vi "Labview.vi"() -> ()   [LabVIEW 2021]
uses:
  <vilib>/userdefined/High Color/IMAQdx.ctl
  <vilib>/Instr/_visa.llb/VISA Configure Serial Port (Instr).vi
  <vilib>/Utility/cursorutil.llb/Set Cursor (Icon Pict).vi
  <vilib>/Utility/file.llb/Write Delimited Spreadsheet (string).vi
  <vilib>/addons/VIRobotics/onnx/Session/Get_Result_float.vi
  <vilib>/vision/driver/NI_Vision_Acquisition_Software.lvlib
  <vilib>/vision/NI_Vision_Development_Module.lvlib
  <vilib>/addons/VIRobotics/onnx/Session/Session.lvclass
panel:
  out "String 2":string
  out "Tab Control":T1(tab)
  in  "Ga2 6":string="908"
  out "Sub1 3":string
  out "MSE loss":string
  in  "Is the probability of the model output deoxidization exceeding":bool
  out "Obtain Growth Temperature":bool
  out "From (2×4) to (n×6)":string
  out "From c(4×4) to (2×4)":string
  out "From As cap to c(4×4)":string
  out "Substrate to find Reconstruction temperature":string
  out "Cool to less than 100 ℃ and wait 20 minutes":bool
  out "GaAs buffer 0.6 μm/h":bool
  in  "nm 3":u32=100
  in  "Ga2 5":string="908"
  out "Sub1 2":string
  out "Heating to completely remove oxidation":bool
  out "Deoxidation temperature":string
  out "Substrate to find Deoxidation temperature":string
  out "Obtaining the reconstruction  temperature":bool
  out "Obtaining the deoxidation temperature":bool
  in  "Start":bool
  in  "Ga2 1":string="908"
  out "Ready for GaAs buffer 0.6 μm/h":bool
  out "GaAs buffer 0.6 μm/h":bool
  out "Sub1":string
  in  "nm":u32=100
  out "Reconstruction模型输出结果":string
  out "InAs growth temperature":string
  out "GaAs growth temperature":string
  out "C =":string
  out "B =":string
  out "A =":string
  in  "Is the probability of the model output c(4×4) exceeding":bool
  in  "Is the probability of the model output (2×4) exceeding":bool
  in  "Is the probability of the model output (n×6) exceeding":bool
  out "Surface InAs QDs for AFM":bool
  out "If In Shutter can be closed 1":bool
  out "Inside InAs QDs":bool
  out "10 nm GaAs cap layer 0.36 μm/h":bool
  out "GaAs buffer 0.6 μm/h  2":bool
  in  "Surface InAs QDs":bool=TRUE
  in  "Cooling":bool=TRUE
  in  "Sub5":string="150"
  out "Sub2":string
  in  "Ga2 2":string="888"
  out "Sub3":string
  in  "Ga2 3":string="908"
  out "Sub4":string
  in  "Ga2 4":string="800"
  out "Temperature adjustment 1":bool
  out "Temperature adjustment 2":bool
  out "Temperature adjustment 3":bool
  out "Optimize Sub Temperature 1":string
  out "Optimize Sub Temperature 2":string
  out "If In Shutter can be closed 2":bool
  in  "nm 2":u32=100
  out "Shutter模型输出结果":string
  out "Temperature模型输出结果 2":string
  in  "模型输出是否超过0.7概率是Ys":bool
  in  "Tab Control 3":enum32{"RHEED", "Array1", "Array2"}(tab)
  out "主界面 1":T2(plugin-control)
  in  "摄像头选择":T3 caption="摄像头开关"
  in  "摄像头开关":bool
  out "Countdow":u16
  out "Reminder Information":string
  in  "Model switch":bool
  in  "Whether to continue heat up for reconstruction":bool
  in  "While loop for cool to less than 100 ℃":bool
  in  "Is the probability of the model output oxidization exceeding":bool
  out "2 (2×4) count":u8
  out "5 (n×6) count":i32
  out "1 c(4×4) count":i32
  out "3 Oxidization count":u8
  out "4 Deoxidization count":u8
  out "0 As cap count":u8
  out "2 (2×4) number":u8
  out "5 (n×6) number":i32
  out "1 c(4×4) number":i32
  out "3 Oxidization number":u8
  out "4 Deoxidization number":u8
  out "0 As cap number":u8
  out "Reconstruction模型输出结果":sgl[](array[numeric])
  out "记录Reconstruction模型的连续24个输出结果":u8[](array[numeric])
  in  "T":i32=24
  in  "repetition 1 LT-GaAs not do":bool
  in  "10 nm LT-GaAs switch Yes is do":bool=TRUE
  out "Shutter count Yes":u8
  out "Shutter count No":u8
  out "Growth Switch":i32
  out "多张图片拼接后的多维数组":dbl[][][](array[numeric])
  out "用于存储单站图片转换后的单通道矩阵":dbl[][](array[numeric])
  out "经过python转换后的数组":dbl[][][][](array[numeric])
  out "error out 6":errorcluster
  in  "选择多少张图片（通道）":i32=24
  in  "转换给模型的像素长宽大小":i32=128
  out "记录Shutter模型的连续24个输出结果":u8[](array[numeric])
  out "0 Growth真空度（字符串）":string
  out "0 Buffer真空度(字符串)":string
  out "Temperature Switch":i32
  out "Shutter模型输出结果 2":sgl[](array[numeric])
  out "Temperature模型输出结果":sgl[](array[numeric])
  out "记录Temperature模型的连续24个输出结果":u8[](array[numeric])
  out "倒计时开关":bool
  out "Temperature count High":u8
  out "Temperature count Low":u8
  out "Temperature count Suitable":u8
  out "Temperature count result":u8
  out "Shutter count Yes result":u8
  in  "Yes prop":dbl=0.7 format="%#_13g"
  in  "Tetragon":cluster{"x":sgl, "y":sgl}[](array[cluster])=[{"x"=659.0, "y"=217.0}, {"x"=1148.0, "y"=217.0}, {"x"=1148.0, "y"=706.0}, {"x"=659.0, "y"=706.0}]
  in  "dimension size":i32=24
  in  "Suitable prop":dbl=0.4 format="%#_13g"
  in  "repeats of InAs/GaAs":i32=1
  in  "Is the probability of the model output As cap exceeding":bool
  in  "Reconstruction probability":dbl=0.8 format="%#_13g"
  in  "Repetition":i32
  in  "Whether to continue heating up operation":bool
  out "主界面 2":T2(plugin-control)
  in  "?":enum32{"Status"}(tab)
  out "Sub程序":string
  in  "Sub速度":string="10"
  in  "Sub设定":string="150" caption="0 Sub设定"
  out "Sub实测":string
  out "Buffer vacuum":dbl format="%.2e"
  out "Growth vacuum":dbl format="%.2e"
  in  "As挡板":bool=TRUE
  in  "In挡板":bool
  in  "Ga2挡板":bool
  in  "Main挡板":bool=TRUE
  out "Ga2实测":string
  in  "Ga2设定":string="400" caption="0 Sub设定"
  in  "Ga2速度":string="6"
  out "Ga2程序":string
  out "In实测":string
  in  "In设定":string="350" caption="0 Sub设定"
  in  "In速度":string="6"
  out "In程序":string
  # "Sub"
  # "Deoxidation temperature"
  # "Sub"
  # "Ga2"
  # "nm"
  # "Sub"
  # "Ga2"
  # "Sub"
  # "From As cap to c(4×4)"
  # "From c(4×4) to (2×4)"
  # "From (2×4) to (n×6)"
  # "Ax^2 + bx + c = 0"
  # "Sub"
  # "Ga2"
  # "nm"
  # "Sub"
  # "Ga2"
  # "Sub"
  # "Ga2"
  # "nm"
  # "Sub"
  # "Ga2"
  # "Sub"
  # "Measured temperature"
  # "Programmed\ntemperature"
  # "Setting\n(℃)"
  # "Rate\n(℃/min)"
  # "Shutter"
  # "Sub"
  # "Ga2"
  # "In"
  # "As"
  # "The As cracker’s needle valve is adjusted manually"
types:
  T1 = enum32{"Growth Temperature Initialization", "InAs/GaAs QDs on GaAs substrates"}
  T2 = typedef "IMAQ Image.ctl" = refnum<image>
  T3 = typedef "IMAQdx.ctl" = refnum<k21>
  T4 = enum8{"Enabled", "Disabled", "Disabled and Grayed Out"}
  T5 = typedef "Image Type" = u32
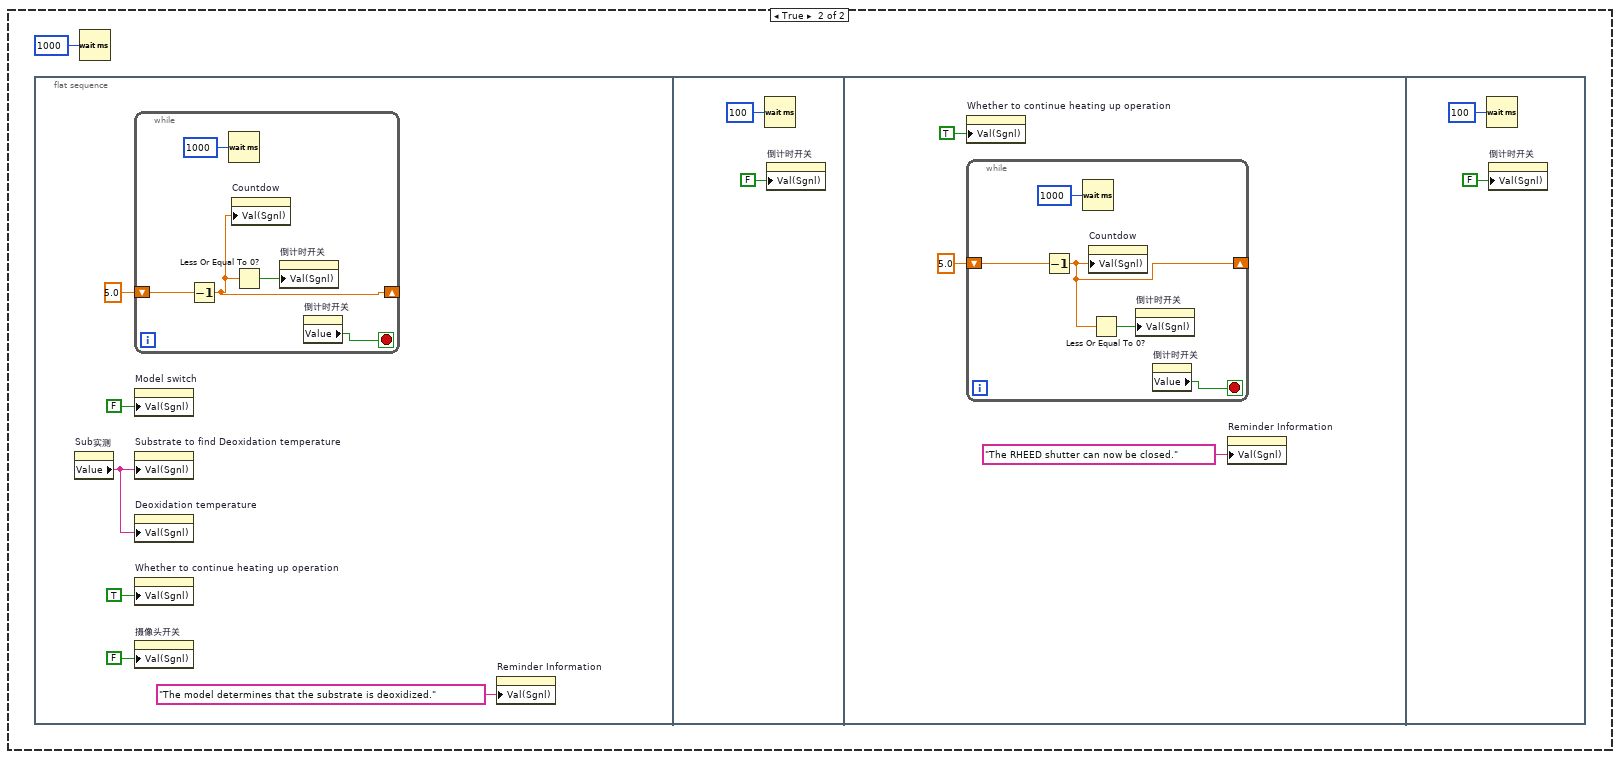
[diagram p4: hidden frame]
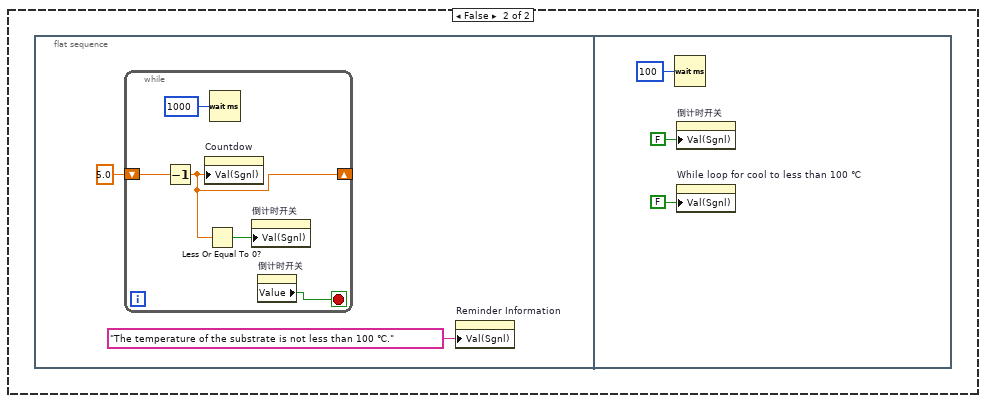
[diagram p6: hidden frame]
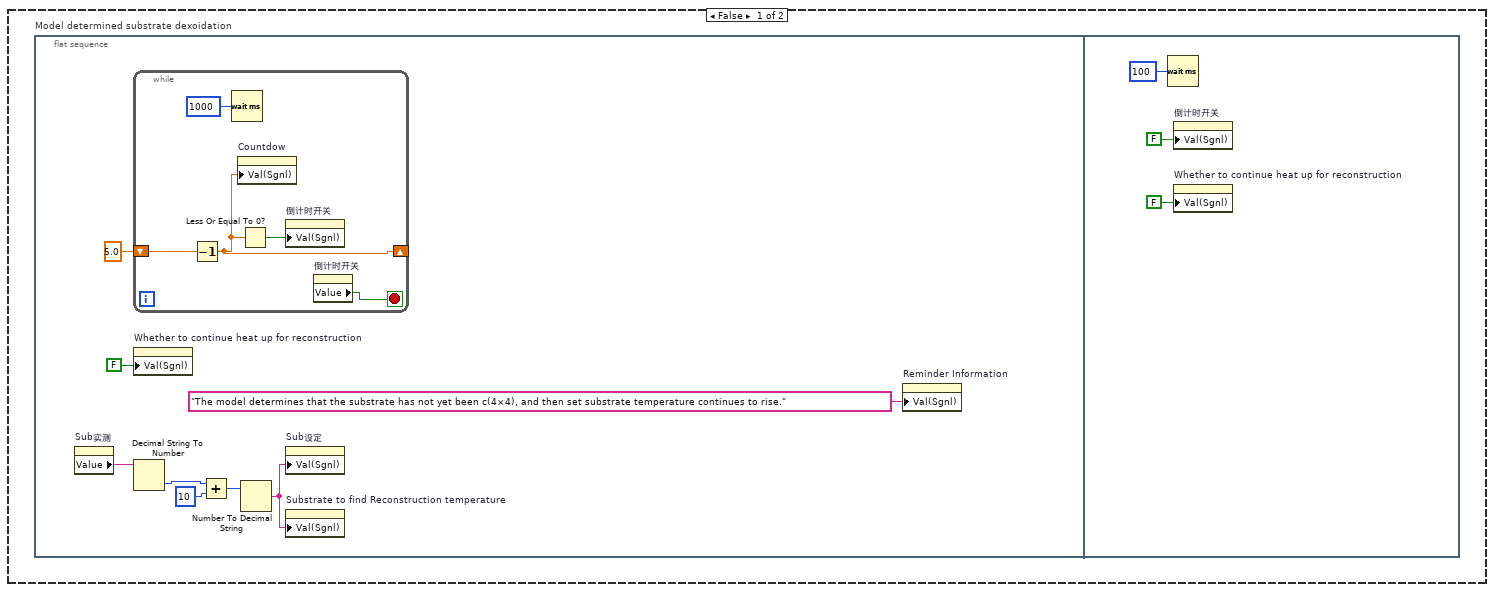
[diagram p9: hidden frame]
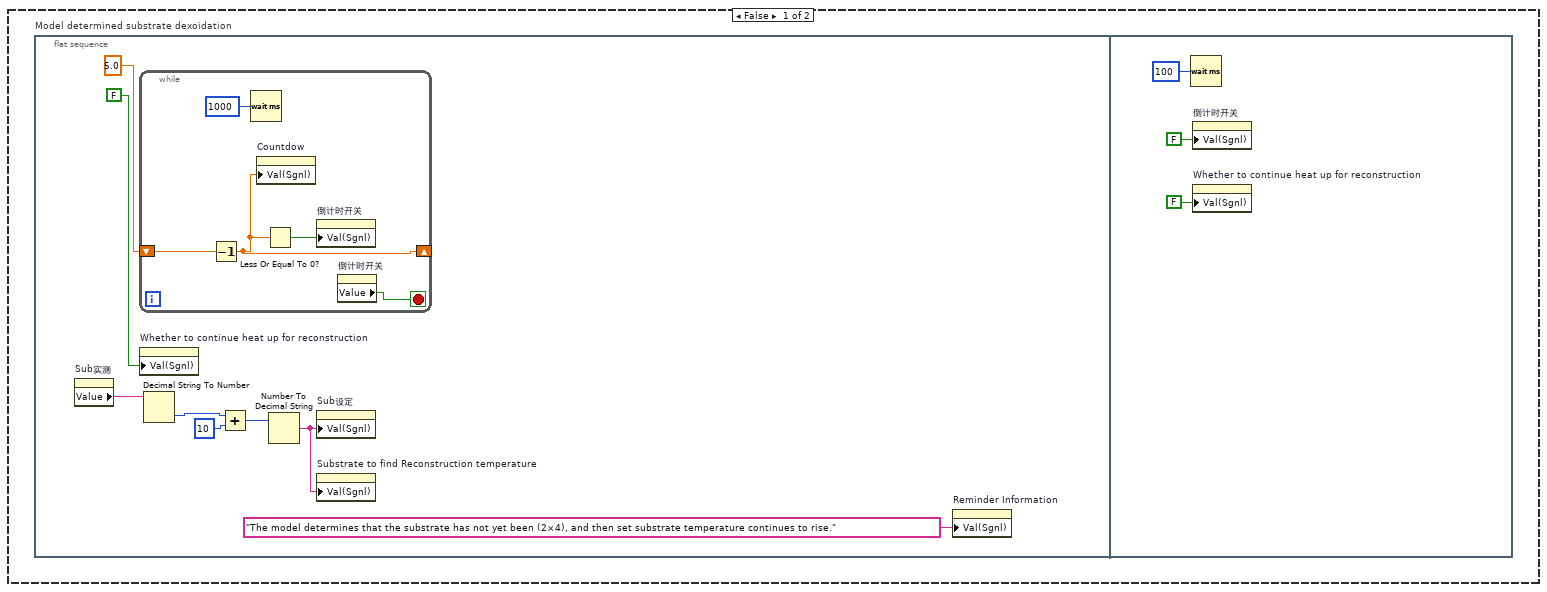
[diagram p11: hidden frame]
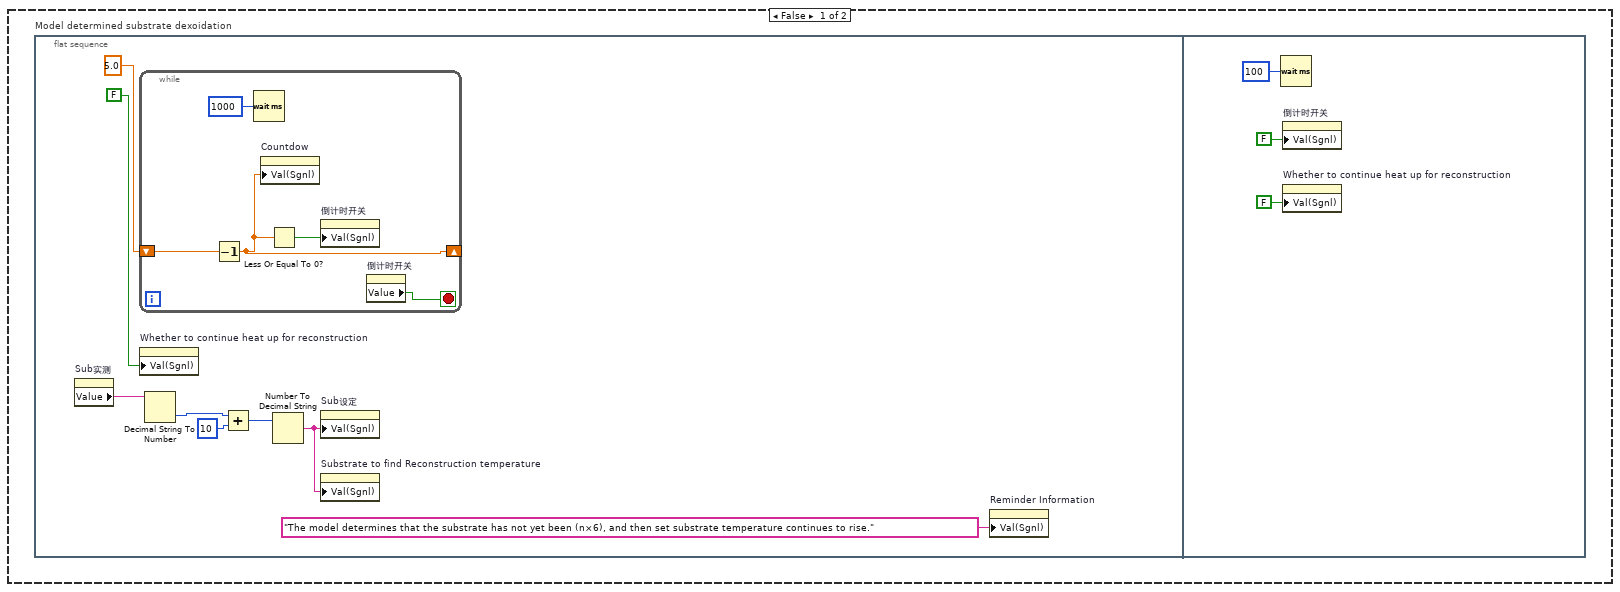
[diagram p13: hidden frame]
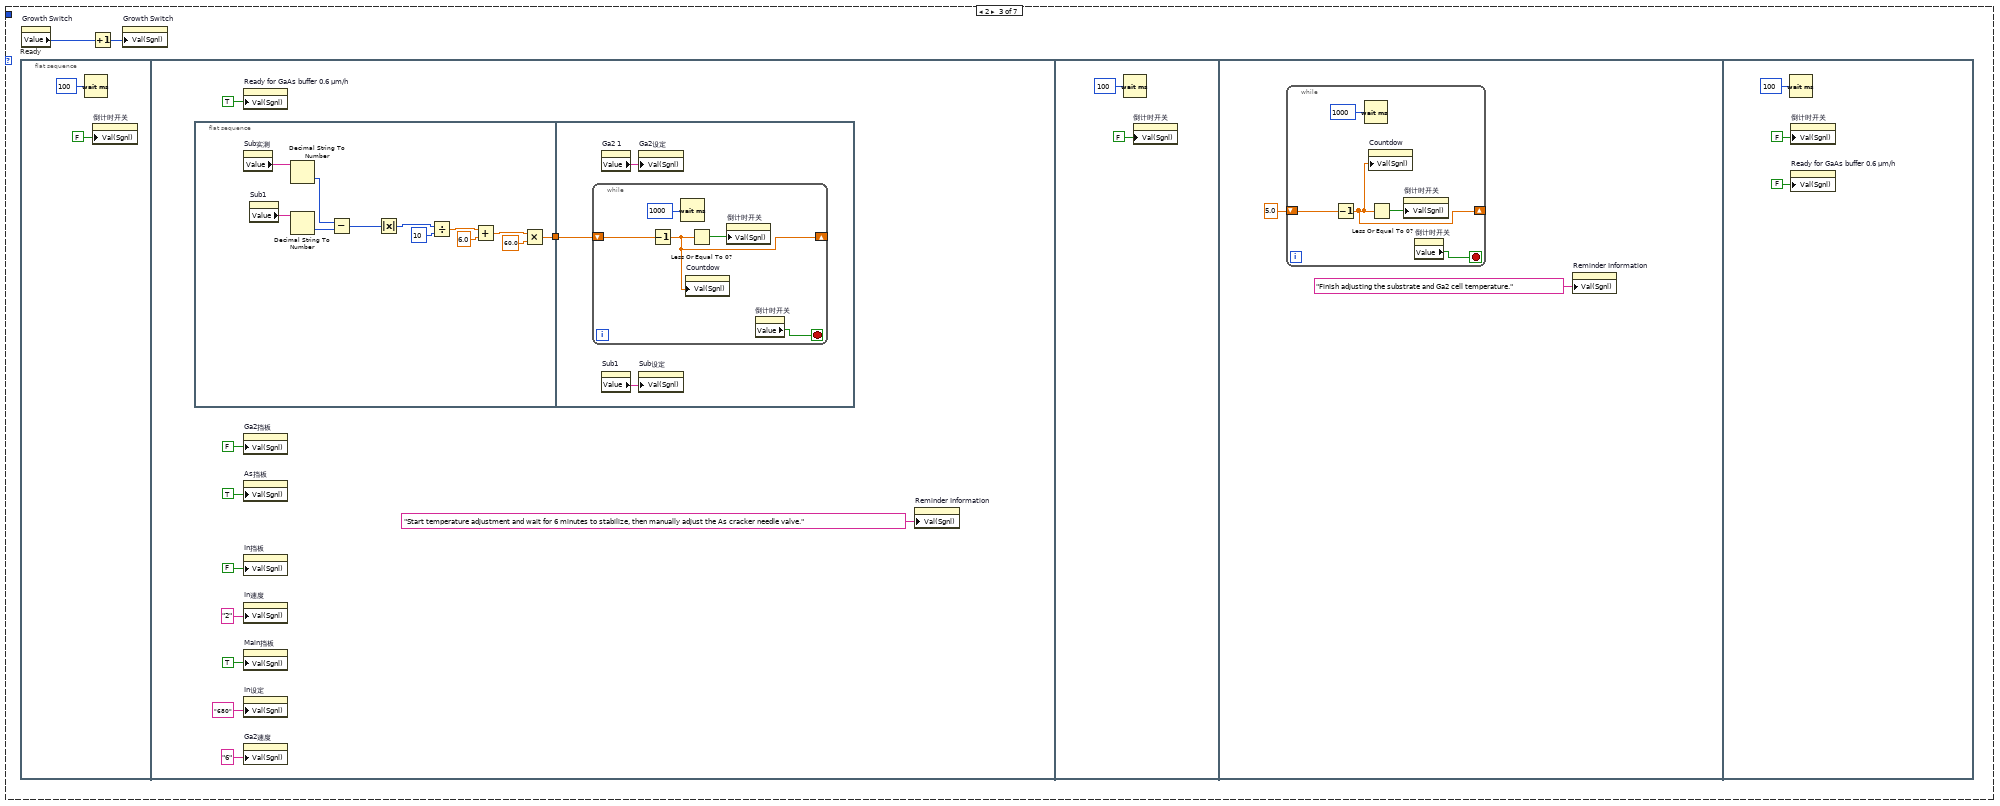
[diagram p15: hidden frame]
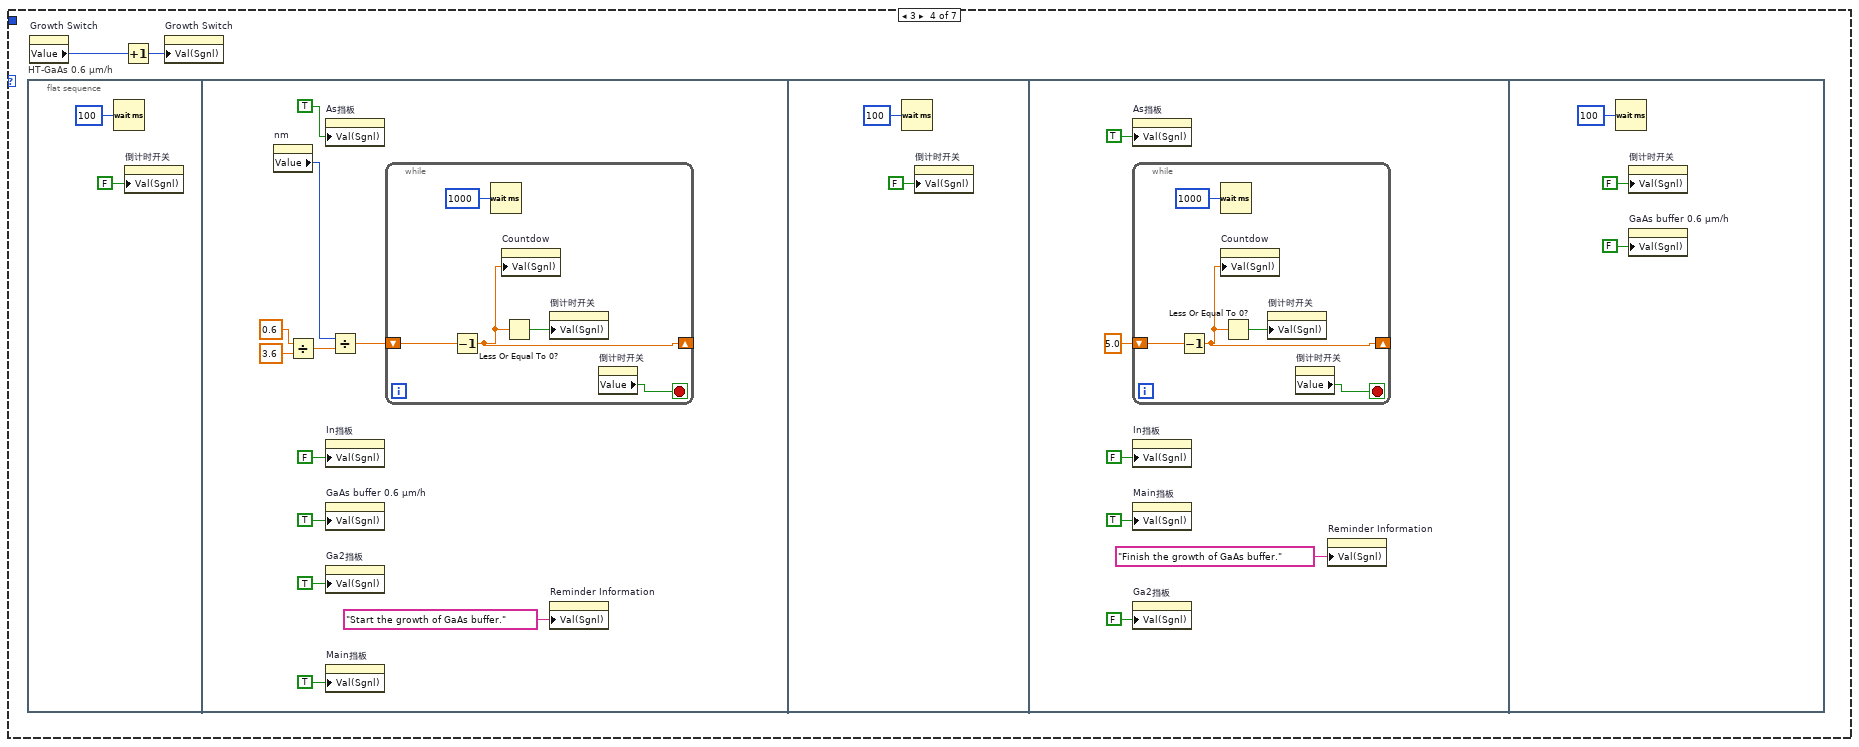
[diagram p16: hidden frame]
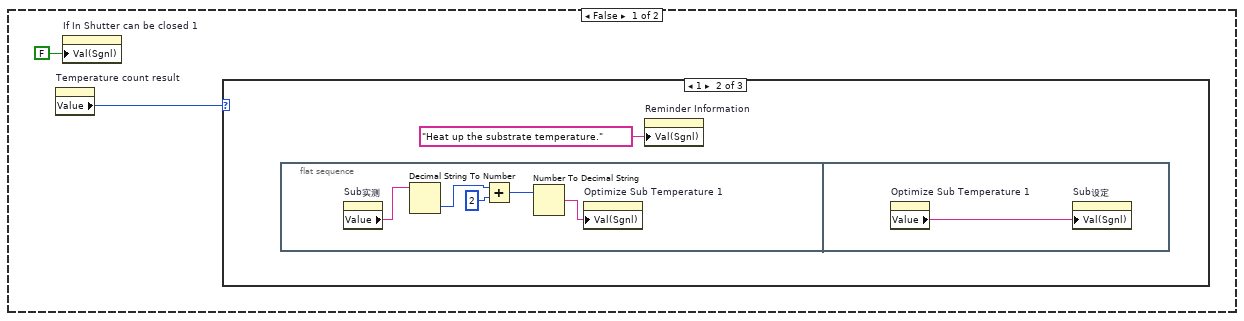
[diagram p17: hidden frame]
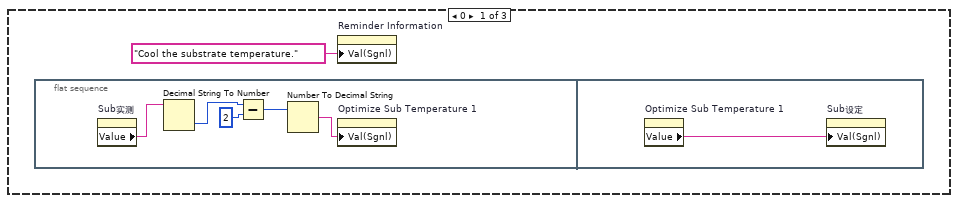
[diagram p18: hidden frame]
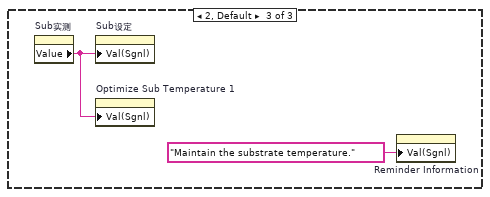
[diagram p19: hidden frame]
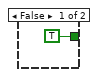
[diagram p20: hidden frame]
diagram:
  w71 = u16 10 items=["1.0"=10, "1.5"=15, "2.0"=20] ("stop bits (10: 1 bit)")
  w82 = u16 20 items=["1.0"=10, "1.5"=15, "2.0"=20] ("stop bits (10: 1 bit)")
  n1 = while {
    stop <- FALSE stop-if-true
    w91 = refnum<visa-resource-name> "COM9"  # Temperature I/O
    n2 = property on="Temperature Switch" class="DigNum (strict)"() -> ("Value"=w92:i32)  [unwired: 2 in, 2 out]
    n3 = case shown="1" w92 {
      tunnel: w91 -> [w97 w111 w124]
      frame 1 {
        n4 = flat-sequence {
          tunnel: w97 -> [w101]
          tunnel: [w101] -> w96
          tunnel: w96 -> [w103]
          tunnel: [w103] -> w95
          tunnel: w95 -> [w105]
          tunnel: [w105] -> w94
          tunnel: w94 -> [w107]
          frame #0 {
            n5 = call "Ga R.vi"("VISA resource name"=w101) -> ("程序温度"=w100:string)  [unwired: 10 in]
            n6 = property on="Ga2程序" class="Str"("Val(Sgnl)"=w100) -> ()  [unwired: 2 in, 2 out]
          }
          frame #1 {
            n7 = call "Ga P.vi"("VISA resource name"=w103) -> ("实测温度"=w102:string)  [unwired: 10 in]
            n8 = property on="Ga2实测" class="Str"("Val(Sgnl)"=w102) -> ()  [unwired: 2 in, 2 out]
          }
          frame #2 {
            n9 = property on="Ga2设定" class="Str"() -> ("Value"=w104:string)  [unwired: 2 in, 2 out]
            n10 = call "Ga S.vi"("VISA resource name 2"=w105, "设定温度"=w104) -> ()  [unwired: 10 in]
          }
          frame #3 {
            n11 = property on="Ga2速度" class="Str"() -> ("Value"=w106:string)  [unwired: 2 in, 2 out]
            n12 = call "Ga V.vi"("VISA resource name"=w107, "升温速度"=w106) -> ()  [unwired: 10 in]
          }
        }
        n13 = property on="Temperature Switch" class="DigNum (strict)"() -> ("Value"=w98:i32)  [unwired: 2 in, 2 out]
        n14 = Increment(x=w98) -> (x+1=w99:i32)
        n15 = property on="Temperature Switch" class="DigNum (strict)"("Val(Sgnl)"=w99) -> ()  [unwired: 2 in, 2 out]
      }
      frame 2 {
        n16 = flat-sequence {
          tunnel: w111 -> [w114]
          tunnel: [w114] -> w110
          tunnel: w110 -> [w116]
          tunnel: [w116] -> w109
          tunnel: w109 -> [w118]
          tunnel: [w118] -> w108
          tunnel: w108 -> [w120]
          frame #0 {
            n17 = call "In R.vi"("VISA resource name"=w114) -> ("程序温度"=w113:string)  [unwired: 10 in]
            n18 = property on="In程序" class="Str"("Val(Sgnl)"=w113) -> ()  [unwired: 2 in, 2 out]
          }
          frame #1 {
            n19 = call "In P.vi"("VISA resource name"=w116) -> ("实测温度"=w115:string)  [unwired: 10 in]
            n20 = property on="In实测" class="Str"("Val(Sgnl)"=w115) -> ()  [unwired: 2 in, 2 out]
          }
          frame #2 {
            n21 = property on="In设定" class="Str"() -> ("Value"=w117:string)  [unwired: 2 in, 2 out]
            n22 = call "In S.vi"("VISA resource name 2"=w118, "设定温度"=w117) -> ()  [unwired: 10 in]
          }
          frame #3 {
            n23 = property on="In速度" class="Str"() -> ("Value"=w119:string)  [unwired: 2 in, 2 out]
            n24 = call "In V.vi"("VISA resource name"=w120, "升温速度"=w119) -> ()  [unwired: 10 in]
          }
        }
        n25 = property on="Temperature Switch" class="DigNum (strict)"("Val(Sgnl)"=0 ("Value (Signaling)")) -> ()  [unwired: 2 in, 2 out]
      }
      frame 0, Default {
        n26 = flat-sequence {
          tunnel: w124 -> [w128]
          tunnel: [w128] -> w123
          tunnel: w123 -> [w130]
          tunnel: [w130] -> w122
          tunnel: w122 -> [w131]
          tunnel: [w131] -> w121
          tunnel: w121 -> [w133]
          frame #0 {
            n27 = call "Sub R.vi"("VISA resource name"=w128) -> ("程序温度"=w127:string)  [unwired: 10 in]
            n28 = property on="Sub程序" class="Str"("Val(Sgnl)"=w127) -> ()  [unwired: 2 in, 2 out]
          }
          frame #1 {
            n29 = call "Sub P.vi"("VISA resource name"=w130) -> ("实测温度"=w129:string)  [unwired: 10 in]
            n30 = property on="Sub实测" class="Str"("Val(Sgnl)"=w129) -> ()  [unwired: 2 in, 2 out]
          }
          frame #2 {
            n31 = property on="Sub设定" class="Str"() -> ("Value"=w132:string)  [unwired: 2 in, 2 out]
            n32 = call "Sub S.vi"("VISA resource name 2"=w131, "设定温度"=w132) -> ()  [unwired: 10 in]
          }
          frame #3 {
            n33 = property on="Sub速度" class="Str"() -> ("Value"=w134:string)  [unwired: 2 in, 2 out]
            n34 = call "Sub V.vi"("VISA resource name"=w133, "升温速度"=w134) -> ()  [unwired: 10 in]
          }
        }
        n35 = property on="Temperature Switch" class="DigNum (strict)"() -> ("Value"=w125:i32)  [unwired: 2 in, 2 out]
        n36 = Increment(x=w125) -> (x+1=w126:i32)
        n37 = property on="Temperature Switch" class="DigNum (strict)"("Val(Sgnl)"=w126) -> ()  [unwired: 2 in, 2 out]
      }
    }
  }
  n38 = flat-sequence {
    frame #0 {
      n39 = Wait (ms)(milliseconds to wait=u32 1000) -> ()  [unwired: 1 out]
    }
    frame #1 {
      n40 = while {
        stop <- FALSE stop-if-true
        n41 = property on="Start" class="Bool (strict)"() -> ("Value"=w136:bool)  [unwired: 2 in, 2 out]
        n42 = case shown="True" w136 {
          frame False {
          }
          frame True {
            n43 = property on="repeats of InAs/GaAs" class="DigNum (strict)"() -> ("Value"=w139:i32)  [unwired: 2 in, 2 out]
            n44 = property on="Growth Switch" class="DigNum (strict)"() -> ("Value"=w138:i32)  [unwired: 2 in, 2 out]
            n45 = case shown="4" w138 {
              tunnel: w139 -> [_ _ _ _ w802 _ _]
              frame 0, Default {
                n46 = flat-sequence {
                  frame #0 {
                    n47 = flat-sequence "Achieving the deoxidation temperature" {
                      frame #0 {
                        n48 = Wait (ms)(milliseconds to wait=u32 100) -> ()  [unwired: 1 out]
                        n49 = property on="倒计时开关" class="Bool (strict)"("Val(Sgnl)"=FALSE ("Value (Signaling)")) -> ()  [unwired: 2 in, 2 out]
                      }
                      frame #1 {
                        w145 = "390" ("Value (Signaling)")
                        n50 = property on="As挡板" class="Bool (strict)"("Val(Sgnl)"=TRUE ("Value (Signaling)")) -> ()  [unwired: 2 in, 2 out]
                        n51 = while {
                          shift-right: [w154] -> _
                          shift-left: 5.0 -> [w156]
                          stop <- w155 stop-if-true
                          n52 = Decrement(x=w156) -> (x-1=w154:dbl)
                          n53 = Wait (ms)(milliseconds to wait=u32 1000) -> ()  [unwired: 1 out]
                          n54 = property on="Countdow" class="DigNum (strict)"("Val(Sgnl)"=w154) -> ()  [unwired: 2 in, 2 out]
                          n55 = Less Or Equal To 0?(x=w154) -> (x <= 0?=w153:bool)
                          n56 = property on="倒计时开关" class="Bool (strict)"("Val(Sgnl)"=w153) -> ()  [unwired: 2 in, 2 out]
                          n57 = property on="倒计时开关" class="Bool (strict)"() -> ("Value"=w155:bool)  [unwired: 2 in, 2 out]
                        }
                        n58 = property on="Ga2挡板" class="Bool (strict)"("Val(Sgnl)"=FALSE ("Value (Signaling)")) -> ()  [unwired: 2 in, 2 out]
                        n59 = property on="Sub设定" class="Str"("Val(Sgnl)"=w145) -> ()  [unwired: 2 in, 2 out]
                        n60 = property on="Substrate to find Deoxidation temperature" class="Str"("Val(Sgnl)"=w145) -> ()  [unwired: 2 in, 2 out]
                        n61 = property on="Main挡板" class="Bool (strict)"("Val(Sgnl)"=TRUE ("Value (Signaling)")) -> ()  [unwired: 2 in, 2 out]
                        n62 = property on="Obtaining the deoxidation temperature" class="Bool (strict)"("Val(Sgnl)"=TRUE ("Value (Signaling)")) -> ()  [unwired: 2 in, 2 out]
                        n63 = property on="In挡板" class="Bool (strict)"("Val(Sgnl)"=FALSE ("Value (Signaling)")) -> ()  [unwired: 2 in, 2 out]
                        n64 = property on="Reminder Information" class="Str"("Val(Sgnl)"="Start to obtain the deoxidation temperature." ("Value (Signaling)")) -> ()  [unwired: 2 in, 2 out]
                      }
                      frame #2 {
                        n65 = Wait (ms)(milliseconds to wait=u32 100) -> ()  [unwired: 1 out]
                        n66 = property on="倒计时开关" class="Bool (strict)"("Val(Sgnl)"=FALSE ("Value (Signaling)")) -> ()  [unwired: 2 in, 2 out]
                      }
                      frame #3 {
                        n67 = flat-sequence {
                          tunnel: [w162] -> w161
                          tunnel: w161 -> [w174]
                          frame #0 {
                            n68 = property on="Sub实测" class="Str"() -> ("Value"=w172:string)  [unwired: 2 in, 2 out]
                            n69 = property on="Sub设定" class="Str"() -> ("Value"=w163:string)  [unwired: 2 in, 2 out]
                            n70 = Decimal String To Number(string=w172) -> (number=w173:i32)  [unwired: 2 in, 1 out]
                            n71 = Decimal String To Number(string=w163) -> (number=w170:i32)  [unwired: 2 in, 1 out]
                            n72 = Subtract(x=w173, y=w170) -> (x-y=w171:i32)
                            n73 = Absolute Value(x=w171) -> (abs(x)=w169:i32)
                            n74 = Divide(x=w169, y=10) -> (x/y=w168:dbl)
                            n75 = Add(x=w168, y=6.0) -> (x+y=w167:dbl)
                            n76 = Multiply(x=w167, y=60.0) -> (x*y=w162:dbl)
                          }
                          frame #1 {
                            n77 = while {
                              shift-right: [w176] -> _
                              shift-left: w174 -> [w179]
                              stop <- w178 stop-if-true
                              n78 = Decrement(x=w179) -> (x-1=w176:dbl)
                              n79 = Wait (ms)(milliseconds to wait=u32 1000) -> ()  [unwired: 1 out]
                              n80 = property on="Countdow" class="DigNum (strict)"("Val(Sgnl)"=w176) -> ()  [unwired: 2 in, 2 out]
                              n81 = Less Or Equal?(x=w176, y=90.0) -> (x <= y?=w175:bool)
                              n82 = property on="倒计时开关" class="Bool (strict)"("Val(Sgnl)"=w175) -> ()  [unwired: 2 in, 2 out]
                              n83 = property on="倒计时开关" class="Bool (strict)"() -> ("Value"=w178:bool)  [unwired: 2 in, 2 out]
                            }
                          }
                        }
                        n84 = property on="Reminder Information" class="Str"("Val(Sgnl)"="Start temperature adjustment and wait for 6 minutes to stabilize." ("Value (Signaling)")) -> ()  [unwired: 2 in, 2 out]
                      }
                      frame #4 {
                        n85 = property on="倒计时开关" class="Bool (strict)"("Val(Sgnl)"=FALSE ("Value (Signaling)")) -> ()  [unwired: 2 in, 2 out]
                      }
                      frame #5 {
                        n86 = property on="摄像头开关" class="Bool (strict)"("Val(Sgnl)"=TRUE ("Value (Signaling)")) -> ()  [unwired: 2 in, 2 out]
                        n87 = while {
                          shift-right: [w186] -> _
                          shift-left: 90.0 -> [w189]
                          stop <- w188 stop-if-true
                          n88 = Decrement(x=w189) -> (x-1=w186:dbl)
                          n89 = property on="Countdow" class="DigNum (strict)"("Val(Sgnl)"=w186) -> ()  [unwired: 2 in, 2 out]
                          n90 = Wait (ms)(milliseconds to wait=u32 1000) -> ()  [unwired: 1 out]
                          n91 = Less Or Equal?(x=w186, y=15.0) -> (x <= y?=w187:bool)
                          n92 = property on="倒计时开关" class="Bool (strict)"("Val(Sgnl)"=w187) -> ()  [unwired: 2 in, 2 out]
                          n93 = property on="倒计时开关" class="Bool (strict)"() -> ("Value"=w188:bool)  [unwired: 2 in, 2 out]
                        }
                        n94 = property on="Reminder Information" class="Str"("Val(Sgnl)"="There are 90 seconds left, please open the RHEED shutter manually." ("Value (Signaling)")) -> ()  [unwired: 2 in, 2 out]
                      }
                      frame #6 {
                        n95 = Wait (ms)(milliseconds to wait=u32 100) -> ()  [unwired: 1 out]
                        n96 = property on="倒计时开关" class="Bool (strict)"("Val(Sgnl)"=FALSE ("Value (Signaling)")) -> ()  [unwired: 2 in, 2 out]
                      }
                      frame #7 {
                        n97 = property on="Model switch" class="Bool (strict)"("Val(Sgnl)"=TRUE ("Value (Signaling)")) -> ()  [unwired: 2 in, 2 out]
                        n98 = while {
                          shift-right: [w195] -> _
                          shift-left: 15.0 -> [w198]
                          stop <- w197 stop-if-true
                          n99 = Decrement(x=w198) -> (x-1=w195:dbl)
                          n100 = Wait (ms)(milliseconds to wait=u32 1000) -> ()  [unwired: 1 out]
                          n101 = property on="Countdow" class="DigNum (strict)"("Val(Sgnl)"=w195) -> ()  [unwired: 2 in, 2 out]
                          n102 = Less Or Equal To 0?(x=w195) -> (x <= 0?=w196:bool)
                          n103 = property on="倒计时开关" class="Bool (strict)"("Val(Sgnl)"=w196) -> ()  [unwired: 2 in, 2 out]
                          n104 = property on="倒计时开关" class="Bool (strict)"() -> ("Value"=w197:bool)  [unwired: 2 in, 2 out]
                        }
                      }
                      frame #8 {
                        n105 = Wait (ms)(milliseconds to wait=u32 100) -> ()  [unwired: 1 out]
                        n106 = property on="倒计时开关" class="Bool (strict)"("Val(Sgnl)"=FALSE ("Value (Signaling)")) -> ()  [unwired: 2 in, 2 out]
                      }
                      frame #9 {
                        n107 = while {
                          stop <- w204 stop-if-true
                          n108 = property on="Is the probability of the model output deoxidization exceeding" class="Bool (strict)"() -> ("Value"=w202:bool)  [unwired: 2 in, 2 out]
                          n109 = property on="Whether to continue heating up operation" class="Bool (strict)"() -> ("Value"=w203:bool)  [unwired: 2 in, 2 out]
                          n110 = case shown="False" w203 {
                            tunnel: w202 -> [w205 _]
                            frame False {
                              n111 = case shown="False" w205 {
                                frame False {
                                n112 = flat-sequence "Model determined substrate dexoidation" {
                                frame #0 {
                                n113 = property on="Sub实测" class="Str"() -> ("Value"=w210:string)  [unwired: 2 in, 2 out]
                                n114 = property on="摄像头开关" class="Bool (strict)"("Val(Sgnl)"=FALSE ("Value (Signaling)")) -> ()  [unwired: 2 in, 2 out]
                                n115 = property on="Whether to continue heating up operation" class="Bool (strict)"("Val(Sgnl)"=FALSE ("Value (Signaling)")) -> ()  [unwired: 2 in, 2 out]
                                n116 = property on="Model switch" class="Bool (strict)"("Val(Sgnl)"=FALSE ("Value (Signaling)")) -> ()  [unwired: 2 in, 2 out]
                                n117 = while {
                                shift-right: [w216] -> _
                                shift-left: 5.0 -> [w219]
                                stop <- w218 stop-if-true
                                n118 = Decrement(x=w219) -> (x-1=w216:dbl)
                                n119 = Wait (ms)(milliseconds to wait=u32 1000) -> ()  [unwired: 1 out]
                                n120 = property on="Countdow" class="DigNum (strict)"("Val(Sgnl)"=w216) -> ()  [unwired: 2 in, 2 out]
                                n121 = Less Or Equal To 0?(x=w216) -> (x <= 0?=w217:bool)
                                n122 = property on="倒计时开关" class="Bool (strict)"("Val(Sgnl)"=w217) -> ()  [unwired: 2 in, 2 out]
                                n123 = property on="倒计时开关" class="Bool (strict)"() -> ("Value"=w218:bool)  [unwired: 2 in, 2 out]
                                }
                                n124 = Decimal String To Number(string=w210) -> (number=w212:i32)  [unwired: 2 in, 1 out]
                                n125 = Add(x=w212, y=5) -> (x+y=w213:i32)
                                n126 = Number To Decimal String(number=w213) -> (decimal integer string=w209:string)  [unwired: 1 in]
                                n127 = property on="Substrate to find Deoxidation temperature" class="Str"("Val(Sgnl)"=w209) -> ()  [unwired: 2 in, 2 out]
                                n128 = property on="Sub设定" class="Str"("Val(Sgnl)"=w209) -> ()  [unwired: 2 in, 2 out]
                                n129 = property on="Reminder Information" class="Str"("Val(Sgnl)"="The model determines that the substrate has not yet been deoxidized, and the set substrate temperature continues to rise." ("Value (Signaling)")) -> ()  [unwired: 2 in, 2 out]
                                }
                                frame #1 {
                                n130 = Wait (ms)(milliseconds to wait=u32 100) -> ()  [unwired: 1 out]
                                n131 = property on="倒计时开关" class="Bool (strict)"("Val(Sgnl)"=FALSE ("Value (Signaling)")) -> ()  [unwired: 2 in, 2 out]
                                }
                                frame #2 {
                                n132 = while {
                                shift-right: [w225] -> _
                                shift-left: 5.0 -> [w228]
                                stop <- w227 stop-if-true
                                n133 = Decrement(x=w228) -> (x-1=w225:dbl)
                                n134 = Wait (ms)(milliseconds to wait=u32 1000) -> ()  [unwired: 1 out]
                                n135 = property on="Countdow" class="DigNum (strict)"("Val(Sgnl)"=w225) -> ()  [unwired: 2 in, 2 out]
                                n136 = Less Or Equal To 0?(x=w225) -> (x <= 0?=w226:bool)
                                n137 = property on="倒计时开关" class="Bool (strict)"("Val(Sgnl)"=w226) -> ()  [unwired: 2 in, 2 out]
                                n138 = property on="倒计时开关" class="Bool (strict)"() -> ("Value"=w227:bool)  [unwired: 2 in, 2 out]
                                }
                                n139 = property on="Reminder Information" class="Str"("Val(Sgnl)"="The RHEED shutter can now be closed." ("Value (Signaling)")) -> ()  [unwired: 2 in, 2 out]
                                }
                                frame #3 {
                                n140 = Wait (ms)(milliseconds to wait=u32 100) -> ()  [unwired: 1 out]
                                n141 = property on="倒计时开关" class="Bool (strict)"("Val(Sgnl)"=FALSE ("Value (Signaling)")) -> ()  [unwired: 2 in, 2 out]
                                }
                                frame #4 {
                                n142 = flat-sequence {
                                tunnel: [w234] -> w232
                                tunnel: w232 -> [w246]
                                frame #0 {
                                n143 = property on="Sub实测" class="Str"() -> ("Value"=w244:string)  [unwired: 2 in, 2 out]
                                n144 = property on="Sub设定" class="Str"() -> ("Value"=w235:string)  [unwired: 2 in, 2 out]
                                n145 = Decimal String To Number(string=w244) -> (number=w245:i32)  [unwired: 2 in, 1 out]
                                n146 = Decimal String To Number(string=w235) -> (number=w242:i32)  [unwired: 2 in, 1 out]
                                n147 = Subtract(x=w245, y=w242) -> (x-y=w243:i32)
                                n148 = Absolute Value(x=w243) -> (abs(x)=w241:i32)
                                n149 = Divide(x=w241, y=10) -> (x/y=w240:dbl)
                                n150 = Add(x=w240, y=6.0) -> (x+y=w239:dbl)
                                n151 = Multiply(x=w239, y=60.0) -> (x*y=w234:dbl)
                                }
                                frame #1 {
                                n152 = while {
                                shift-right: [w248] -> _
                                shift-left: w246 -> [w251]
                                stop <- w250 stop-if-true
                                n153 = Decrement(x=w251) -> (x-1=w248:dbl)
                                n154 = property on="Countdow" class="DigNum (strict)"("Val(Sgnl)"=w248) -> ()  [unwired: 2 in, 2 out]
                                n155 = Wait (ms)(milliseconds to wait=u32 1000) -> ()  [unwired: 1 out]
                                n156 = Less Or Equal?(x=w248, y=90.0) -> (x <= y?=w247:bool)
                                n157 = property on="倒计时开关" class="Bool (strict)"("Val(Sgnl)"=w247) -> ()  [unwired: 2 in, 2 out]
                                n158 = property on="倒计时开关" class="Bool (strict)"() -> ("Value"=w250:bool)  [unwired: 2 in, 2 out]
                                }
                                }
                                }
                                n159 = property on="Reminder Information" class="Str"("Val(Sgnl)"="Start temperature adjustment and wait for 6 minutes to stabilize." ("Value (Signaling)")) -> ()  [unwired: 2 in, 2 out]
                                }
                                frame #5 {
                                n160 = Wait (ms)(milliseconds to wait=u32 100) -> ()  [unwired: 1 out]
                                n161 = property on="倒计时开关" class="Bool (strict)"("Val(Sgnl)"=FALSE ("Value (Signaling)")) -> ()  [unwired: 2 in, 2 out]
                                }
                                frame #6 {
                                n162 = property on="摄像头开关" class="Bool (strict)"("Val(Sgnl)"=TRUE ("Value (Signaling)")) -> ()  [unwired: 2 in, 2 out]
                                n163 = while {
                                shift-right: [w259] -> _
                                shift-left: 90.0 -> [w262]
                                stop <- w261 stop-if-true
                                n164 = Decrement(x=w262) -> (x-1=w259:dbl)
                                n165 = property on="Countdow" class="DigNum (strict)"("Val(Sgnl)"=w259) -> ()  [unwired: 2 in, 2 out]
                                n166 = Wait (ms)(milliseconds to wait=u32 1000) -> ()  [unwired: 1 out]
                                n167 = Less Or Equal?(x=w259, y=15.0) -> (x <= y?=w260:bool)
                                n168 = property on="倒计时开关" class="Bool (strict)"("Val(Sgnl)"=w260) -> ()  [unwired: 2 in, 2 out]
                                n169 = property on="倒计时开关" class="Bool (strict)"() -> ("Value"=w261:bool)  [unwired: 2 in, 2 out]
                                }
                                n170 = property on="Reminder Information" class="Str"("Val(Sgnl)"="There are 90 seconds left, please open the RHEED shutter manually." ("Value (Signaling)")) -> ()  [unwired: 2 in, 2 out]
                                }
                                frame #7 {
                                n171 = Wait (ms)(milliseconds to wait=u32 100) -> ()  [unwired: 1 out]
                                n172 = property on="倒计时开关" class="Bool (strict)"("Val(Sgnl)"=FALSE ("Value (Signaling)")) -> ()  [unwired: 2 in, 2 out]
                                }
                                frame #8 {
                                n173 = property on="Model switch" class="Bool (strict)"("Val(Sgnl)"=TRUE ("Value (Signaling)")) -> ()  [unwired: 2 in, 2 out]
                                n174 = while {
                                shift-right: [w269] -> _
                                shift-left: 15.0 -> [w271]
                                stop <- w270 stop-if-true
                                n175 = Decrement(x=w271) -> (x-1=w269:dbl)
                                n176 = Wait (ms)(milliseconds to wait=u32 1000) -> ()  [unwired: 1 out]
                                n177 = property on="Countdow" class="DigNum (strict)"("Val(Sgnl)"=w269) -> ()  [unwired: 2 in, 2 out]
                                n178 = Less Or Equal To 0?(x=w269) -> (x <= 0?=w268:bool)
                                n179 = property on="倒计时开关" class="Bool (strict)"("Val(Sgnl)"=w268) -> ()  [unwired: 2 in, 2 out]
                                n180 = property on="倒计时开关" class="Bool (strict)"() -> ("Value"=w270:bool)  [unwired: 2 in, 2 out]
                                }
                                }
                                frame #9 {
                                n181 = property on="Whether to continue heating up operation" class="Bool (strict)"("Val(Sgnl)"=FALSE ("Value (Signaling)")) -> ()  [unwired: 2 in, 2 out]
                                }
                                }
                                }
                                frame True {
                                n182 = flat-sequence {
                                frame #0 {
                                n183 = property on="Sub实测" class="Str"() -> ("Value"=w278:string)  [unwired: 2 in, 2 out]
                                n184 = while {
                                shift-right: [w282] -> _
                                shift-left: 5.0 -> [w284]
                                stop <- w283 stop-if-true
                                n185 = Decrement(x=w284) -> (x-1=w282:dbl)
                                n186 = Wait (ms)(milliseconds to wait=u32 1000) -> ()  [unwired: 1 out]
                                n187 = property on="Countdow" class="DigNum (strict)"("Val(Sgnl)"=w282) -> ()  [unwired: 2 in, 2 out]
                                n188 = Less Or Equal To 0?(x=w282) -> (x <= 0?=w281:bool)
                                n189 = property on="倒计时开关" class="Bool (strict)"("Val(Sgnl)"=w281) -> ()  [unwired: 2 in, 2 out]
                                n190 = property on="倒计时开关" class="Bool (strict)"() -> ("Value"=w283:bool)  [unwired: 2 in, 2 out]
                                }
                                n191 = property on="Model switch" class="Bool (strict)"("Val(Sgnl)"=FALSE ("Value (Signaling)")) -> ()  [unwired: 2 in, 2 out]
                                n192 = property on="Substrate to find Deoxidation temperature" class="Str"("Val(Sgnl)"=w278) -> ()  [unwired: 2 in, 2 out]
                                n193 = property on="Deoxidation temperature" class="Str"("Val(Sgnl)"=w278) -> ()  [unwired: 2 in, 2 out]
                                n194 = property on="Whether to continue heating up operation" class="Bool (strict)"("Val(Sgnl)"=TRUE ("Value (Signaling)")) -> ()  [unwired: 2 in, 2 out]
                                n195 = property on="摄像头开关" class="Bool (strict)"("Val(Sgnl)"=FALSE ("Value (Signaling)")) -> ()  [unwired: 2 in, 2 out]
                                n196 = property on="Reminder Information" class="Str"("Val(Sgnl)"="The model determines that the substrate is deoxidized." ("Value (Signaling)")) -> ()  [unwired: 2 in, 2 out]
                                }
                                frame #1 {
                                n197 = Wait (ms)(milliseconds to wait=u32 100) -> ()  [unwired: 1 out]
                                n198 = property on="倒计时开关" class="Bool (strict)"("Val(Sgnl)"=FALSE ("Value (Signaling)")) -> ()  [unwired: 2 in, 2 out]
                                }
                                frame #2 {
                                n199 = property on="Whether to continue heating up operation" class="Bool (strict)"("Val(Sgnl)"=TRUE ("Value (Signaling)")) -> ()  [unwired: 2 in, 2 out]
                                n200 = while {
                                shift-right: [w291] -> _
                                shift-left: 5.0 -> [w294]
                                stop <- w293 stop-if-true
                                n201 = Decrement(x=w294) -> (x-1=w291:dbl)
                                n202 = Wait (ms)(milliseconds to wait=u32 1000) -> ()  [unwired: 1 out]
                                n203 = property on="Countdow" class="DigNum (strict)"("Val(Sgnl)"=w291) -> ()  [unwired: 2 in, 2 out]
                                n204 = Less Or Equal To 0?(x=w291) -> (x <= 0?=w292:bool)
                                n205 = property on="倒计时开关" class="Bool (strict)"("Val(Sgnl)"=w292) -> ()  [unwired: 2 in, 2 out]
                                n206 = property on="倒计时开关" class="Bool (strict)"() -> ("Value"=w293:bool)  [unwired: 2 in, 2 out]
                                }
                                n207 = property on="Reminder Information" class="Str"("Val(Sgnl)"="The RHEED shutter can now be closed." ("Value (Signaling)")) -> ()  [unwired: 2 in, 2 out]
                                }
                                frame #3 {
                                n208 = Wait (ms)(milliseconds to wait=u32 100) -> ()  [unwired: 1 out]
                                n209 = property on="倒计时开关" class="Bool (strict)"("Val(Sgnl)"=FALSE ("Value (Signaling)")) -> ()  [unwired: 2 in, 2 out]
                                }
                                }
                                n210 = Wait (ms)(milliseconds to wait=u32 1000) -> ()  [unwired: 1 out]
                                }
                              }
                            }
                            frame True {
                            }
                          }
                          n211 = property on="Whether to continue heating up operation" class="Bool (strict)"() -> ("Value"=w204:bool)  [unwired: 2 in, 2 out]
                        }
                      }
                      frame #10 {
                        n212 = Wait (ms)(milliseconds to wait=u32 100) -> ()  [unwired: 1 out]
                        n213 = property on="倒计时开关" class="Bool (strict)"("Val(Sgnl)"=FALSE ("Value (Signaling)")) -> ()  [unwired: 2 in, 2 out]
                      }
                      frame #11 {
                        n214 = property on="Obtaining the deoxidation temperature" class="Bool (strict)"("Val(Sgnl)"=FALSE ("Value (Signaling)")) -> ()  [unwired: 2 in, 2 out]
                        n215 = while {
                          shift-right: [w304] -> _
                          shift-left: 5.0 -> [w306]
                          stop <- w305 stop-if-true
                          n216 = Decrement(x=w306) -> (x-1=w304:dbl)
                          n217 = property on="Countdow" class="DigNum (strict)"("Val(Sgnl)"=w304) -> ()  [unwired: 2 in, 2 out]
                          n218 = Wait (ms)(milliseconds to wait=u32 1000) -> ()  [unwired: 1 out]
                          n219 = Less Or Equal To 0?(x=w304) -> (x <= 0?=w303:bool)
                          n220 = property on="倒计时开关" class="Bool (strict)"("Val(Sgnl)"=w303) -> ()  [unwired: 2 in, 2 out]
                          n221 = property on="倒计时开关" class="Bool (strict)"() -> ("Value"=w305:bool)  [unwired: 2 in, 2 out]
                        }
                        n222 = property on="Reminder Information" class="Str"("Val(Sgnl)"="Finish obtaining the deoxidation temperature." ("Value (Signaling)")) -> ()  [unwired: 2 in, 2 out]
                      }
                      frame #12 {
                        n223 = Wait (ms)(milliseconds to wait=u32 100) -> ()  [unwired: 1 out]
                        n224 = property on="倒计时开关" class="Bool (strict)"("Val(Sgnl)"=FALSE ("Value (Signaling)")) -> ()  [unwired: 2 in, 2 out]
                      }
                    }
                  }
                  frame #1 {
                    n225 = flat-sequence "Outgassing at about 620 ℃ for 10 minutes" {
                      frame #0 {
                        n226 = property on="Deoxidation temperature" class="Str"() -> ("Value"=w316:string)  [unwired: 2 in, 2 out]
                        n227 = Wait (ms)(milliseconds to wait=u32 100) -> ()  [unwired: 1 out]
                        n228 = property on="倒计时开关" class="Bool (strict)"("Val(Sgnl)"=FALSE ("Value (Signaling)")) -> ()  [unwired: 2 in, 2 out]
                        n229 = Decimal String To Number(string=w316) -> (number=w314:i32)  [unwired: 2 in, 1 out]
                        n230 = Divide(x=w314, y=580.0) -> (x/y=w312:dbl)
                        n231 = Multiply(x=w312, y=620.0) -> (x*y=w311:dbl)
                        n232 = Number To Decimal String(number=w311) -> (decimal integer string=w310:string)  [unwired: 1 in]
                        n233 = property on="Sub1 2" class="Str"("Val(Sgnl)"=w310) -> ()  [unwired: 2 in, 2 out]
                        n234 = property on="Sub设定" class="Str"("Val(Sgnl)"=w310) -> ()  [unwired: 2 in, 2 out]
                      }
                      frame #1 {
                        n235 = flat-sequence {
                          tunnel: [w327] -> w320
                          tunnel: w320 -> [w339]
                          frame #0 {
                            n236 = property on="Sub实测" class="Str"() -> ("Value"=w336:string)  [unwired: 2 in, 2 out]
                            n237 = property on="Sub1 2" class="Str"() -> ("Value"=w326:string)  [unwired: 2 in, 2 out]
                            n238 = Decimal String To Number(string=w336) -> (number=w337:i32)  [unwired: 2 in, 1 out]
                            n239 = Decimal String To Number(string=w326) -> (number=w334:i32)  [unwired: 2 in, 1 out]
                            n240 = Subtract(x=w337, y=w334) -> (x-y=w335:i32)
                            n241 = Absolute Value(x=w335) -> (abs(x)=w333:i32)
                            n242 = Divide(x=w333, y=10) -> (x/y=w332:dbl)
                            n243 = Add(x=w332, y=10.0) -> (x+y=w331:dbl)
                            n244 = Multiply(x=w331, y=60.0) -> (x*y=w327:dbl)
                          }
                          frame #1 {
                            n245 = while {
                              shift-right: [w340] -> _
                              shift-left: w339 -> [w343]
                              stop <- w342 stop-if-true
                              n246 = Decrement(x=w343) -> (x-1=w340:dbl)
                              n247 = property on="Countdow" class="DigNum (strict)"("Val(Sgnl)"=w340) -> ()  [unwired: 2 in, 2 out]
                              n248 = Wait (ms)(milliseconds to wait=u32 1000) -> ()  [unwired: 1 out]
                              n249 = Less Or Equal To 0?(x=w340) -> (x <= 0?=w341:bool)
                              n250 = property on="倒计时开关" class="Bool (strict)"("Val(Sgnl)"=w341) -> ()  [unwired: 2 in, 2 out]
                              n251 = property on="倒计时开关" class="Bool (strict)"() -> ("Value"=w342:bool)  [unwired: 2 in, 2 out]
                            }
                            n252 = property on="Ga2 5" class="Str"() -> ("Value"=w338:string)  [unwired: 2 in, 2 out]
                            n253 = property on="Ga2设定" class="Str"("Val(Sgnl)"=w338) -> ()  [unwired: 2 in, 2 out]
                          }
                        }
                        n254 = property on="As挡板" class="Bool (strict)"("Val(Sgnl)"=TRUE ("Value (Signaling)")) -> ()  [unwired: 2 in, 2 out]
                        n255 = property on="Ga2挡板" class="Bool (strict)"("Val(Sgnl)"=FALSE ("Value (Signaling)")) -> ()  [unwired: 2 in, 2 out]
                        n256 = property on="Main挡板" class="Bool (strict)"("Val(Sgnl)"=TRUE ("Value (Signaling)")) -> ()  [unwired: 2 in, 2 out]
                        n257 = property on="Heating to completely remove oxidation" class="Bool (strict)"("Val(Sgnl)"=TRUE ("Value (Signaling)")) -> ()  [unwired: 2 in, 2 out]
                        n258 = property on="In挡板" class="Bool (strict)"("Val(Sgnl)"=FALSE ("Value (Signaling)")) -> ()  [unwired: 2 in, 2 out]
                        n259 = property on="Reminder Information" class="Str"("Val(Sgnl)"="Heating to completely remove oxidation and waiting 10 minutes." ("Value (Signaling)")) -> ()  [unwired: 2 in, 2 out]
                      }
                      frame #2 {
                        n260 = Wait (ms)(milliseconds to wait=u32 100) -> ()  [unwired: 1 out]
                        n261 = property on="倒计时开关" class="Bool (strict)"("Val(Sgnl)"=FALSE ("Value (Signaling)")) -> ()  [unwired: 2 in, 2 out]
                      }
                      frame #3 {
                        n262 = property on="Ga2 6" class="Str"() -> ("Value"=w347:string)  [unwired: 2 in, 2 out]
                        n263 = property on="Deoxidation temperature" class="Str"() -> ("Value"=w356:string)  [unwired: 2 in, 2 out]
                        n264 = property on="Ga2设定" class="Str"("Val(Sgnl)"=w347) -> ()  [unwired: 2 in, 2 out]
                        n265 = property on="Heating to completely remove oxidation" class="Bool (strict)"("Val(Sgnl)"=FALSE ("Value (Signaling)")) -> ()  [unwired: 2 in, 2 out]
                        n266 = while {
                          shift-right: [w358] -> _
                          shift-left: 5.0 -> [w361]
                          stop <- w360 stop-if-true
                          n267 = Decrement(x=w361) -> (x-1=w358:dbl)
                          n268 = Wait (ms)(milliseconds to wait=u32 1000) -> ()  [unwired: 1 out]
                          n269 = property on="Countdow" class="DigNum (strict)"("Val(Sgnl)"=w358) -> ()  [unwired: 2 in, 2 out]
                          n270 = Less Or Equal To 0?(x=w358) -> (x <= 0?=w359:bool)
                          n271 = property on="倒计时开关" class="Bool (strict)"("Val(Sgnl)"=w359) -> ()  [unwired: 2 in, 2 out]
                          n272 = property on="倒计时开关" class="Bool (strict)"() -> ("Value"=w360:bool)  [unwired: 2 in, 2 out]
                        }
                        n273 = property on="Reminder Information" class="Str"("Val(Sgnl)"="Finish deoxidation." ("Value (Signaling)")) -> ()  [unwired: 2 in, 2 out]
                        n274 = Decimal String To Number(string=w356) -> (number=w355:i32)  [unwired: 2 in, 1 out]
                        n275 = Divide(x=w355, y=580.0) -> (x/y=w354:dbl)
                        n276 = Multiply(x=w354, y=600.0) -> (x*y=w353:dbl)
                        n277 = Number To Decimal String(number=w353) -> (decimal integer string=w348:string)  [unwired: 1 in]
                        n278 = property on="Sub1 3" class="Str"("Val(Sgnl)"=w348) -> ()  [unwired: 2 in, 2 out]
                        n279 = property on="Sub设定" class="Str"("Val(Sgnl)"=w348) -> ()  [unwired: 2 in, 2 out]
                      }
                      frame #4 {
                        n280 = Wait (ms)(milliseconds to wait=u32 100) -> ()  [unwired: 1 out]
                        n281 = property on="倒计时开关" class="Bool (strict)"("Val(Sgnl)"=FALSE ("Value (Signaling)")) -> ()  [unwired: 2 in, 2 out]
                      }
                      frame #5 {
                        n282 = flat-sequence {
                          tunnel: [w369] -> w367
                          tunnel: w367 -> [w381]
                          frame #0 {
                            n283 = property on="Sub实测" class="Str"() -> ("Value"=w378:string)  [unwired: 2 in, 2 out]
                            n284 = property on="Sub1 2" class="Str"() -> ("Value"=w368:string)  [unwired: 2 in, 2 out]
                            n285 = Decimal String To Number(string=w378) -> (number=w379:i32)  [unwired: 2 in, 1 out]
                            n286 = Decimal String To Number(string=w368) -> (number=w376:i32)  [unwired: 2 in, 1 out]
                            n287 = Subtract(x=w379, y=w376) -> (x-y=w377:i32)
                            n288 = Absolute Value(x=w377) -> (abs(x)=w375:i32)
                            n289 = Divide(x=w375, y=10) -> (x/y=w374:dbl)
                            n290 = Add(x=w374, y=3.0) -> (x+y=w373:dbl)
                            n291 = Multiply(x=w373, y=60.0) -> (x*y=w369:dbl)
                          }
                          frame #1 {
                            n292 = property on="Ga2 5" class="Str"() -> ("Value"=w380:string)  [unwired: 2 in, 2 out]
                            n293 = while {
                              shift-right: [w382] -> _
                              shift-left: w381 -> [w385]
                              stop <- w384 stop-if-true
                              n294 = Decrement(x=w385) -> (x-1=w382:dbl)
                              n295 = Wait (ms)(milliseconds to wait=u32 1000) -> ()  [unwired: 1 out]
                              n296 = property on="Countdow" class="DigNum (strict)"("Val(Sgnl)"=w382) -> ()  [unwired: 2 in, 2 out]
                              n297 = Less Or Equal To 0?(x=w382) -> (x <= 0?=w383:bool)
                              n298 = property on="倒计时开关" class="Bool (strict)"("Val(Sgnl)"=w383) -> ()  [unwired: 2 in, 2 out]
                              n299 = property on="倒计时开关" class="Bool (strict)"() -> ("Value"=w384:bool)  [unwired: 2 in, 2 out]
                            }
                            n300 = property on="Ga2设定" class="Str"("Val(Sgnl)"=w380) -> ()  [unwired: 2 in, 2 out]
                          }
                        }
                        n301 = property on="GaAs buffer 0.6 μm/h" class="Bool (strict)"("Val(Sgnl)"=TRUE ("Value (Signaling)")) -> ()  [unwired: 2 in, 2 out]
                        n302 = property on="Reminder Information" class="Str"("Val(Sgnl)"="Start temperature adjustment and wait 3 minutes to stabilize for GaAs growth." ("Value (Signaling)")) -> ()  [unwired: 2 in, 2 out]
                      }
                      frame #6 {
                        n303 = Wait (ms)(milliseconds to wait=u32 100) -> ()  [unwired: 1 out]
                        n304 = property on="倒计时开关" class="Bool (strict)"("Val(Sgnl)"=FALSE ("Value (Signaling)")) -> ()  [unwired: 2 in, 2 out]
                      }
                      frame #7 {
                        n305 = property on="nm 3" class="DigNum (strict)"() -> ("Value"=w389:u32)  [unwired: 2 in, 2 out]
                        n306 = Divide(x=0.6, y=3.6) -> (x/y=w398:dbl)
                        n307 = Divide(x=w389, y=w398) -> (x/y=w397:dbl)
                        n308 = property on="As挡板" class="Bool (strict)"("Val(Sgnl)"=TRUE ("Value (Signaling)")) -> ()  [unwired: 2 in, 2 out]
                        n309 = property on="In挡板" class="Bool (strict)"("Val(Sgnl)"=FALSE ("Value (Signaling)")) -> ()  [unwired: 2 in, 2 out]
                        n310 = property on="Ga2挡板" class="Bool (strict)"("Val(Sgnl)"=TRUE ("Value (Signaling)")) -> ()  [unwired: 2 in, 2 out]
                        n311 = property on="Main挡板" class="Bool (strict)"("Val(Sgnl)"=TRUE ("Value (Signaling)")) -> ()  [unwired: 2 in, 2 out]
                        n312 = while {
                          shift-right: [w400] -> _
                          shift-left: w397 -> [w402]
                          stop <- w401 stop-if-true
                          n313 = Decrement(x=w402) -> (x-1=w400:dbl)
                          n314 = Wait (ms)(milliseconds to wait=u32 1000) -> ()  [unwired: 1 out]
                          n315 = property on="Countdow" class="DigNum (strict)"("Val(Sgnl)"=w400) -> ()  [unwired: 2 in, 2 out]
                          n316 = Less Or Equal To 0?(x=w400) -> (x <= 0?=w399:bool)
                          n317 = property on="倒计时开关" class="Bool (strict)"("Val(Sgnl)"=w399) -> ()  [unwired: 2 in, 2 out]
                          n318 = property on="倒计时开关" class="Bool (strict)"() -> ("Value"=w401:bool)  [unwired: 2 in, 2 out]
                        }
                        n319 = property on="Reminder Information" class="Str"("Val(Sgnl)"="Start the growth of GaAs buffer." ("Value (Signaling)")) -> ()  [unwired: 2 in, 2 out]
                      }
                      frame #8 {
                        n320 = Wait (ms)(milliseconds to wait=u32 100) -> ()  [unwired: 1 out]
                        n321 = property on="倒计时开关" class="Bool (strict)"("Val(Sgnl)"=FALSE ("Value (Signaling)")) -> ()  [unwired: 2 in, 2 out]
                      }
                      frame #9 {
                        n322 = property on="Main挡板" class="Bool (strict)"("Val(Sgnl)"=TRUE ("Value (Signaling)")) -> ()  [unwired: 2 in, 2 out]
                        n323 = while {
                          shift-right: [w412] -> _
                          shift-left: 5.0 -> [w415]
                          stop <- w414 stop-if-true
                          n324 = Decrement(x=w415) -> (x-1=w412:dbl)
                          n325 = property on="Countdow" class="DigNum (strict)"("Val(Sgnl)"=w412) -> ()  [unwired: 2 in, 2 out]
                          n326 = Less Or Equal To 0?(x=w412) -> (x <= 0?=w413:bool)
                          n327 = Wait (ms)(milliseconds to wait=u32 1000) -> ()  [unwired: 1 out]
                          n328 = property on="倒计时开关" class="Bool (strict)"("Val(Sgnl)"=w413) -> ()  [unwired: 2 in, 2 out]
                          n329 = property on="倒计时开关" class="Bool (strict)"() -> ("Value"=w414:bool)  [unwired: 2 in, 2 out]
                        }
                        n330 = property on="As挡板" class="Bool (strict)"("Val(Sgnl)"=TRUE ("Value (Signaling)")) -> ()  [unwired: 2 in, 2 out]
                        n331 = property on="Ga2挡板" class="Bool (strict)"("Val(Sgnl)"=FALSE ("Value (Signaling)")) -> ()  [unwired: 2 in, 2 out]
                        n332 = property on="In挡板" class="Bool (strict)"("Val(Sgnl)"=FALSE ("Value (Signaling)")) -> ()  [unwired: 2 in, 2 out]
                        n333 = property on="Reminder Information" class="Str"("Val(Sgnl)"="Finish the growth of GaAs buffer." ("Value (Signaling)")) -> ()  [unwired: 2 in, 2 out]
                      }
                      frame #10 {
                        n334 = Wait (ms)(milliseconds to wait=u32 100) -> ()  [unwired: 1 out]
                        n335 = property on="倒计时开关" class="Bool (strict)"("Val(Sgnl)"=FALSE ("Value (Signaling)")) -> ()  [unwired: 2 in, 2 out]
                        n336 = property on="GaAs buffer 0.6 μm/h" class="Bool (strict)"("Val(Sgnl)"=FALSE ("Value (Signaling)")) -> ()  [unwired: 2 in, 2 out]
                      }
                    }
                  }
                  frame #2 {
                    n337 = flat-sequence {
                      frame #0 {
                        n338 = property on="As挡板" class="Bool (strict)"("Val(Sgnl)"=TRUE ("Value (Signaling)")) -> ()  [unwired: 2 in, 2 out]
                        n339 = while {
                          shift-right: [w429] -> _
                          shift-left: 5.0 -> [w432]
                          stop <- w431 stop-if-true
                          n340 = Decrement(x=w432) -> (x-1=w429:dbl)
                          n341 = property on="Countdow" class="DigNum (strict)"("Val(Sgnl)"=w429) -> ()  [unwired: 2 in, 2 out]
                          n342 = Less Or Equal To 0?(x=w429) -> (x <= 0?=w430:bool)
                          n343 = Wait (ms)(milliseconds to wait=u32 1000) -> ()  [unwired: 1 out]
                          n344 = property on="倒计时开关" class="Bool (strict)"("Val(Sgnl)"=w430) -> ()  [unwired: 2 in, 2 out]
                          n345 = property on="倒计时开关" class="Bool (strict)"() -> ("Value"=w431:bool)  [unwired: 2 in, 2 out]
                        }
                        n346 = property on="Sub设定" class="Str"("Val(Sgnl)"="50" ("Value (Signaling)")) -> ()  [unwired: 2 in, 2 out]
                        n347 = property on="Main挡板" class="Bool (strict)"("Val(Sgnl)"=TRUE ("Value (Signaling)")) -> ()  [unwired: 2 in, 2 out]
                        n348 = property on="Cool to less than 100 ℃ and wait 20 minutes" class="Bool (strict)"("Val(Sgnl)"=TRUE ("Value (Signaling)")) -> ()  [unwired: 2 in, 2 out]
                        n349 = property on="Ga2挡板" class="Bool (strict)"("Val(Sgnl)"=FALSE ("Value (Signaling)")) -> ()  [unwired: 2 in, 2 out]
                        n350 = property on="Ga2设定" class="Str"("Val(Sgnl)"="890" ("Value (Signaling)")) -> ()  [unwired: 2 in, 2 out]
                        n351 = property on="In挡板" class="Bool (strict)"("Val(Sgnl)"=FALSE ("Value (Signaling)")) -> ()  [unwired: 2 in, 2 out]
                        n352 = property on="Reminder Information" class="Str"("Val(Sgnl)"="Cool the substrate to less than 100 ℃ and wait 20 minutes." ("Value (Signaling)")) -> ()  [unwired: 2 in, 2 out]
                      }
                      frame #1 {
                        n353 = Wait (ms)(milliseconds to wait=u32 100) -> ()  [unwired: 1 out]
                        n354 = property on="倒计时开关" class="Bool (strict)"("Val(Sgnl)"=FALSE ("Value (Signaling)")) -> ()  [unwired: 2 in, 2 out]
                      }
                      frame #2 {
                        n355 = while {
                          stop <- w438 stop-if-true
                          n356 = property on="While loop for cool to less than 100 ℃" class="Bool (strict)"() -> ("Value"=w437:bool)  [unwired: 2 in, 2 out]
                          n357 = property on="Sub实测" class="Str"() -> ("Value"=w441:string)  [unwired: 2 in, 2 out]
                          n358 = Decimal String To Number(string=w441) -> (number=w439:i32)  [unwired: 2 in, 1 out]
                          n359 = Less?(x=w439, y=100.0) -> (x < y?=w436:bool)
                          n360 = case shown="False" w437 {
                            tunnel: w436 -> [w442 _]
                            frame False {
                              n361 = case shown="True" w442 {
                                frame True {
                                n362 = flat-sequence {
                                frame #0 {
                                n363 = while {
                                shift-right: [w445] -> _
                                shift-left: 5.0 -> [w448]
                                stop <- w447 stop-if-true
                                n364 = Decrement(x=w448) -> (x-1=w445:dbl)
                                n365 = property on="Countdow" class="DigNum (strict)"("Val(Sgnl)"=w445) -> ()  [unwired: 2 in, 2 out]
                                n366 = Less Or Equal To 0?(x=w445) -> (x <= 0?=w446:bool)
                                n367 = Wait (ms)(milliseconds to wait=u32 1000) -> ()  [unwired: 1 out]
                                n368 = property on="倒计时开关" class="Bool (strict)"("Val(Sgnl)"=w446) -> ()  [unwired: 2 in, 2 out]
                                n369 = property on="倒计时开关" class="Bool (strict)"() -> ("Value"=w447:bool)  [unwired: 2 in, 2 out]
                                }
                                n370 = property on="Reminder Information" class="Str"("Val(Sgnl)"="The temperature of the substrate is less than 100 ℃." ("Value (Signaling)")) -> ()  [unwired: 2 in, 2 out]
                                }
                                frame #1 {
                                n371 = Wait (ms)(milliseconds to wait=u32 100) -> ()  [unwired: 1 out]
                                n372 = property on="倒计时开关" class="Bool (strict)"("Val(Sgnl)"=FALSE ("Value (Signaling)")) -> ()  [unwired: 2 in, 2 out]
                                }
                                frame #2 {
                                n373 = Multiply(x=20.0, y=60.0) -> (x*y=w452:dbl)
                                n374 = while {
                                shift-right: [w456] -> _
                                shift-left: w452 -> [w459]
                                stop <- w458 stop-if-true
                                n375 = Decrement(x=w459) -> (x-1=w456:dbl)
                                n376 = property on="Countdow" class="DigNum (strict)"("Val(Sgnl)"=w456) -> ()  [unwired: 2 in, 2 out]
                                n377 = Wait (ms)(milliseconds to wait=u32 1000) -> ()  [unwired: 1 out]
                                n378 = Less Or Equal To 0?(x=w456) -> (x <= 0?=w457:bool)
                                n379 = property on="倒计时开关" class="Bool (strict)"("Val(Sgnl)"=w457) -> ()  [unwired: 2 in, 2 out]
                                n380 = property on="倒计时开关" class="Bool (strict)"() -> ("Value"=w458:bool)  [unwired: 2 in, 2 out]
                                }
                                n381 = property on="Reminder Information" class="Str"("Val(Sgnl)"="Wait for about 20 minutes." ("Value (Signaling)")) -> ()  [unwired: 2 in, 2 out]
                                }
                                frame #3 {
                                n382 = Wait (ms)(milliseconds to wait=u32 100) -> ()  [unwired: 1 out]
                                n383 = property on="倒计时开关" class="Bool (strict)"("Val(Sgnl)"=FALSE ("Value (Signaling)")) -> ()  [unwired: 2 in, 2 out]
                                n384 = property on="While loop for cool to less than 100 ℃" class="Bool (strict)"("Val(Sgnl)"=TRUE ("Value (Signaling)")) -> ()  [unwired: 2 in, 2 out]
                                }
                                }
                                }
                                frame False {
                                n385 = flat-sequence {
                                frame #0 {
                                n386 = while {
                                shift-right: [w466] -> _
                                shift-left: 5.0 -> [w469]
                                stop <- w468 stop-if-true
                                n387 = Decrement(x=w469) -> (x-1=w466:dbl)
                                n388 = property on="Countdow" class="DigNum (strict)"("Val(Sgnl)"=w466) -> ()  [unwired: 2 in, 2 out]
                                n389 = Less Or Equal To 0?(x=w466) -> (x <= 0?=w467:bool)
                                n390 = Wait (ms)(milliseconds to wait=u32 1000) -> ()  [unwired: 1 out]
                                n391 = property on="倒计时开关" class="Bool (strict)"("Val(Sgnl)"=w467) -> ()  [unwired: 2 in, 2 out]
                                n392 = property on="倒计时开关" class="Bool (strict)"() -> ("Value"=w468:bool)  [unwired: 2 in, 2 out]
                                }
                                n393 = property on="Reminder Information" class="Str"("Val(Sgnl)"="The temperature of the substrate is not less than 100 ℃." ("Value (Signaling)")) -> ()  [unwired: 2 in, 2 out]
                                }
                                frame #1 {
                                n394 = Wait (ms)(milliseconds to wait=u32 100) -> ()  [unwired: 1 out]
                                n395 = property on="倒计时开关" class="Bool (strict)"("Val(Sgnl)"=FALSE ("Value (Signaling)")) -> ()  [unwired: 2 in, 2 out]
                                n396 = property on="While loop for cool to less than 100 ℃" class="Bool (strict)"("Val(Sgnl)"=FALSE ("Value (Signaling)")) -> ()  [unwired: 2 in, 2 out]
                                }
                                }
                                }
                              }
                            }
                            frame True {
                            }
                          }
                          n397 = property on="While loop for cool to less than 100 ℃" class="Bool (strict)"() -> ("Value"=w438:bool)  [unwired: 2 in, 2 out]
                        }
                      }
                      frame #3 {
                        n398 = while {
                          shift-right: [w476] -> _
                          shift-left: 5.0 -> [w479]
                          stop <- w478 stop-if-true
                          n399 = Decrement(x=w479) -> (x-1=w476:dbl)
                          n400 = property on="Countdow" class="DigNum (strict)"("Val(Sgnl)"=w476) -> ()  [unwired: 2 in, 2 out]
                          n401 = Less Or Equal To 0?(x=w476) -> (x <= 0?=w477:bool)
                          n402 = Wait (ms)(milliseconds to wait=u32 1000) -> ()  [unwired: 1 out]
                          n403 = property on="倒计时开关" class="Bool (strict)"("Val(Sgnl)"=w477) -> ()  [unwired: 2 in, 2 out]
                          n404 = property on="倒计时开关" class="Bool (strict)"() -> ("Value"=w478:bool)  [unwired: 2 in, 2 out]
                        }
                        n405 = property on="Reminder Information" class="Str"("Val(Sgnl)"="Finish the cooling of the substrate." ("Value (Signaling)")) -> ()  [unwired: 2 in, 2 out]
                      }
                      frame #4 {
                        n406 = Wait (ms)(milliseconds to wait=u32 100) -> ()  [unwired: 1 out]
                        n407 = property on="倒计时开关" class="Bool (strict)"("Val(Sgnl)"=FALSE ("Value (Signaling)")) -> ()  [unwired: 2 in, 2 out]
                        n408 = property on="Cool to less than 100 ℃ and wait 20 minutes" class="Bool (strict)"("Val(Sgnl)"=FALSE ("Value (Signaling)")) -> ()  [unwired: 2 in, 2 out]
                      }
                    }
                  }
                }
                n409 = property on="Growth Switch" class="DigNum (strict)"() -> ("Value"=w141:i32)  [unwired: 2 in, 2 out]
                n410 = Increment(x=w141) -> (x+1=w142:i32)
                n411 = property on="Growth Switch" class="DigNum (strict)"("Val(Sgnl)"=w142) -> ()  [unwired: 2 in, 2 out]
                n412 = property on="Tab Control" class="TabCtl (strict)"("Value"=T1."Growth Temperature Initialization" ("Value (Signaling)")) -> ()  [unwired: 2 in, 2 out]
              }
              frame 1 {
                n413 = flat-sequence {
                  frame #0 {
                    n414 = flat-sequence {
                      frame #0 {
                        n415 = property on="Sub速度" class="Str"("Val(Sgnl)"="15" ("Value (Signaling)")) -> ()  [unwired: 2 in, 2 out]
                        n416 = property on="Obtaining the reconstruction  temperature" class="Bool (strict)"("Val(Sgnl)"=TRUE ("Value (Signaling)")) -> ()  [unwired: 2 in, 2 out]
                        n417 = property on="摄像头开关" class="Bool (strict)"("Val(Sgnl)"=TRUE ("Value (Signaling)")) -> ()  [unwired: 2 in, 2 out]
                        n418 = while {
                          shift-right: [w492] -> _
                          shift-left: 120.0 -> [w495]
                          stop <- w494 stop-if-true
                          n419 = Decrement(x=w495) -> (x-1=w492:dbl)
                          n420 = Wait (ms)(milliseconds to wait=u32 1000) -> ()  [unwired: 1 out]
                          n421 = property on="Countdow" class="DigNum (strict)"("Val(Sgnl)"=w492) -> ()  [unwired: 2 in, 2 out]
                          n422 = Less Or Equal?(x=w492, y=15.0) -> (x <= y?=w493:bool)
                          n423 = property on="倒计时开关" class="Bool (strict)"("Val(Sgnl)"=w493) -> ()  [unwired: 2 in, 2 out]
                          n424 = property on="倒计时开关" class="Bool (strict)"() -> ("Value"=w494:bool)  [unwired: 2 in, 2 out]
                        }
                        n425 = property on="Reminder Information" class="Str"("Val(Sgnl)"="There are 120 seconds left, please open the RHEED shutter manually." ("Value (Signaling)")) -> ()  [unwired: 2 in, 2 out]
                      }
                      frame #1 {
                        n426 = Wait (ms)(milliseconds to wait=u32 100) -> ()  [unwired: 1 out]
                        n427 = property on="倒计时开关" class="Bool (strict)"("Val(Sgnl)"=FALSE ("Value (Signaling)")) -> ()  [unwired: 2 in, 2 out]
                      }
                      frame #2 {
                        n428 = property on="Model switch" class="Bool (strict)"("Val(Sgnl)"=TRUE ("Value (Signaling)")) -> ()  [unwired: 2 in, 2 out]
                        n429 = while {
                          shift-right: [w502] -> _
                          shift-left: 15.0 -> [w504]
                          stop <- w503 stop-if-true
                          n430 = Decrement(x=w504) -> (x-1=w502:dbl)
                          n431 = Wait (ms)(milliseconds to wait=u32 1000) -> ()  [unwired: 1 out]
                          n432 = property on="Countdow" class="DigNum (strict)"("Val(Sgnl)"=w502) -> ()  [unwired: 2 in, 2 out]
                          n433 = Less Or Equal To 0?(x=w502) -> (x <= 0?=w501:bool)
                          n434 = property on="倒计时开关" class="Bool (strict)"("Val(Sgnl)"=w501) -> ()  [unwired: 2 in, 2 out]
                          n435 = property on="倒计时开关" class="Bool (strict)"() -> ("Value"=w503:bool)  [unwired: 2 in, 2 out]
                        }
                      }
                      frame #3 {
                        n436 = Wait (ms)(milliseconds to wait=u32 100) -> ()  [unwired: 1 out]
                        n437 = property on="倒计时开关" class="Bool (strict)"("Val(Sgnl)"=FALSE ("Value (Signaling)")) -> ()  [unwired: 2 in, 2 out]
                      }
                    }
                  }
                  frame #1 {
                    n438 = while {
                      stop <- w510 stop-if-true
                      n439 = property on="Is the probability of the model output c(4×4) exceeding" class="Bool (strict)"() -> ("Value"=w508:bool)  [unwired: 2 in, 2 out]
                      n440 = property on="Whether to continue heat up for reconstruction" class="Bool (strict)"() -> ("Value"=w509:bool)  [unwired: 2 in, 2 out]
                      n441 = case shown="False" w509 {
                        tunnel: w508 -> [w511 _]
                        frame False {
                          n442 = case shown="True" w511 {
                            frame False {
                              n443 = flat-sequence "Model determined substrate dexoidation" {
                                frame #0 {
                                n444 = property on="Sub实测" class="Str"() -> ("Value"=w514:string)  [unwired: 2 in, 2 out]
                                n445 = while {
                                shift-right: [w521] -> _
                                shift-left: 5.0 -> [w523]
                                stop <- w522 stop-if-true
                                n446 = Decrement(x=w523) -> (x-1=w521:dbl)
                                n447 = Wait (ms)(milliseconds to wait=u32 1000) -> ()  [unwired: 1 out]
                                n448 = property on="Countdow" class="DigNum (strict)"("Val(Sgnl)"=w521) -> ()  [unwired: 2 in, 2 out]
                                n449 = Less Or Equal To 0?(x=w521) -> (x <= 0?=w520:bool)
                                n450 = property on="倒计时开关" class="Bool (strict)"("Val(Sgnl)"=w520) -> ()  [unwired: 2 in, 2 out]
                                n451 = property on="倒计时开关" class="Bool (strict)"() -> ("Value"=w522:bool)  [unwired: 2 in, 2 out]
                                }
                                n452 = property on="Whether to continue heat up for reconstruction" class="Bool (strict)"("Val(Sgnl)"=FALSE ("Value (Signaling)")) -> ()  [unwired: 2 in, 2 out]
                                n453 = Decimal String To Number(string=w514) -> (number=w518:i32)  [unwired: 2 in, 1 out]
                                n454 = Add(x=w518, y=10) -> (x+y=w519:i32)
                                n455 = Number To Decimal String(number=w519) -> (decimal integer string=w513:string)  [unwired: 1 in]
                                n456 = property on="Sub设定" class="Str"("Val(Sgnl)"=w513) -> ()  [unwired: 2 in, 2 out]
                                n457 = property on="Substrate to find Reconstruction temperature" class="Str"("Val(Sgnl)"=w513) -> ()  [unwired: 2 in, 2 out]
                                n458 = property on="Reminder Information" class="Str"("Val(Sgnl)"="The model determines that the substrate has not yet been c(4×4), and then set substrate temperature continues to rise." ("Value (Signaling)")) -> ()  [unwired: 2 in, 2 out]
                                }
                                frame #1 {
                                n459 = Wait (ms)(milliseconds to wait=u32 100) -> ()  [unwired: 1 out]
                                n460 = property on="倒计时开关" class="Bool (strict)"("Val(Sgnl)"=FALSE ("Value (Signaling)")) -> ()  [unwired: 2 in, 2 out]
                                n461 = property on="Whether to continue heat up for reconstruction" class="Bool (strict)"("Val(Sgnl)"=FALSE ("Value (Signaling)")) -> ()  [unwired: 2 in, 2 out]
                                }
                              }
                            }
                            frame True {
                              n462 = flat-sequence {
                                frame #0 {
                                n463 = property on="Sub实测" class="Str"() -> ("Value"=w531:string)  [unwired: 2 in, 2 out]
                                n464 = property on="Whether to continue heat up for reconstruction" class="Bool (strict)"("Val(Sgnl)"=TRUE ("Value (Signaling)")) -> ()  [unwired: 2 in, 2 out]
                                n465 = property on="From As cap to c(4×4)" class="Str"("Val(Sgnl)"=w531) -> ()  [unwired: 2 in, 2 out]
                                }
                                frame #1 {
                                n466 = Wait (ms)(milliseconds to wait=u32 100) -> ()  [unwired: 1 out]
                                n467 = property on="倒计时开关" class="Bool (strict)"("Val(Sgnl)"=FALSE ("Value (Signaling)")) -> ()  [unwired: 2 in, 2 out]
                                n468 = property on="Whether to continue heat up for reconstruction" class="Bool (strict)"("Val(Sgnl)"=TRUE ("Value (Signaling)")) -> ()  [unwired: 2 in, 2 out]
                                }
                              }
                              n469 = Wait (ms)(milliseconds to wait=u32 1000) -> ()  [unwired: 1 out]
                              n470 = property on="Reminder Information" class="Str"("Val(Sgnl)"="The model determines that the reconstruction has been c(4×4)." ("Value (Signaling)")) -> ()  [unwired: 2 in, 2 out]
                            }
                          }
                        }
                        frame True {
                        }
                      }
                      n471 = property on="Whether to continue heat up for reconstruction" class="Bool (strict)"() -> ("Value"=w510:bool)  [unwired: 2 in, 2 out]
                    }
                  }
                  frame #2 {
                    n472 = property on="Whether to continue heat up for reconstruction" class="Bool (strict)"("Val(Sgnl)"=FALSE ("Value (Signaling)")) -> ()  [unwired: 2 in, 2 out]
                    n473 = property on="倒计时开关" class="Bool (strict)"("Val(Sgnl)"=FALSE ("Value (Signaling)")) -> ()  [unwired: 2 in, 2 out]
                    n474 = Wait (ms)(milliseconds to wait=u32 1000) -> ()  [unwired: 1 out]
                  }
                  frame #3 {
                    n475 = while {
                      stop <- w540 stop-if-true
                      n476 = property on="Is the probability of the model output (2×4) exceeding" class="Bool (strict)"() -> ("Value"=w538:bool)  [unwired: 2 in, 2 out]
                      n477 = property on="Whether to continue heat up for reconstruction" class="Bool (strict)"() -> ("Value"=w539:bool)  [unwired: 2 in, 2 out]
                      n478 = case shown="False" w539 {
                        tunnel: w538 -> [w541 _]
                        frame False {
                          n479 = case shown="True" w541 {
                            frame False {
                              n480 = flat-sequence "Model determined substrate dexoidation" {
                                frame #0 {
                                n481 = property on="Sub实测" class="Str"() -> ("Value"=w544:string)  [unwired: 2 in, 2 out]
                                n482 = while {
                                shift-right: [w551] -> _
                                shift-left: 5.0 -> [w553]
                                stop <- w552 stop-if-true
                                n483 = Decrement(x=w553) -> (x-1=w551:dbl)
                                n484 = Wait (ms)(milliseconds to wait=u32 1000) -> ()  [unwired: 1 out]
                                n485 = property on="Countdow" class="DigNum (strict)"("Val(Sgnl)"=w551) -> ()  [unwired: 2 in, 2 out]
                                n486 = Less Or Equal To 0?(x=w551) -> (x <= 0?=w550:bool)
                                n487 = property on="倒计时开关" class="Bool (strict)"("Val(Sgnl)"=w550) -> ()  [unwired: 2 in, 2 out]
                                n488 = property on="倒计时开关" class="Bool (strict)"() -> ("Value"=w552:bool)  [unwired: 2 in, 2 out]
                                }
                                n489 = property on="Whether to continue heat up for reconstruction" class="Bool (strict)"("Val(Sgnl)"=FALSE ("Value (Signaling)")) -> ()  [unwired: 2 in, 2 out]
                                n490 = Decimal String To Number(string=w544) -> (number=w548:i32)  [unwired: 2 in, 1 out]
                                n491 = Add(x=w548, y=10) -> (x+y=w549:i32)
                                n492 = Number To Decimal String(number=w549) -> (decimal integer string=w543:string)  [unwired: 1 in]
                                n493 = property on="Sub设定" class="Str"("Val(Sgnl)"=w543) -> ()  [unwired: 2 in, 2 out]
                                n494 = property on="Substrate to find Reconstruction temperature" class="Str"("Val(Sgnl)"=w543) -> ()  [unwired: 2 in, 2 out]
                                n495 = property on="Reminder Information" class="Str"("Val(Sgnl)"="The model determines that the substrate has not yet been (2×4), and then set substrate temperature continues to rise." ("Value (Signaling)")) -> ()  [unwired: 2 in, 2 out]
                                }
                                frame #1 {
                                n496 = Wait (ms)(milliseconds to wait=u32 100) -> ()  [unwired: 1 out]
                                n497 = property on="倒计时开关" class="Bool (strict)"("Val(Sgnl)"=FALSE ("Value (Signaling)")) -> ()  [unwired: 2 in, 2 out]
                                n498 = property on="Whether to continue heat up for reconstruction" class="Bool (strict)"("Val(Sgnl)"=FALSE ("Value (Signaling)")) -> ()  [unwired: 2 in, 2 out]
                                }
                              }
                            }
                            frame True {
                              n499 = flat-sequence {
                                frame #0 {
                                n500 = property on="Sub实测" class="Str"() -> ("Value"=w561:string)  [unwired: 2 in, 2 out]
                                n501 = while {
                                shift-right: [w564] -> _
                                shift-left: 5.0 -> [w566]
                                stop <- w565 stop-if-true
                                n502 = Decrement(x=w566) -> (x-1=w564:dbl)
                                n503 = Wait (ms)(milliseconds to wait=u32 1000) -> ()  [unwired: 1 out]
                                n504 = property on="Countdow" class="DigNum (strict)"("Val(Sgnl)"=w564) -> ()  [unwired: 2 in, 2 out]
                                n505 = Less Or Equal To 0?(x=w564) -> (x <= 0?=w563:bool)
                                n506 = property on="倒计时开关" class="Bool (strict)"("Val(Sgnl)"=w563) -> ()  [unwired: 2 in, 2 out]
                                n507 = property on="倒计时开关" class="Bool (strict)"() -> ("Value"=w565:bool)  [unwired: 2 in, 2 out]
                                }
                                n508 = property on="Whether to continue heat up for reconstruction" class="Bool (strict)"("Val(Sgnl)"=TRUE ("Value (Signaling)")) -> ()  [unwired: 2 in, 2 out]
                                n509 = property on="From c(4×4) to (2×4)" class="Str"("Val(Sgnl)"=w561) -> ()  [unwired: 2 in, 2 out]
                                }
                                frame #1 {
                                n510 = Wait (ms)(milliseconds to wait=u32 100) -> ()  [unwired: 1 out]
                                n511 = property on="倒计时开关" class="Bool (strict)"("Val(Sgnl)"=FALSE ("Value (Signaling)")) -> ()  [unwired: 2 in, 2 out]
                                n512 = property on="Whether to continue heat up for reconstruction" class="Bool (strict)"("Val(Sgnl)"=TRUE ("Value (Signaling)")) -> ()  [unwired: 2 in, 2 out]
                                }
                              }
                              n513 = Wait (ms)(milliseconds to wait=u32 1000) -> ()  [unwired: 1 out]
                              n514 = property on="Reminder Information" class="Str"("Val(Sgnl)"="The model determines that the reconstruction has been (2×4)." ("Value (Signaling)")) -> ()  [unwired: 2 in, 2 out]
                            }
                          }
                        }
                        frame True {
                        }
                      }
                      n515 = property on="Whether to continue heat up for reconstruction" class="Bool (strict)"() -> ("Value"=w540:bool)  [unwired: 2 in, 2 out]
                    }
                  }
                  frame #4 {
                    n516 = property on="Whether to continue heat up for reconstruction" class="Bool (strict)"("Val(Sgnl)"=FALSE ("Value (Signaling)")) -> ()  [unwired: 2 in, 2 out]
                    n517 = property on="倒计时开关" class="Bool (strict)"("Val(Sgnl)"=FALSE ("Value (Signaling)")) -> ()  [unwired: 2 in, 2 out]
                    n518 = Wait (ms)(milliseconds to wait=u32 1000) -> ()  [unwired: 1 out]
                  }
                  frame #5 {
                    n519 = while {
                      stop <- w576 stop-if-true
                      n520 = property on="Is the probability of the model output (n×6) exceeding" class="Bool (strict)"() -> ("Value"=w574:bool)  [unwired: 2 in, 2 out]
                      n521 = property on="Whether to continue heat up for reconstruction" class="Bool (strict)"() -> ("Value"=w575:bool)  [unwired: 2 in, 2 out]
                      n522 = case shown="False" w575 {
                        tunnel: w574 -> [w577 _]
                        frame False {
                          n523 = case shown="True" w577 {
                            frame False {
                              n524 = flat-sequence "Model determined substrate dexoidation" {
                                frame #0 {
                                n525 = property on="Sub实测" class="Str"() -> ("Value"=w580:string)  [unwired: 2 in, 2 out]
                                n526 = while {
                                shift-right: [w587] -> _
                                shift-left: 5.0 -> [w589]
                                stop <- w588 stop-if-true
                                n527 = Decrement(x=w589) -> (x-1=w587:dbl)
                                n528 = Wait (ms)(milliseconds to wait=u32 1000) -> ()  [unwired: 1 out]
                                n529 = property on="Countdow" class="DigNum (strict)"("Val(Sgnl)"=w587) -> ()  [unwired: 2 in, 2 out]
                                n530 = Less Or Equal To 0?(x=w587) -> (x <= 0?=w586:bool)
                                n531 = property on="倒计时开关" class="Bool (strict)"("Val(Sgnl)"=w586) -> ()  [unwired: 2 in, 2 out]
                                n532 = property on="倒计时开关" class="Bool (strict)"() -> ("Value"=w588:bool)  [unwired: 2 in, 2 out]
                                }
                                n533 = property on="Whether to continue heat up for reconstruction" class="Bool (strict)"("Val(Sgnl)"=FALSE ("Value (Signaling)")) -> ()  [unwired: 2 in, 2 out]
                                n534 = Decimal String To Number(string=w580) -> (number=w584:i32)  [unwired: 2 in, 1 out]
                                n535 = Add(x=w584, y=10) -> (x+y=w585:i32)
                                n536 = Number To Decimal String(number=w585) -> (decimal integer string=w579:string)  [unwired: 1 in]
                                n537 = property on="Sub设定" class="Str"("Val(Sgnl)"=w579) -> ()  [unwired: 2 in, 2 out]
                                n538 = property on="Substrate to find Reconstruction temperature" class="Str"("Val(Sgnl)"=w579) -> ()  [unwired: 2 in, 2 out]
                                n539 = property on="Reminder Information" class="Str"("Val(Sgnl)"="The model determines that the substrate has not yet been (n×6), and then set substrate temperature continues to rise." ("Value (Signaling)")) -> ()  [unwired: 2 in, 2 out]
                                }
                                frame #1 {
                                n540 = Wait (ms)(milliseconds to wait=u32 100) -> ()  [unwired: 1 out]
                                n541 = property on="倒计时开关" class="Bool (strict)"("Val(Sgnl)"=FALSE ("Value (Signaling)")) -> ()  [unwired: 2 in, 2 out]
                                n542 = property on="Whether to continue heat up for reconstruction" class="Bool (strict)"("Val(Sgnl)"=FALSE ("Value (Signaling)")) -> ()  [unwired: 2 in, 2 out]
                                }
                              }
                            }
                            frame True {
                              n543 = flat-sequence {
                                frame #0 {
                                n544 = property on="Sub实测" class="Str"() -> ("Value"=w597:string)  [unwired: 2 in, 2 out]
                                n545 = while {
                                shift-right: [w600] -> _
                                shift-left: 5.0 -> [w602]
                                stop <- w601 stop-if-true
                                n546 = Decrement(x=w602) -> (x-1=w600:dbl)
                                n547 = Wait (ms)(milliseconds to wait=u32 1000) -> ()  [unwired: 1 out]
                                n548 = property on="Countdow" class="DigNum (strict)"("Val(Sgnl)"=w600) -> ()  [unwired: 2 in, 2 out]
                                n549 = Less Or Equal To 0?(x=w600) -> (x <= 0?=w599:bool)
                                n550 = property on="倒计时开关" class="Bool (strict)"("Val(Sgnl)"=w599) -> ()  [unwired: 2 in, 2 out]
                                n551 = property on="倒计时开关" class="Bool (strict)"() -> ("Value"=w601:bool)  [unwired: 2 in, 2 out]
                                }
                                n552 = property on="From (2×4) to (n×6)" class="Str"("Val(Sgnl)"=w597) -> ()  [unwired: 2 in, 2 out]
                                n553 = property on="Whether to continue heat up for reconstruction" class="Bool (strict)"("Val(Sgnl)"=TRUE ("Value (Signaling)")) -> ()  [unwired: 2 in, 2 out]
                                }
                                frame #1 {
                                n554 = Wait (ms)(milliseconds to wait=u32 100) -> ()  [unwired: 1 out]
                                n555 = property on="倒计时开关" class="Bool (strict)"("Val(Sgnl)"=FALSE ("Value (Signaling)")) -> ()  [unwired: 2 in, 2 out]
                                n556 = property on="Whether to continue heat up for reconstruction" class="Bool (strict)"("Val(Sgnl)"=TRUE ("Value (Signaling)")) -> ()  [unwired: 2 in, 2 out]
                                }
                              }
                              n557 = Wait (ms)(milliseconds to wait=u32 1000) -> ()  [unwired: 1 out]
                              n558 = property on="Reminder Information" class="Str"("Val(Sgnl)"="The model determines that the reconstruction has been (n×6)." ("Value (Signaling)")) -> ()  [unwired: 2 in, 2 out]
                            }
                          }
                        }
                        frame True {
                        }
                      }
                      n559 = property on="Whether to continue heat up for reconstruction" class="Bool (strict)"() -> ("Value"=w576:bool)  [unwired: 2 in, 2 out]
                    }
                  }
                  frame #6 {
                    n560 = Wait (ms)(milliseconds to wait=u32 1000) -> ()  [unwired: 1 out]
                    n561 = property on="Whether to continue heat up for reconstruction" class="Bool (strict)"("Val(Sgnl)"=FALSE ("Value (Signaling)")) -> ()  [unwired: 2 in, 2 out]
                    n562 = property on="倒计时开关" class="Bool (strict)"("Val(Sgnl)"=FALSE ("Value (Signaling)")) -> ()  [unwired: 2 in, 2 out]
                  }
                  frame #7 {
                    n563 = property on="摄像头开关" class="Bool (strict)"("Val(Sgnl)"=FALSE ("Value (Signaling)")) -> ()  [unwired: 2 in, 2 out]
                    n564 = while {
                      shift-right: [w615] -> _
                      shift-left: 5.0 -> [w617]
                      stop <- w616 stop-if-true
                      n565 = Decrement(x=w617) -> (x-1=w615:dbl)
                      n566 = Wait (ms)(milliseconds to wait=u32 1000) -> ()  [unwired: 1 out]
                      n567 = property on="Countdow" class="DigNum (strict)"("Val(Sgnl)"=w615) -> ()  [unwired: 2 in, 2 out]
                      n568 = Less Or Equal To 0?(x=w615) -> (x <= 0?=w614:bool)
                      n569 = property on="倒计时开关" class="Bool (strict)"("Val(Sgnl)"=w614) -> ()  [unwired: 2 in, 2 out]
                      n570 = property on="倒计时开关" class="Bool (strict)"() -> ("Value"=w616:bool)  [unwired: 2 in, 2 out]
                    }
                    n571 = property on="Model switch" class="Bool (strict)"("Val(Sgnl)"=FALSE ("Value (Signaling)")) -> ()  [unwired: 2 in, 2 out]
                    n572 = property on="Reminder Information" class="Str"("Val(Sgnl)"="The RHEED shutter can now be closed." ("Value (Signaling)")) -> ()  [unwired: 2 in, 2 out]
                  }
                  frame #8 {
                    n573 = Wait (ms)(milliseconds to wait=u32 100) -> ()  [unwired: 1 out]
                    n574 = property on="倒计时开关" class="Bool (strict)"("Val(Sgnl)"=FALSE ("Value (Signaling)")) -> ()  [unwired: 2 in, 2 out]
                  }
                  frame #9 {
                    n575 = while {
                      shift-right: [w626] -> _
                      shift-left: 5.0 -> [w628]
                      stop <- w627 stop-if-true
                      n576 = Decrement(x=w628) -> (x-1=w626:dbl)
                      n577 = Wait (ms)(milliseconds to wait=u32 1000) -> ()  [unwired: 1 out]
                      n578 = property on="Countdow" class="DigNum (strict)"("Val(Sgnl)"=w626) -> ()  [unwired: 2 in, 2 out]
                      n579 = Less Or Equal To 0?(x=w626) -> (x <= 0?=w625:bool)
                      n580 = property on="倒计时开关" class="Bool (strict)"("Val(Sgnl)"=w625) -> ()  [unwired: 2 in, 2 out]
                      n581 = property on="倒计时开关" class="Bool (strict)"() -> ("Value"=w627:bool)  [unwired: 2 in, 2 out]
                    }
                    n582 = property on="Obtaining the reconstruction  temperature" class="Bool (strict)"("Val(Sgnl)"=FALSE ("Value (Signaling)")) -> ()  [unwired: 2 in, 2 out]
                    n583 = property on="Sub速度" class="Str"("Val(Sgnl)"="10" ("Value (Signaling)")) -> ()  [unwired: 2 in, 2 out]
                    n584 = property on="Reminder Information" class="Str"("Val(Sgnl)"="Finish obtaining the reconstruction temperature." ("Value (Signaling)")) -> ()  [unwired: 2 in, 2 out]
                  }
                  frame #10 {
                    n585 = Wait (ms)(milliseconds to wait=u32 100) -> ()  [unwired: 1 out]
                    n586 = property on="倒计时开关" class="Bool (strict)"("Val(Sgnl)"=FALSE ("Value (Signaling)")) -> ()  [unwired: 2 in, 2 out]
                  }
                  frame #11 {
                    n587 = property on="Obtain Growth Temperature" class="Bool (strict)"("Val(Sgnl)"=TRUE ("Value (Signaling)")) -> ()  [unwired: 2 in, 2 out]
                    n588 = while {
                      shift-right: [w636] -> _
                      shift-left: 5.0 -> [w638]
                      stop <- w637 stop-if-true
                      n589 = Decrement(x=w638) -> (x-1=w636:dbl)
                      n590 = Wait (ms)(milliseconds to wait=u32 1000) -> ()  [unwired: 1 out]
                      n591 = property on="Countdow" class="DigNum (strict)"("Val(Sgnl)"=w636) -> ()  [unwired: 2 in, 2 out]
                      n592 = Less Or Equal To 0?(x=w636) -> (x <= 0?=w635:bool)
                      n593 = property on="倒计时开关" class="Bool (strict)"("Val(Sgnl)"=w635) -> ()  [unwired: 2 in, 2 out]
                      n594 = property on="倒计时开关" class="Bool (strict)"() -> ("Value"=w637:bool)  [unwired: 2 in, 2 out]
                    }
                    n595 = property on="Reminder Information" class="Str"("Val(Sgnl)"="Start to obtain growth temperature." ("Value (Signaling)")) -> ()  [unwired: 2 in, 2 out]
                  }
                  frame #12 {
                    n596 = Wait (ms)(milliseconds to wait=u32 100) -> ()  [unwired: 1 out]
                    n597 = property on="倒计时开关" class="Bool (strict)"("Val(Sgnl)"=FALSE ("Value (Signaling)")) -> ()  [unwired: 2 in, 2 out]
                  }
                  frame #13 {
                    n598 = flat-sequence {
                      tunnel: [w663] -> w651
                      tunnel: [w662] -> w650
                      tunnel: ["fit_and_evaluate" ("函数名称")] -> w649
                      tunnel: [w660] -> w646
                      tunnel: [w659] -> w645
                      tunnel: [w658] -> w644
                      tunnel: [w657] -> w643
                      tunnel: [w653] -> w642
                      tunnel: [w696] -> w648
                      tunnel: [w695] -> w647
                      tunnel: w651 -> [w694]
                      tunnel: w650 -> [w693]
                      tunnel: w649 -> [w692]
                      tunnel: w646 -> [w684]
                      tunnel: w645 -> [w683]
                      tunnel: w644 -> [w682]
                      tunnel: w643 -> [w681]
                      tunnel: w642 -> [w680]
                      tunnel: w648 -> [w706]
                      tunnel: w647 -> [w705]
                      frame #0 {
                        n599 = Wait (ms)(milliseconds to wait=u32 100) -> ()  [unwired: 1 out]
                        n600 = property on="Deoxidation temperature" class="Str"() -> ("Value"=w659:string)  [unwired: 2 in, 2 out]
                        n601 = property on="From As cap to c(4×4)" class="Str"() -> ("Value"=w657:string)  [unwired: 2 in, 2 out]
                        n602 = Current VI's Path() -> (path=w656:path)
                        n603 = property on="From c(4×4) to (2×4)" class="Str"() -> ("Value"=w658:string)  [unwired: 2 in, 2 out]
                        n604 = property on="From (2×4) to (n×6)" class="Str"() -> ("Value"=w660:string)  [unwired: 2 in, 2 out]
                        n605 = Strip Path(path=w656) -> (stripped path=w655:path)  [unwired: 1 out]
                        n606 = Open Python Session(python version="3.9" ("Python版本"), python path=path "C:/Users/meiyo/anaconda3/envs/pytorchnn/python.exe" ("Python path")) -> (session out=w663:refnum<k35>, error out=w662:errorcluster)  [unwired: 1 in]
                        n607 = Build Path(base path=w655, name or relative path=".\\unsupervised curve fitting Labview.py") -> (appended path=w653:path)
                      }
                      frame #1 {
                        w666 = i16 0 ("precision (6)")
                        n608 = Decimal String To Number(string=w681) -> (number=w699:i32)  [unwired: 2 in, 1 out]
                        n609 = Decimal String To Number(string=w682) -> (number=w700:i32)  [unwired: 2 in, 1 out]
                        n610 = Decimal String To Number(string=w683) -> (number=w701:i32)  [unwired: 2 in, 1 out]
                        n611 = Decimal String To Number(string=w684) -> (number=w702:i32)  [unwired: 2 in, 1 out]
                        n612 = Wait (ms)(milliseconds to wait=u32 100) -> ()  [unwired: 1 out]
                        n613 = Build Array(w699, w700, w701, w702) -> (w703:i32[])
                        n614 = node(w694, w680, w692, w693, dbl[] [] ("return type"), w703, dbl[] [350.0, 510.0, 580.0, 620.0] ("多张图片处理后的数据结果 3")) -> (w696:refnum<k35>, w695:errorcluster, w685:dbl[])  [unwired: 2 in, 2 out]
                        n615 = Index Array(array=w685, index=0) -> (element=w679:dbl)
                        n616 = Index Array(array=w685, index=3) -> (element=w673:dbl)
                        n617 = Index Array(array=w685, index=4) -> (element=w671:dbl)
                        n618 = Index Array(array=w685, index=5) -> (element=w669:dbl)
                        n619 = Index Array(array=w685, index=1) -> (element=w677:dbl)
                        n620 = Index Array(array=w685, index=2) -> (element=w675:dbl)
                        n621 = Number To Fractional String(number=w679) -> (F-format string=w678:string)  [unwired: 3 in]
                        n622 = Number To Fractional String(number=w673) -> (F-format string=w672:string)  [unwired: 3 in]
                        n623 = Number To Fractional String(number=w671, precision (6)=w666) -> (F-format string=w670:string)  [unwired: 2 in]
                        n624 = Number To Fractional String(number=w669, precision (6)=w666) -> (F-format string=w668:string)  [unwired: 2 in]
                        n625 = Number To Fractional String(number=w677) -> (F-format string=w676:string)  [unwired: 3 in]
                        n626 = Number To Fractional String(number=w675) -> (F-format string=w674:string)  [unwired: 3 in]
                        n627 = property on="A =" class="Str"("Val(Sgnl)"=w678) -> ()  [unwired: 2 in, 2 out]
                        n628 = property on="MSE loss" class="Str"("Val(Sgnl)"=w672) -> ()  [unwired: 2 in, 2 out]
                        n629 = property on="InAs growth temperature" class="Str"("Val(Sgnl)"=w670) -> ()  [unwired: 2 in, 2 out]
                        n630 = property on="GaAs growth temperature" class="Str"("Val(Sgnl)"=w668) -> ()  [unwired: 2 in, 2 out]
                        n631 = property on="B =" class="Str"("Val(Sgnl)"=w676) -> ()  [unwired: 2 in, 2 out]
                        n632 = property on="C =" class="Str"("Val(Sgnl)"=w674) -> ()  [unwired: 2 in, 2 out]
                      }
                      frame #2 {
                        n633 = Close Python Session(session in=w706, error in=w705) -> ()  [unwired: 1 out]
                        n634 = Wait (ms)(milliseconds to wait=u32 100) -> ()  [unwired: 1 out]
                      }
                    }
                  }
                  frame #14 {
                    n635 = property on="GaAs growth temperature" class="Str"() -> ("Value"=w707:string)  [unwired: 2 in, 2 out]
                    n636 = property on="Obtain Growth Temperature" class="Bool (strict)"("Val(Sgnl)"=FALSE ("Value (Signaling)")) -> ()  [unwired: 2 in, 2 out]
                    n637 = while {
                      shift-right: [w713] -> _
                      shift-left: 5.0 -> [w715]
                      stop <- w714 stop-if-true
                      n638 = Decrement(x=w715) -> (x-1=w713:dbl)
                      n639 = Wait (ms)(milliseconds to wait=u32 1000) -> ()  [unwired: 1 out]
                      n640 = property on="Countdow" class="DigNum (strict)"("Val(Sgnl)"=w713) -> ()  [unwired: 2 in, 2 out]
                      n641 = Less Or Equal To 0?(x=w713) -> (x <= 0?=w712:bool)
                      n642 = property on="倒计时开关" class="Bool (strict)"("Val(Sgnl)"=w712) -> ()  [unwired: 2 in, 2 out]
                      n643 = property on="倒计时开关" class="Bool (strict)"() -> ("Value"=w714:bool)  [unwired: 2 in, 2 out]
                    }
                    n644 = property on="InAs growth temperature" class="Str"() -> ("Value"=w708:string)  [unwired: 2 in, 2 out]
                    n645 = property on="Sub3" class="Str"("Value"=w707) -> ()  [unwired: 2 in, 2 out]
                    n646 = property on="Sub1" class="Str"("Value"=w707) -> ()  [unwired: 2 in, 2 out]
                    n647 = property on="Sub4" class="Str"("Value"=w708) -> ()  [unwired: 2 in, 2 out]
                    n648 = property on="Sub2" class="Str"("Value"=w708) -> ()  [unwired: 2 in, 2 out]
                    n649 = property on="Reminder Information" class="Str"("Val(Sgnl)"="Finish obtaining growing temperature and complete temperature setting." ("Value (Signaling)")) -> ()  [unwired: 2 in, 2 out]
                  }
                  frame #15 {
                    n650 = Wait (ms)(milliseconds to wait=u32 100) -> ()  [unwired: 1 out]
                    n651 = property on="倒计时开关" class="Bool (strict)"("Val(Sgnl)"=FALSE ("Value (Signaling)")) -> ()  [unwired: 2 in, 2 out]
                  }
                }
                n652 = property on="Growth Switch" class="DigNum (strict)"() -> ("Value"=w484:i32)  [unwired: 2 in, 2 out]
                n653 = Increment(x=w484) -> (x+1=w485:i32)
                n654 = property on="Growth Switch" class="DigNum (strict)"("Val(Sgnl)"=w485) -> ()  [unwired: 2 in, 2 out]
              }
              frame 2 {
                n655 = flat-sequence "Ready" {
                  frame #0 {
                    n656 = Wait (ms)(milliseconds to wait=u32 100) -> ()  [unwired: 1 out]
                    n657 = property on="倒计时开关" class="Bool (strict)"("Val(Sgnl)"=FALSE ("Value (Signaling)")) -> ()  [unwired: 2 in, 2 out]
                  }
                  frame #1 {
                    n658 = flat-sequence {
                      tunnel: [w733] -> w726
                      tunnel: w726 -> [w745]
                      frame #0 {
                        n659 = property on="Sub实测" class="Str"() -> ("Value"=w743:string)  [unwired: 2 in, 2 out]
                        n660 = property on="Sub1" class="Str"() -> ("Value"=w734:string)  [unwired: 2 in, 2 out]
                        n661 = Decimal String To Number(string=w743) -> (number=w744:i32)  [unwired: 2 in, 1 out]
                        n662 = Decimal String To Number(string=w734) -> (number=w741:i32)  [unwired: 2 in, 1 out]
                        n663 = Subtract(x=w744, y=w741) -> (x-y=w742:i32)
                        n664 = Absolute Value(x=w742) -> (abs(x)=w740:i32)
                        n665 = Divide(x=w740, y=10) -> (x/y=w739:dbl)
                        n666 = Add(x=w739, y=6.0) -> (x+y=w738:dbl)
                        n667 = Multiply(x=w738, y=60.0) -> (x*y=w733:dbl)
                      }
                      frame #1 {
                        n668 = while {
                          shift-right: [w748] -> _
                          shift-left: w745 -> [w751]
                          stop <- w750 stop-if-true
                          n669 = Decrement(x=w751) -> (x-1=w748:dbl)
                          n670 = Wait (ms)(milliseconds to wait=u32 1000) -> ()  [unwired: 1 out]
                          n671 = property on="Countdow" class="DigNum (strict)"("Val(Sgnl)"=w748) -> ()  [unwired: 2 in, 2 out]
                          n672 = Less Or Equal To 0?(x=w748) -> (x <= 0?=w749:bool)
                          n673 = property on="倒计时开关" class="Bool (strict)"("Val(Sgnl)"=w749) -> ()  [unwired: 2 in, 2 out]
                          n674 = property on="倒计时开关" class="Bool (strict)"() -> ("Value"=w750:bool)  [unwired: 2 in, 2 out]
                        }
                        n675 = property on="Ga2 1" class="Str"() -> ("Value"=w746:string)  [unwired: 2 in, 2 out]
                        n676 = property on="Sub1" class="Str"() -> ("Value"=w747:string)  [unwired: 2 in, 2 out]
                        n677 = property on="Ga2设定" class="Str"("Val(Sgnl)"=w746) -> ()  [unwired: 2 in, 2 out]
                        n678 = property on="Sub设定" class="Str"("Val(Sgnl)"=w747) -> ()  [unwired: 2 in, 2 out]
                      }
                    }
                    n679 = property on="Ready for GaAs buffer 0.6 μm/h" class="Bool (strict)"("Val(Sgnl)"=TRUE ("Value (Signaling)")) -> ()  [unwired: 2 in, 2 out]
                    n680 = property on="Ga2挡板" class="Bool (strict)"("Val(Sgnl)"=FALSE ("Value (Signaling)")) -> ()  [unwired: 2 in, 2 out]
                    n681 = property on="As挡板" class="Bool (strict)"("Val(Sgnl)"=TRUE ("Value (Signaling)")) -> ()  [unwired: 2 in, 2 out]
                    n682 = property on="In挡板" class="Bool (strict)"("Val(Sgnl)"=FALSE ("Value (Signaling)")) -> ()  [unwired: 2 in, 2 out]
                    n683 = property on="In速度" class="Str"("Val(Sgnl)"="2" ("Value (Signaling)")) -> ()  [unwired: 2 in, 2 out]
                    n684 = property on="Main挡板" class="Bool (strict)"("Val(Sgnl)"=TRUE ("Value (Signaling)")) -> ()  [unwired: 2 in, 2 out]
                    n685 = property on="In设定" class="Str"("Val(Sgnl)"="680" ("Value (Signaling)")) -> ()  [unwired: 2 in, 2 out]
                    n686 = property on="Ga2速度" class="Str"("Val(Sgnl)"="6" ("Value (Signaling)")) -> ()  [unwired: 2 in, 2 out]
                    n687 = property on="Reminder Information" class="Str"("Val(Sgnl)"="Start temperature adjustment and wait for 6 minutes to stabilize, then manually adjust the As cracker needle valve." ("Value (Signaling)")) -> ()  [unwired: 2 in, 2 out]
                  }
                  frame #2 {
                    n688 = Wait (ms)(milliseconds to wait=u32 100) -> ()  [unwired: 1 out]
                    n689 = property on="倒计时开关" class="Bool (strict)"("Val(Sgnl)"=FALSE ("Value (Signaling)")) -> ()  [unwired: 2 in, 2 out]
                  }
                  frame #3 {
                    n690 = while {
                      shift-right: [w757] -> _
                      shift-left: 5.0 -> [w760]
                      stop <- w759 stop-if-true
                      n691 = Decrement(x=w760) -> (x-1=w757:dbl)
                      n692 = Wait (ms)(milliseconds to wait=u32 1000) -> ()  [unwired: 1 out]
                      n693 = property on="Countdow" class="DigNum (strict)"("Val(Sgnl)"=w757) -> ()  [unwired: 2 in, 2 out]
                      n694 = Less Or Equal To 0?(x=w757) -> (x <= 0?=w758:bool)
                      n695 = property on="倒计时开关" class="Bool (strict)"("Val(Sgnl)"=w758) -> ()  [unwired: 2 in, 2 out]
                      n696 = property on="倒计时开关" class="Bool (strict)"() -> ("Value"=w759:bool)  [unwired: 2 in, 2 out]
                    }
                    n697 = property on="Reminder Information" class="Str"("Val(Sgnl)"="Finish adjusting the substrate and Ga2 cell temperature." ("Value (Signaling)")) -> ()  [unwired: 2 in, 2 out]
                  }
                  frame #4 {
                    n698 = Wait (ms)(milliseconds to wait=u32 100) -> ()  [unwired: 1 out]
                    n699 = property on="倒计时开关" class="Bool (strict)"("Val(Sgnl)"=FALSE ("Value (Signaling)")) -> ()  [unwired: 2 in, 2 out]
                    n700 = property on="Ready for GaAs buffer 0.6 μm/h" class="Bool (strict)"("Val(Sgnl)"=FALSE ("Value (Signaling)")) -> ()  [unwired: 2 in, 2 out]
                  }
                }
                n701 = property on="Growth Switch" class="DigNum (strict)"() -> ("Value"=w719:i32)  [unwired: 2 in, 2 out]
                n702 = Increment(x=w719) -> (x+1=w720:i32)
                n703 = property on="Growth Switch" class="DigNum (strict)"("Val(Sgnl)"=w720) -> ()  [unwired: 2 in, 2 out]
              }
              frame 3 {
                n704 = flat-sequence "HT-GaAs 0.6 μm/h" {
                  frame #0 {
                    n705 = Wait (ms)(milliseconds to wait=u32 100) -> ()  [unwired: 1 out]
                    n706 = property on="倒计时开关" class="Bool (strict)"("Val(Sgnl)"=FALSE ("Value (Signaling)")) -> ()  [unwired: 2 in, 2 out]
                  }
                  frame #1 {
                    n707 = property on="nm" class="DigNum (strict)"() -> ("Value"=w769:u32)  [unwired: 2 in, 2 out]
                    n708 = Divide(x=0.6, y=3.6) -> (x/y=w771:dbl)
                    n709 = property on="As挡板" class="Bool (strict)"("Val(Sgnl)"=TRUE ("Value (Signaling)")) -> ()  [unwired: 2 in, 2 out]
                    n710 = property on="In挡板" class="Bool (strict)"("Val(Sgnl)"=FALSE ("Value (Signaling)")) -> ()  [unwired: 2 in, 2 out]
                    n711 = property on="GaAs buffer 0.6 μm/h" class="Bool (strict)"("Val(Sgnl)"=TRUE ("Value (Signaling)")) -> ()  [unwired: 2 in, 2 out]
                    n712 = property on="Ga2挡板" class="Bool (strict)"("Val(Sgnl)"=TRUE ("Value (Signaling)")) -> ()  [unwired: 2 in, 2 out]
                    n713 = property on="Main挡板" class="Bool (strict)"("Val(Sgnl)"=TRUE ("Value (Signaling)")) -> ()  [unwired: 2 in, 2 out]
                    n714 = Divide(x=w769, y=w771) -> (x/y=w770:dbl)
                    n715 = while {
                      shift-right: [w781] -> _
                      shift-left: w770 -> [w783]
                      stop <- w782 stop-if-true
                      n716 = Decrement(x=w783) -> (x-1=w781:dbl)
                      n717 = Wait (ms)(milliseconds to wait=u32 1000) -> ()  [unwired: 1 out]
                      n718 = property on="Countdow" class="DigNum (strict)"("Val(Sgnl)"=w781) -> ()  [unwired: 2 in, 2 out]
                      n719 = Less Or Equal To 0?(x=w781) -> (x <= 0?=w780:bool)
                      n720 = property on="倒计时开关" class="Bool (strict)"("Val(Sgnl)"=w780) -> ()  [unwired: 2 in, 2 out]
                      n721 = property on="倒计时开关" class="Bool (strict)"() -> ("Value"=w782:bool)  [unwired: 2 in, 2 out]
                    }
                    n722 = property on="Reminder Information" class="Str"("Val(Sgnl)"="Start the growth of GaAs buffer." ("Value (Signaling)")) -> ()  [unwired: 2 in, 2 out]
                  }
                  frame #2 {
                    n723 = Wait (ms)(milliseconds to wait=u32 100) -> ()  [unwired: 1 out]
                    n724 = property on="倒计时开关" class="Bool (strict)"("Val(Sgnl)"=FALSE ("Value (Signaling)")) -> ()  [unwired: 2 in, 2 out]
                  }
                  frame #3 {
                    n725 = property on="As挡板" class="Bool (strict)"("Val(Sgnl)"=TRUE ("Value (Signaling)")) -> ()  [unwired: 2 in, 2 out]
                    n726 = while {
                      shift-right: [w793] -> _
                      shift-left: 5.0 -> [w796]
                      stop <- w795 stop-if-true
                      n727 = Decrement(x=w796) -> (x-1=w793:dbl)
                      n728 = Wait (ms)(milliseconds to wait=u32 1000) -> ()  [unwired: 1 out]
                      n729 = property on="Countdow" class="DigNum (strict)"("Val(Sgnl)"=w793) -> ()  [unwired: 2 in, 2 out]
                      n730 = Less Or Equal To 0?(x=w793) -> (x <= 0?=w794:bool)
                      n731 = property on="倒计时开关" class="Bool (strict)"("Val(Sgnl)"=w794) -> ()  [unwired: 2 in, 2 out]
                      n732 = property on="倒计时开关" class="Bool (strict)"() -> ("Value"=w795:bool)  [unwired: 2 in, 2 out]
                    }
                    n733 = property on="In挡板" class="Bool (strict)"("Val(Sgnl)"=FALSE ("Value (Signaling)")) -> ()  [unwired: 2 in, 2 out]
                    n734 = property on="Main挡板" class="Bool (strict)"("Val(Sgnl)"=TRUE ("Value (Signaling)")) -> ()  [unwired: 2 in, 2 out]
                    n735 = property on="Ga2挡板" class="Bool (strict)"("Val(Sgnl)"=FALSE ("Value (Signaling)")) -> ()  [unwired: 2 in, 2 out]
                    n736 = property on="Reminder Information" class="Str"("Val(Sgnl)"="Finish the growth of GaAs buffer." ("Value (Signaling)")) -> ()  [unwired: 2 in, 2 out]
                  }
                  frame #4 {
                    n737 = Wait (ms)(milliseconds to wait=u32 100) -> ()  [unwired: 1 out]
                    n738 = property on="倒计时开关" class="Bool (strict)"("Val(Sgnl)"=FALSE ("Value (Signaling)")) -> ()  [unwired: 2 in, 2 out]
                    n739 = property on="GaAs buffer 0.6 μm/h" class="Bool (strict)"("Val(Sgnl)"=FALSE ("Value (Signaling)")) -> ()  [unwired: 2 in, 2 out]
                  }
                }
                n740 = property on="Growth Switch" class="DigNum (strict)"() -> ("Value"=w765:i32)  [unwired: 2 in, 2 out]
                n741 = Increment(x=w765) -> (x+1=w766:i32)
                n742 = property on="Growth Switch" class="DigNum (strict)"("Val(Sgnl)"=w766) -> ()  [unwired: 2 in, 2 out]
              }
              frame 4 {
                n743 = for {
                  N: w802 -> [_]
                  i -> [w806]
                  n744 = flat-sequence {
                    frame #0 {
                      n745 = flat-sequence "Inside InAs QDs" {
                        frame #0 {
                          n746 = Wait (ms)(milliseconds to wait=u32 100) -> ()  [unwired: 1 out]
                          n747 = property on="倒计时开关" class="Bool (strict)"("Val(Sgnl)"=FALSE ("Value (Signaling)")) -> ()  [unwired: 2 in, 2 out]
                        }
                        frame #1 {
                          n748 = flat-sequence {
                            tunnel: [w814] -> w810
                            tunnel: w810 -> [w826]
                            frame #0 {
                              n749 = property on="Sub实测" class="Str"() -> ("Value"=w819:string)  [unwired: 2 in, 2 out]
                              n750 = property on="Sub2" class="Str"() -> ("Value"=w825:string)  [unwired: 2 in, 2 out]
                              n751 = property on="倒计时开关" class="Bool (strict)"("Val(Sgnl)"=FALSE ("Value (Signaling)")) -> ()  [unwired: 2 in, 2 out]
                              n752 = property on="Optimize Sub Temperature 1" class="Str"("Val(Sgnl)"=w825) -> ()  [unwired: 2 in, 2 out]
                              n753 = Decimal String To Number(string=w819) -> (number=w818:i32)  [unwired: 2 in, 1 out]
                              n754 = Decimal String To Number(string=w825) -> (number=w821:i32)  [unwired: 2 in, 1 out]
                              n755 = Subtract(x=w818, y=w821) -> (x-y=w820:i32)
                              n756 = Absolute Value(x=w820) -> (abs(x)=w822:i32)
                              n757 = Divide(x=w822, y=10) -> (x/y=w823:dbl)
                              n758 = Add(x=w823, y=3.0) -> (x+y=w824:dbl)
                              n759 = Multiply(x=w824, y=60.0) -> (x*y=w814:dbl)
                            }
                            frame #1 {
                              n760 = while {
                                shift-right: [w829] -> _
                                shift-left: w826 -> [w831]
                                stop <- w830 stop-if-true
                                n761 = Decrement(x=w831) -> (x-1=w829:dbl)
                                n762 = Wait (ms)(milliseconds to wait=u32 1000) -> ()  [unwired: 1 out]
                                n763 = property on="Countdow" class="DigNum (strict)"("Val(Sgnl)"=w829) -> ()  [unwired: 2 in, 2 out]
                                n764 = Less Or Equal To 0?(x=w829) -> (x <= 0?=w828:bool)
                                n765 = property on="倒计时开关" class="Bool (strict)"("Val(Sgnl)"=w828) -> ()  [unwired: 2 in, 2 out]
                                n766 = property on="倒计时开关" class="Bool (strict)"() -> ("Value"=w830:bool)  [unwired: 2 in, 2 out]
                              }
                              n767 = property on="Sub2" class="Str"() -> ("Value"=w827:string)  [unwired: 2 in, 2 out]
                              n768 = property on="Sub设定" class="Str"("Val(Sgnl)"=w827) -> ()  [unwired: 2 in, 2 out]
                            }
                          }
                          n769 = property on="Ga2 2" class="Str"() -> ("Value"=w811:string)  [unwired: 2 in, 2 out]
                          n770 = property on="Temperature adjustment 1" class="Bool (strict)"("Val(Sgnl)"=TRUE ("Temperature adjustment 1")) -> ()  [unwired: 2 in, 2 out]
                          n771 = property on="Ga2设定" class="Str"("Val(Sgnl)"=w811) -> ()  [unwired: 2 in, 2 out]
                          n772 = property on="Reminder Information" class="Str"("Val(Sgnl)"="Start temperature adjustment, then manually adjust the As cracker needle valve." ("Value (Signaling)")) -> ()  [unwired: 2 in, 2 out]
                        }
                        frame #2 {
                          n773 = Wait (ms)(milliseconds to wait=u32 100) -> ()  [unwired: 1 out]
                          n774 = property on="倒计时开关" class="Bool (strict)"("Val(Sgnl)"=FALSE ("Value (Signaling)")) -> ()  [unwired: 2 in, 2 out]
                        }
                        frame #3 {
                          n775 = property on="Temperature adjustment 1" class="Bool (strict)"("Val(Sgnl)"=FALSE ("Temperature adjustment 1")) -> ()  [unwired: 2 in, 2 out]
                          n776 = while {
                            shift-right: [w839] -> _
                            shift-left: 5.0 -> [w841]
                            stop <- w840 stop-if-true
                            n777 = Decrement(x=w841) -> (x-1=w839:dbl)
                            n778 = property on="Countdow" class="DigNum (strict)"("Val(Sgnl)"=w839) -> ()  [unwired: 2 in, 2 out]
                            n779 = Less Or Equal To 0?(x=w839) -> (x <= 0?=w838:bool)
                            n780 = Wait (ms)(milliseconds to wait=u32 1000) -> ()  [unwired: 1 out]
                            n781 = property on="倒计时开关" class="Bool (strict)"("Val(Sgnl)"=w838) -> ()  [unwired: 2 in, 2 out]
                            n782 = property on="倒计时开关" class="Bool (strict)"() -> ("Value"=w840:bool)  [unwired: 2 in, 2 out]
                          }
                          n783 = property on="Reminder Information" class="Str"("Val(Sgnl)"="Finish temperature adjustment." ("Value (Signaling)")) -> ()  [unwired: 2 in, 2 out]
                        }
                        frame #4 {
                          n784 = Wait (ms)(milliseconds to wait=u32 100) -> ()  [unwired: 1 out]
                          n785 = property on="倒计时开关" class="Bool (strict)"("Val(Sgnl)"=FALSE ("Value (Signaling)")) -> ()  [unwired: 2 in, 2 out]
                        }
                      }
                    }
                    frame #1 {
                      n786 = flat-sequence "Overshoot" {
                        frame #0 {
                          n787 = property on="Main挡板" class="Bool (strict)"("Val(Sgnl)"=FALSE ("Value (Signaling)")) -> ()  [unwired: 2 in, 2 out]
                          n788 = property on="Inside InAs QDs" class="Bool (strict)"("Val(Sgnl)"=TRUE ("Value (Signaling)")) -> ()  [unwired: 2 in, 2 out]
                          n789 = property on="Ga2挡板" class="Bool (strict)"("Val(Sgnl)"=FALSE ("Value (Signaling)")) -> ()  [unwired: 2 in, 2 out]
                          n790 = while {
                            shift-right: [w852] -> _
                            shift-left: 4.0 -> [w855]
                            stop <- w854 stop-if-true
                            n791 = Decrement(x=w855) -> (x-1=w852:dbl)
                            n792 = Wait (ms)(milliseconds to wait=u32 1000) -> ()  [unwired: 1 out]
                            n793 = property on="Countdow" class="DigNum (strict)"("Val(Sgnl)"=w852) -> ()  [unwired: 2 in, 2 out]
                            n794 = Less Or Equal To 0?(x=w852) -> (x <= 0?=w853:bool)
                            n795 = property on="倒计时开关" class="Bool (strict)"("Val(Sgnl)"=w853) -> ()  [unwired: 2 in, 2 out]
                            n796 = property on="倒计时开关" class="Bool (strict)"() -> ("Value"=w854:bool)  [unwired: 2 in, 2 out]
                          }
                          n797 = property on="As挡板" class="Bool (strict)"("Val(Sgnl)"=TRUE ("Value (Signaling)")) -> ()  [unwired: 2 in, 2 out]
                          n798 = property on="In挡板" class="Bool (strict)"("Val(Sgnl)"=FALSE ("Value (Signaling)")) -> ()  [unwired: 2 in, 2 out]
                          n799 = property on="Reminder Information" class="Str"("Val(Sgnl)"="Start overshoot by 2 minutes." ("Value (Signaling)")) -> ()  [unwired: 2 in, 2 out]
                        }
                        frame #1 {
                          n800 = Wait (ms)(milliseconds to wait=u32 100) -> ()  [unwired: 1 out]
                          n801 = property on="倒计时开关" class="Bool (strict)"("Val(Sgnl)"=FALSE ("Value (Signaling)")) -> ()  [unwired: 2 in, 2 out]
                        }
                        frame #2 {
                          n802 = property on="As挡板" class="Bool (strict)"("Val(Sgnl)"=TRUE ("Value (Signaling)")) -> ()  [unwired: 2 in, 2 out]
                          n803 = while {
                            shift-right: [w864] -> _
                            shift-left: 4.0 -> [w867]
                            stop <- w866 stop-if-true
                            n804 = Decrement(x=w867) -> (x-1=w864:dbl)
                            n805 = property on="Countdow" class="DigNum (strict)"("Val(Sgnl)"=w864) -> ()  [unwired: 2 in, 2 out]
                            n806 = Wait (ms)(milliseconds to wait=u32 1000) -> ()  [unwired: 1 out]
                            n807 = Less Or Equal To 0?(x=w864) -> (x <= 0?=w865:bool)
                            n808 = property on="倒计时开关" class="Bool (strict)"("Val(Sgnl)"=w865) -> ()  [unwired: 2 in, 2 out]
                            n809 = property on="倒计时开关" class="Bool (strict)"() -> ("Value"=w866:bool)  [unwired: 2 in, 2 out]
                          }
                          n810 = property on="Main挡板" class="Bool (strict)"("Val(Sgnl)"=FALSE ("Value (Signaling)")) -> ()  [unwired: 2 in, 2 out]
                          n811 = property on="Ga2挡板" class="Bool (strict)"("Val(Sgnl)"=TRUE ("Value (Signaling)")) -> ()  [unwired: 2 in, 2 out]
                          n812 = property on="In挡板" class="Bool (strict)"("Val(Sgnl)"=TRUE ("Value (Signaling)")) -> ()  [unwired: 2 in, 2 out]
                        }
                        frame #3 {
                          n813 = Wait (ms)(milliseconds to wait=u32 100) -> ()  [unwired: 1 out]
                          n814 = property on="倒计时开关" class="Bool (strict)"("Val(Sgnl)"=FALSE ("Value (Signaling)")) -> ()  [unwired: 2 in, 2 out]
                        }
                        frame #4 {
                          n815 = while {
                            shift-right: [w872] -> _
                            shift-left: 120.0 -> [w876]
                            stop <- w875 stop-if-true
                            n816 = Decrement(x=w876) -> (x-1=w872:dbl)
                            n817 = property on="Countdow" class="DigNum (strict)"("Val(Sgnl)"=w872) -> ()  [unwired: 2 in, 2 out]
                            n818 = Wait (ms)(milliseconds to wait=u32 1000) -> ()  [unwired: 1 out]
                            n819 = Less?(x=w872, y=60.0) -> (x < y?=w874:bool)
                            n820 = property on="倒计时开关" class="Bool (strict)"("Val(Sgnl)"=w874) -> ()  [unwired: 2 in, 2 out]
                            n821 = property on="倒计时开关" class="Bool (strict)"() -> ("Value"=w875:bool)  [unwired: 2 in, 2 out]
                          }
                        }
                        frame #5 {
                          n822 = Wait (ms)(milliseconds to wait=u32 100) -> ()  [unwired: 1 out]
                          n823 = property on="倒计时开关" class="Bool (strict)"("Val(Sgnl)"=FALSE ("Value (Signaling)")) -> ()  [unwired: 2 in, 2 out]
                        }
                        frame #6 {
                          n824 = while {
                            shift-right: [w883] -> _
                            shift-left: 60.0 -> [w886]
                            stop <- w885 stop-if-true
                            n825 = Decrement(x=w886) -> (x-1=w883:dbl)
                            n826 = Wait (ms)(milliseconds to wait=u32 1000) -> ()  [unwired: 1 out]
                            n827 = property on="Countdow" class="DigNum (strict)"("Val(Sgnl)"=w883) -> ()  [unwired: 2 in, 2 out]
                            n828 = Less Or Equal To 0?(x=w883) -> (x <= 0?=w884:bool)
                            n829 = property on="倒计时开关" class="Bool (strict)"("Val(Sgnl)"=w884) -> ()  [unwired: 2 in, 2 out]
                            n830 = property on="倒计时开关" class="Bool (strict)"() -> ("Value"=w885:bool)  [unwired: 2 in, 2 out]
                          }
                          n831 = property on="摄像头开关" class="Bool (strict)"("Val(Sgnl)"=TRUE ("Value (Signaling)")) -> ()  [unwired: 2 in, 2 out]
                          n832 = property on="Reminder Information" class="Str"("Val(Sgnl)"="Please manually open the RHEED shutter." ("Value (Signaling)")) -> ()  [unwired: 2 in, 2 out]
                        }
                        frame #7 {
                          n833 = Wait (ms)(milliseconds to wait=u32 100) -> ()  [unwired: 1 out]
                          n834 = property on="倒计时开关" class="Bool (strict)"("Val(Sgnl)"=FALSE ("Value (Signaling)")) -> ()  [unwired: 2 in, 2 out]
                        }
                        frame #8 {
                          n835 = property on="As挡板" class="Bool (strict)"("Val(Sgnl)"=TRUE ("Value (Signaling)")) -> ()  [unwired: 2 in, 2 out]
                          n836 = while {
                            shift-right: [w895] -> _
                            shift-left: 4.0 -> [w898]
                            stop <- w897 stop-if-true
                            n837 = Decrement(x=w898) -> (x-1=w895:dbl)
                            n838 = Wait (ms)(milliseconds to wait=u32 1000) -> ()  [unwired: 1 out]
                            n839 = property on="Countdow" class="DigNum (strict)"("Val(Sgnl)"=w895) -> ()  [unwired: 2 in, 2 out]
                            n840 = Less Or Equal To 0?(x=w895) -> (x <= 0?=w896:bool)
                            n841 = property on="倒计时开关" class="Bool (strict)"("Val(Sgnl)"=w896) -> ()  [unwired: 2 in, 2 out]
                            n842 = property on="倒计时开关" class="Bool (strict)"() -> ("Value"=w897:bool)  [unwired: 2 in, 2 out]
                          }
                          n843 = property on="In挡板" class="Bool (strict)"("Val(Sgnl)"=FALSE ("Value (Signaling)")) -> ()  [unwired: 2 in, 2 out]
                          n844 = property on="Main挡板" class="Bool (strict)"("Val(Sgnl)"=FALSE ("Value (Signaling)")) -> ()  [unwired: 2 in, 2 out]
                          n845 = property on="Ga2挡板" class="Bool (strict)"("Val(Sgnl)"=FALSE ("Value (Signaling)")) -> ()  [unwired: 2 in, 2 out]
                        }
                        frame #9 {
                          n846 = Wait (ms)(milliseconds to wait=u32 100) -> ()  [unwired: 1 out]
                          n847 = property on="倒计时开关" class="Bool (strict)"("Val(Sgnl)"=FALSE ("Value (Signaling)")) -> ()  [unwired: 2 in, 2 out]
                        }
                        frame #10 {
                          n848 = property on="Model switch" class="Bool (strict)"("Val(Sgnl)"=TRUE ("Value (Signaling)")) -> ()  [unwired: 2 in, 2 out]
                          n849 = property on="Main挡板" class="Bool (strict)"("Val(Sgnl)"=TRUE ("Value (Signaling)")) -> ()  [unwired: 2 in, 2 out]
                          n850 = while {
                            shift-right: [w910] -> _
                            shift-left: 4.0 -> [w913]
                            stop <- w912 stop-if-true
                            n851 = Decrement(x=w913) -> (x-1=w910:dbl)
                            n852 = Wait (ms)(milliseconds to wait=u32 1000) -> ()  [unwired: 1 out]
                            n853 = property on="Countdow" class="DigNum (strict)"("Val(Sgnl)"=w910) -> ()  [unwired: 2 in, 2 out]
                            n854 = Less Or Equal To 0?(x=w910) -> (x <= 0?=w911:bool)
                            n855 = property on="倒计时开关" class="Bool (strict)"("Val(Sgnl)"=w911) -> ()  [unwired: 2 in, 2 out]
                            n856 = property on="记录Shutter模型的连续24个输出结果" class="Arr (strict)"("Val(Sgnl)"=u8[] [0, 0, 0, 0, 0, 0, 0, 0, 0, 0, 0, 0, 0, 0, 0, 0, 0, 0, 0, 0, 0, 0, 0, 0] ("initialized array")) -> ()  [unwired: 2 in, 2 out]
                            n857 = property on="倒计时开关" class="Bool (strict)"() -> ("Value"=w912:bool)  [unwired: 2 in, 2 out]
                          }
                          n858 = property on="Ga2挡板" class="Bool (strict)"("Val(Sgnl)"=FALSE ("Value (Signaling)")) -> ()  [unwired: 2 in, 2 out]
                          n859 = property on="As挡板" class="Bool (strict)"("Val(Sgnl)"=TRUE ("Value (Signaling)")) -> ()  [unwired: 2 in, 2 out]
                          n860 = property on="In挡板" class="Bool (strict)"("Val(Sgnl)"=FALSE ("Value (Signaling)")) -> ()  [unwired: 2 in, 2 out]
                          n861 = property on="Reminder Information" class="Str"("Val(Sgnl)"="Finish overshoot." ("Value (Signaling)")) -> ()  [unwired: 2 in, 2 out]
                        }
                        frame #11 {
                          n862 = Wait (ms)(milliseconds to wait=u32 100) -> ()  [unwired: 1 out]
                          n863 = property on="倒计时开关" class="Bool (strict)"("Val(Sgnl)"=FALSE ("Value (Signaling)")) -> ()  [unwired: 2 in, 2 out]
                        }
                      }
                    }
                    frame #2 {
                      n864 = flat-sequence "Inside InAs QDs" {
                        frame #0 {
                          n865 = property on="Sub速度" class="Str"("Val(Sgnl)"="5" ("Value (Signaling)")) -> ()  [unwired: 2 in, 2 out]
                          n866 = while {
                            shift-right: [w924] -> _
                            shift-left: 10.0 -> [w927]
                            stop <- w926 stop-if-true
                            n867 = Decrement(x=w927) -> (x-1=w924:dbl)
                            n868 = property on="Countdow" class="DigNum (strict)"("Val(Sgnl)"=w924) -> ()  [unwired: 2 in, 2 out]
                            n869 = Less Or Equal To 0?(x=w924) -> (x <= 0?=w925:bool)
                            n870 = Wait (ms)(milliseconds to wait=u32 1000) -> ()  [unwired: 1 out]
                            n871 = property on="倒计时开关" class="Bool (strict)"("Val(Sgnl)"=w925) -> ()  [unwired: 2 in, 2 out]
                            n872 = property on="倒计时开关" class="Bool (strict)"() -> ("Value"=w926:bool)  [unwired: 2 in, 2 out]
                          }
                          n873 = property on="As挡板" class="Bool (strict)"("Val(Sgnl)"=TRUE ("Value (Signaling)")) -> ()  [unwired: 2 in, 2 out]
                          n874 = property on="In挡板" class="Bool (strict)"("Val(Sgnl)"=TRUE ("Value (Signaling)")) -> ()  [unwired: 2 in, 2 out]
                          n875 = property on="Main挡板" class="Bool (strict)"("Val(Sgnl)"=TRUE ("Value (Signaling)")) -> ()  [unwired: 2 in, 2 out]
                          n876 = property on="Ga2挡板" class="Bool (strict)"("Val(Sgnl)"=FALSE ("Value (Signaling)")) -> ()  [unwired: 2 in, 2 out]
                          n877 = property on="Reminder Information" class="Str"("Val(Sgnl)"="Start growth of inside InAs QDs." ("Value (Signaling)")) -> ()  [unwired: 2 in, 2 out]
                        }
                        frame #1 {
                          n878 = while {
                            stop <- w929 stop-if-true
                            n879 = property on="模型输出是否超过0.7概率是Ys" class="Bool (strict)"() -> ("Value"=w930:bool)  [unwired: 2 in, 2 out]
                            n880 = case shown="True" w930 {
                              frame False {
                                n881 = property on="Temperature count result" class="DigNum (strict)"() -> ("Value"=w932:u8)  [unwired: 2 in, 2 out]
                                n882 = property on="If In Shutter can be closed 1" class="Bool (strict)"("Val(Sgnl)"=FALSE ("Value (Signaling)")) -> ()  [unwired: 2 in, 2 out]
                                n883 = case shown="1" w932 {
                                frame 0 {
                                n884 = flat-sequence {
                                frame #0 {
                                n885 = property on="Sub实测" class="Str"() -> ("Value"=w938:string)  [unwired: 2 in, 2 out]
                                n886 = Decimal String To Number(string=w938) -> (number=w936:i32)  [unwired: 2 in, 1 out]
                                n887 = Subtract(x=w936, y=2) -> (x-y=w934:i32)
                                n888 = Number To Decimal String(number=w934) -> (decimal integer string=w937:string)  [unwired: 1 in]
                                n889 = property on="Optimize Sub Temperature 1" class="Str"("Val(Sgnl)"=w937) -> ()  [unwired: 2 in, 2 out]
                                }
                                frame #1 {
                                n890 = property on="Optimize Sub Temperature 1" class="Str"() -> ("Value"=w939:string)  [unwired: 2 in, 2 out]
                                n891 = property on="Sub设定" class="Str"("Val(Sgnl)"=w939) -> ()  [unwired: 2 in, 2 out]
                                }
                                }
                                n892 = property on="Reminder Information" class="Str"("Val(Sgnl)"="Cool the substrate temperature." ("Value (Signaling)")) -> ()  [unwired: 2 in, 2 out]
                                }
                                frame 1 {
                                n893 = flat-sequence {
                                frame #0 {
                                n894 = property on="Sub实测" class="Str"() -> ("Value"=w945:string)  [unwired: 2 in, 2 out]
                                n895 = Decimal String To Number(string=w945) -> (number=w943:i32)  [unwired: 2 in, 1 out]
                                n896 = Add(x=w943, y=2) -> (x+y=w941:i32)
                                n897 = Number To Decimal String(number=w941) -> (decimal integer string=w944:string)  [unwired: 1 in]
                                n898 = property on="Optimize Sub Temperature 1" class="Str"("Val(Sgnl)"=w944) -> ()  [unwired: 2 in, 2 out]
                                }
                                frame #1 {
                                n899 = property on="Optimize Sub Temperature 1" class="Str"() -> ("Value"=w946:string)  [unwired: 2 in, 2 out]
                                n900 = property on="Sub设定" class="Str"("Val(Sgnl)"=w946) -> ()  [unwired: 2 in, 2 out]
                                }
                                }
                                n901 = property on="Reminder Information" class="Str"("Val(Sgnl)"="Heat up the substrate temperature." ("Value (Signaling)")) -> ()  [unwired: 2 in, 2 out]
                                }
                                frame 2, Default {
                                n902 = property on="Sub实测" class="Str"() -> ("Value"=w947:string)  [unwired: 2 in, 2 out]
                                n903 = property on="Sub设定" class="Str"("Val(Sgnl)"=w947) -> ()  [unwired: 2 in, 2 out]
                                n904 = property on="Optimize Sub Temperature 1" class="Str"("Val(Sgnl)"=w947) -> ()  [unwired: 2 in, 2 out]
                                n905 = property on="Reminder Information" class="Str"("Val(Sgnl)"="Maintain the substrate temperature." ("Value (Signaling)")) -> ()  [unwired: 2 in, 2 out]
                                }
                                }
                              }
                              frame True {
                                n906 = property on="Sub实测" class="Str"() -> ("Value"=w949:string)  [unwired: 2 in, 2 out]
                                n907 = while {
                                shift-right: [w957] -> _
                                shift-left: 5.0 -> [w960]
                                stop <- w959 stop-if-true
                                n908 = Decrement(x=w960) -> (x-1=w957:dbl)
                                n909 = property on="Countdow" class="DigNum (strict)"("Val(Sgnl)"=w957) -> ()  [unwired: 2 in, 2 out]
                                n910 = Wait (ms)(milliseconds to wait=u32 1000) -> ()  [unwired: 1 out]
                                n911 = Less Or Equal To 0?(x=w957) -> (x <= 0?=w958:bool)
                                n912 = property on="倒计时开关" class="Bool (strict)"("Val(Sgnl)"=w958) -> ()  [unwired: 2 in, 2 out]
                                n913 = property on="倒计时开关" class="Bool (strict)"() -> ("Value"=w959:bool)  [unwired: 2 in, 2 out]
                                }
                                n914 = property on="Main挡板" class="Bool (strict)"("Val(Sgnl)"=TRUE ("Value (Signaling)")) -> ()  [unwired: 2 in, 2 out]
                                n915 = property on="Sub2" class="Str"("Val(Sgnl)"=w949) -> ()  [unwired: 2 in, 2 out]
                                n916 = property on="Optimize Sub Temperature 1" class="Str"("Val(Sgnl)"=w949) -> ()  [unwired: 2 in, 2 out]
                                n917 = property on="Sub4" class="Str"("Val(Sgnl)"=w949) -> ()  [unwired: 2 in, 2 out]
                                n918 = property on="In挡板" class="Bool (strict)"("Val(Sgnl)"=FALSE ("Value (Signaling)")) -> ()  [unwired: 2 in, 2 out]
                                n919 = property on="As挡板" class="Bool (strict)"("Val(Sgnl)"=TRUE ("Value (Signaling)")) -> ()  [unwired: 2 in, 2 out]
                                n920 = property on="If In Shutter can be closed 1" class="Bool (strict)"("Val(Sgnl)"=TRUE ("Value (Signaling)")) -> ()  [unwired: 2 in, 2 out]
                                n921 = property on="Ga2挡板" class="Bool (strict)"("Val(Sgnl)"=FALSE ("Value (Signaling)")) -> ()  [unwired: 2 in, 2 out]
                                n922 = property on="Reminder Information" class="Str"("Val(Sgnl)"="Finish growth of inside InAs QDs." ("Value (Signaling)")) -> ()  [unwired: 2 in, 2 out]
                              }
                            }
                            n923 = property on="If In Shutter can be closed 1" class="Bool (strict)"() -> ("Value"=w929:bool)  [unwired: 2 in, 2 out]
                          }
                        }
                        frame #2 {
                          n924 = Wait (ms)(milliseconds to wait=u32 100) -> ()  [unwired: 1 out]
                          n925 = property on="摄像头开关" class="Bool (strict)"("Val(Sgnl)"=FALSE ("Value (Signaling)")) -> ()  [unwired: 2 in, 2 out]
                        }
                        frame #3 {
                          n926 = property on="Inside InAs QDs" class="Bool (strict)"("Val(Sgnl)"=FALSE ("Value (Signaling)")) -> ()  [unwired: 2 in, 2 out]
                          n927 = property on="If In Shutter can be closed 1" class="Bool (strict)"("Val(Sgnl)"=FALSE ("Value (Signaling)")) -> ()  [unwired: 2 in, 2 out]
                          n928 = property on="Sub速度" class="Str"("Val(Sgnl)"="10" ("Value (Signaling)")) -> ()  [unwired: 2 in, 2 out]
                          n929 = property on="模型输出是否超过0.7概率是Ys" class="Bool (strict)"("Val(Sgnl)"=FALSE ("Value (Signaling)")) -> ()  [unwired: 2 in, 2 out]
                          n930 = property on="Model switch" class="Bool (strict)"("Val(Sgnl)"=FALSE ("Value (Signaling)")) -> ()  [unwired: 2 in, 2 out]
                          n931 = while {
                            shift-right: [w972] -> _
                            shift-left: 5.0 -> [w975]
                            stop <- w974 stop-if-true
                            n932 = Decrement(x=w975) -> (x-1=w972:dbl)
                            n933 = Wait (ms)(milliseconds to wait=u32 1000) -> ()  [unwired: 1 out]
                            n934 = property on="Countdow" class="DigNum (strict)"("Val(Sgnl)"=w972) -> ()  [unwired: 2 in, 2 out]
                            n935 = Less Or Equal To 0?(x=w972) -> (x <= 0?=w973:bool)
                            n936 = property on="倒计时开关" class="Bool (strict)"("Val(Sgnl)"=w973) -> ()  [unwired: 2 in, 2 out]
                            n937 = property on="记录Shutter模型的连续24个输出结果" class="Arr (strict)"("Val(Sgnl)"=u8[] [0, 0, 0, 0, 0, 0, 0, 0, 0, 0, 0, 0, 0, 0, 0, 0, 0, 0, 0, 0, 0, 0, 0, 0] ("initialized array")) -> ()  [unwired: 2 in, 2 out]
                            n938 = property on="倒计时开关" class="Bool (strict)"() -> ("Value"=w974:bool)  [unwired: 2 in, 2 out]
                          }
                          n939 = property on="Reminder Information" class="Str"("Val(Sgnl)"="The RHEED shutter can now be closed." ("Value (Signaling)")) -> ()  [unwired: 2 in, 2 out]
                        }
                        frame #4 {
                          n940 = Wait (ms)(milliseconds to wait=u32 100) -> ()  [unwired: 1 out]
                          n941 = property on="摄像头开关" class="Bool (strict)"("Val(Sgnl)"=FALSE ("Value (Signaling)")) -> ()  [unwired: 2 in, 2 out]
                        }
                      }
                    }
                    frame #3 {
                      n942 = property on="repetition 1 LT-GaAs not do" class="Bool (strict)"() -> ("Value"=w979:bool)  [unwired: 2 in, 2 out]
                      n943 = case shown="True" w979 {
                        tunnel: [TRUE w984] -> w982
                        frame False {
                        }
                        frame True {
                          n944 = property on="Repetition" class="DigNum (strict)"() -> ("Value"=w986:i32)  [unwired: 2 in, 2 out]
                          n945 = Not Equal?(x=w986, y=1) -> (x != y?=w984:bool)
                        }
                      }
                      n946 = property on="10 nm LT-GaAs switch Yes is do" class="Bool (strict)"() -> ("Value"=w981:bool)  [unwired: 2 in, 2 out]
                      n947 = And(x=w981, y=w982) -> (x .and. y?=w980:bool)
                      n948 = case shown="True" w980 {
                        frame False {
                        }
                        frame True {
                          n949 = flat-sequence "10 nm LT-GaAs" {
                            frame #0 {
                              n950 = property on="10 nm GaAs cap layer 0.36 μm/h" class="Bool (strict)"("Val(Sgnl)"=TRUE ("Value (Signaling)")) -> ()  [unwired: 2 in, 2 out]
                              n951 = while {
                                shift-right: [w990] -> _
                                shift-left: 5.0 -> [w993]
                                stop <- w992 stop-if-true
                                n952 = Decrement(x=w993) -> (x-1=w990:dbl)
                                n953 = property on="Countdow" class="DigNum (strict)"("Val(Sgnl)"=w990) -> ()  [unwired: 2 in, 2 out]
                                n954 = Less Or Equal To 0?(x=w990) -> (x <= 0?=w991:bool)
                                n955 = Wait (ms)(milliseconds to wait=u32 1000) -> ()  [unwired: 1 out]
                                n956 = property on="倒计时开关" class="Bool (strict)"("Val(Sgnl)"=w991) -> ()  [unwired: 2 in, 2 out]
                                n957 = property on="倒计时开关" class="Bool (strict)"() -> ("Value"=w992:bool)  [unwired: 2 in, 2 out]
                              }
                              n958 = property on="Reminder Information" class="Str"("Val(Sgnl)"="Manually adjust the As cracker needle valve." ("Value (Signaling)")) -> ()  [unwired: 2 in, 2 out]
                            }
                            frame #1 {
                              n959 = Wait (ms)(milliseconds to wait=u32 100) -> ()  [unwired: 1 out]
                              n960 = property on="倒计时开关" class="Bool (strict)"("Val(Sgnl)"=FALSE ("Value (Signaling)")) -> ()  [unwired: 2 in, 2 out]
                            }
                            frame #2 {
                              n961 = property on="In挡板" class="Bool (strict)"("Val(Sgnl)"=FALSE ("Value (Signaling)")) -> ()  [unwired: 2 in, 2 out]
                              n962 = property on="Main挡板" class="Bool (strict)"("Val(Sgnl)"=TRUE ("Value (Signaling)")) -> ()  [unwired: 2 in, 2 out]
                              n963 = property on="As挡板" class="Bool (strict)"("Val(Sgnl)"=TRUE ("Value (Signaling)")) -> ()  [unwired: 2 in, 2 out]
                              n964 = property on="Ga2挡板" class="Bool (strict)"("Val(Sgnl)"=TRUE ("Value (Signaling)")) -> ()  [unwired: 2 in, 2 out]
                              n965 = Divide(x=0.36, y=3.6) -> (x/y=w1006:dbl)
                              n966 = Divide(x=10.0, y=w1006) -> (x/y=w1005:dbl)
                              n967 = while {
                                shift-right: [w1008] -> _
                                shift-left: w1005 -> [w1010]
                                stop <- w1009 stop-if-true
                                n968 = Decrement(x=w1010) -> (x-1=w1008:dbl)
                                n969 = property on="Countdow" class="DigNum (strict)"("Val(Sgnl)"=w1008) -> ()  [unwired: 2 in, 2 out]
                                n970 = Less Or Equal To 0?(x=w1008) -> (x <= 0?=w1007:bool)
                                n971 = Wait (ms)(milliseconds to wait=u32 1000) -> ()  [unwired: 1 out]
                                n972 = property on="倒计时开关" class="Bool (strict)"("Val(Sgnl)"=w1007) -> ()  [unwired: 2 in, 2 out]
                                n973 = property on="倒计时开关" class="Bool (strict)"() -> ("Value"=w1009:bool)  [unwired: 2 in, 2 out]
                              }
                              n974 = property on="Reminder Information" class="Str"("Val(Sgnl)"="Start the growth of GaAs cap layer." ("Value (Signaling)")) -> ()  [unwired: 2 in, 2 out]
                            }
                            frame #3 {
                              n975 = Wait (ms)(milliseconds to wait=u32 100) -> ()  [unwired: 1 out]
                              n976 = property on="倒计时开关" class="Bool (strict)"("Val(Sgnl)"=FALSE ("Value (Signaling)")) -> ()  [unwired: 2 in, 2 out]
                            }
                            frame #4 {
                              n977 = property on="Main挡板" class="Bool (strict)"("Val(Sgnl)"=TRUE ("Value (Signaling)")) -> ()  [unwired: 2 in, 2 out]
                              n978 = property on="10 nm GaAs cap layer 0.36 μm/h" class="Bool (strict)"("Val(Sgnl)"=FALSE ("Value (Signaling)")) -> ()  [unwired: 2 in, 2 out]
                              n979 = property on="In挡板" class="Bool (strict)"("Val(Sgnl)"=FALSE ("Value (Signaling)")) -> ()  [unwired: 2 in, 2 out]
                              n980 = while {
                                shift-right: [w1021] -> _
                                shift-left: 5.0 -> [w1024]
                                stop <- w1023 stop-if-true
                                n981 = Decrement(x=w1024) -> (x-1=w1021:dbl)
                                n982 = Wait (ms)(milliseconds to wait=u32 1000) -> ()  [unwired: 1 out]
                                n983 = property on="Countdow" class="DigNum (strict)"("Val(Sgnl)"=w1021) -> ()  [unwired: 2 in, 2 out]
                                n984 = Less Or Equal To 0?(x=w1021) -> (x <= 0?=w1022:bool)
                                n985 = property on="倒计时开关" class="Bool (strict)"("Val(Sgnl)"=w1022) -> ()  [unwired: 2 in, 2 out]
                                n986 = property on="倒计时开关" class="Bool (strict)"() -> ("Value"=w1023:bool)  [unwired: 2 in, 2 out]
                              }
                              n987 = property on="As挡板" class="Bool (strict)"("Val(Sgnl)"=TRUE ("Value (Signaling)")) -> ()  [unwired: 2 in, 2 out]
                              n988 = property on="Ga2挡板" class="Bool (strict)"("Val(Sgnl)"=FALSE ("Value (Signaling)")) -> ()  [unwired: 2 in, 2 out]
                              n989 = property on="Reminder Information" class="Str"("Val(Sgnl)"="Finish the growth of GaAs cap layer." ("Value (Signaling)")) -> ()  [unwired: 2 in, 2 out]
                            }
                            frame #5 {
                              n990 = Wait (ms)(milliseconds to wait=u32 100) -> ()  [unwired: 1 out]
                              n991 = property on="倒计时开关" class="Bool (strict)"("Val(Sgnl)"=FALSE ("Value (Signaling)")) -> ()  [unwired: 2 in, 2 out]
                            }
                          }
                        }
                      }
                    }
                    frame #4 {
                      n992 = flat-sequence "temperature adjustment," {
                        frame #0 {
                          n993 = property on="Ga2 3" class="Str"() -> ("Value"=w1030:string)  [unwired: 2 in, 2 out]
                          n994 = flat-sequence {
                            tunnel: [w1032] -> w1031
                            tunnel: w1031 -> [w1044]
                            frame #0 {
                              n995 = property on="Sub实测" class="Str"() -> ("Value"=w1037:string)  [unwired: 2 in, 2 out]
                              n996 = property on="Sub3" class="Str"() -> ("Value"=w1043:string)  [unwired: 2 in, 2 out]
                              n997 = Decimal String To Number(string=w1037) -> (number=w1036:i32)  [unwired: 2 in, 1 out]
                              n998 = Decimal String To Number(string=w1043) -> (number=w1039:i32)  [unwired: 2 in, 1 out]
                              n999 = Subtract(x=w1036, y=w1039) -> (x-y=w1038:i32)
                              n1000 = Absolute Value(x=w1038) -> (abs(x)=w1040:i32)
                              n1001 = Divide(x=w1040, y=10) -> (x/y=w1041:dbl)
                              n1002 = Add(x=w1041, y=3.0) -> (x+y=w1042:dbl)
                              n1003 = Multiply(x=w1042, y=60.0) -> (x*y=w1032:dbl)
                            }
                            frame #1 {
                              n1004 = property on="Sub3" class="Str"() -> ("Value"=w1045:string)  [unwired: 2 in, 2 out]
                              n1005 = while {
                                shift-right: [w1047] -> _
                                shift-left: w1044 -> [w1049]
                                stop <- w1048 stop-if-true
                                n1006 = Decrement(x=w1049) -> (x-1=w1047:dbl)
                                n1007 = property on="Countdow" class="DigNum (strict)"("Val(Sgnl)"=w1047) -> ()  [unwired: 2 in, 2 out]
                                n1008 = Less Or Equal To 0?(x=w1047) -> (x <= 0?=w1046:bool)
                                n1009 = Wait (ms)(milliseconds to wait=u32 1000) -> ()  [unwired: 1 out]
                                n1010 = property on="倒计时开关" class="Bool (strict)"("Val(Sgnl)"=w1046) -> ()  [unwired: 2 in, 2 out]
                                n1011 = property on="倒计时开关" class="Bool (strict)"() -> ("Value"=w1048:bool)  [unwired: 2 in, 2 out]
                              }
                              n1012 = property on="Sub设定" class="Str"("Val(Sgnl)"=w1045) -> ()  [unwired: 2 in, 2 out]
                            }
                          }
                          n1013 = property on="Ga2设定" class="Str"("Val(Sgnl)"=w1030) -> ()  [unwired: 2 in, 2 out]
                          n1014 = property on="Temperature adjustment 2" class="Bool (strict)"("Val(Sgnl)"=TRUE ("Temperature adjustment 1")) -> ()  [unwired: 2 in, 2 out]
                          n1015 = property on="Reminder Information" class="Str"("Val(Sgnl)"="Start temperature adjustment, then manually adjust the As cracker needle valve." ("Value (Signaling)")) -> ()  [unwired: 2 in, 2 out]
                        }
                        frame #1 {
                          n1016 = Wait (ms)(milliseconds to wait=u32 100) -> ()  [unwired: 1 out]
                          n1017 = property on="倒计时开关" class="Bool (strict)"("Val(Sgnl)"=FALSE ("Value (Signaling)")) -> ()  [unwired: 2 in, 2 out]
                        }
                        frame #2 {
                          n1018 = property on="Temperature adjustment 2" class="Bool (strict)"("Val(Sgnl)"=FALSE ("Temperature adjustment 1")) -> ()  [unwired: 2 in, 2 out]
                          n1019 = while {
                            shift-right: [w1057] -> _
                            shift-left: 5.0 -> [w1059]
                            stop <- w1058 stop-if-true
                            n1020 = Decrement(x=w1059) -> (x-1=w1057:dbl)
                            n1021 = property on="Countdow" class="DigNum (strict)"("Val(Sgnl)"=w1057) -> ()  [unwired: 2 in, 2 out]
                            n1022 = Wait (ms)(milliseconds to wait=u32 1000) -> ()  [unwired: 1 out]
                            n1023 = Less Or Equal To 0?(x=w1057) -> (x <= 0?=w1056:bool)
                            n1024 = property on="倒计时开关" class="Bool (strict)"("Val(Sgnl)"=w1056) -> ()  [unwired: 2 in, 2 out]
                            n1025 = property on="倒计时开关" class="Bool (strict)"() -> ("Value"=w1058:bool)  [unwired: 2 in, 2 out]
                          }
                          n1026 = property on="Reminder Information" class="Str"("Val(Sgnl)"="Finish temperature adjustment." ("Value (Signaling)")) -> ()  [unwired: 2 in, 2 out]
                        }
                        frame #3 {
                          n1027 = Wait (ms)(milliseconds to wait=u32 100) -> ()  [unwired: 1 out]
                          n1028 = property on="倒计时开关" class="Bool (strict)"("Val(Sgnl)"=FALSE ("Value (Signaling)")) -> ()  [unwired: 2 in, 2 out]
                        }
                      }
                    }
                    frame #5 {
                      n1029 = flat-sequence "HT-GaAs 0.6 μm/h" {
                        frame #0 {
                          n1030 = property on="nm 2" class="DigNum (strict)"() -> ("Value"=w1064:u32)  [unwired: 2 in, 2 out]
                          n1031 = Divide(x=0.6, y=3.6) -> (x/y=w1066:dbl)
                          n1032 = Divide(x=w1064, y=w1066) -> (x/y=w1065:dbl)
                          n1033 = property on="As挡板" class="Bool (strict)"("Val(Sgnl)"=TRUE ("Value (Signaling)")) -> ()  [unwired: 2 in, 2 out]
                          n1034 = property on="In挡板" class="Bool (strict)"("Val(Sgnl)"=FALSE ("Value (Signaling)")) -> ()  [unwired: 2 in, 2 out]
                          n1035 = property on="GaAs buffer 0.6 μm/h  2" class="Bool (strict)"("Val(Sgnl)"=TRUE ("Value (Signaling)")) -> ()  [unwired: 2 in, 2 out]
                          n1036 = property on="Ga2挡板" class="Bool (strict)"("Val(Sgnl)"=TRUE ("Value (Signaling)")) -> ()  [unwired: 2 in, 2 out]
                          n1037 = property on="Main挡板" class="Bool (strict)"("Val(Sgnl)"=TRUE ("Value (Signaling)")) -> ()  [unwired: 2 in, 2 out]
                          n1038 = while {
                            shift-right: [w1075] -> _
                            shift-left: w1065 -> [w1077]
                            stop <- w1076 stop-if-true
                            n1039 = Decrement(x=w1077) -> (x-1=w1075:dbl)
                            n1040 = property on="Countdow" class="DigNum (strict)"("Val(Sgnl)"=w1075) -> ()  [unwired: 2 in, 2 out]
                            n1041 = Less Or Equal To 0?(x=w1075) -> (x <= 0?=w1074:bool)
                            n1042 = Wait (ms)(milliseconds to wait=u32 1000) -> ()  [unwired: 1 out]
                            n1043 = property on="倒计时开关" class="Bool (strict)"("Val(Sgnl)"=w1074) -> ()  [unwired: 2 in, 2 out]
                            n1044 = property on="倒计时开关" class="Bool (strict)"() -> ("Value"=w1076:bool)  [unwired: 2 in, 2 out]
                          }
                          n1045 = property on="Reminder Information" class="Str"("Val(Sgnl)"="Start the growth of GaAs buffer." ("Value (Signaling)")) -> ()  [unwired: 2 in, 2 out]
                        }
                        frame #1 {
                          n1046 = Wait (ms)(milliseconds to wait=u32 100) -> ()  [unwired: 1 out]
                          n1047 = property on="倒计时开关" class="Bool (strict)"("Val(Sgnl)"=FALSE ("Value (Signaling)")) -> ()  [unwired: 2 in, 2 out]
                        }
                        frame #2 {
                          n1048 = property on="As挡板" class="Bool (strict)"("Val(Sgnl)"=TRUE ("Value (Signaling)")) -> ()  [unwired: 2 in, 2 out]
                          n1049 = while {
                            shift-right: [w1087] -> _
                            shift-left: 5.0 -> [w1090]
                            stop <- w1089 stop-if-true
                            n1050 = Decrement(x=w1090) -> (x-1=w1087:dbl)
                            n1051 = property on="Countdow" class="DigNum (strict)"("Val(Sgnl)"=w1087) -> ()  [unwired: 2 in, 2 out]
                            n1052 = Less Or Equal To 0?(x=w1087) -> (x <= 0?=w1088:bool)
                            n1053 = Wait (ms)(milliseconds to wait=u32 1000) -> ()  [unwired: 1 out]
                            n1054 = property on="倒计时开关" class="Bool (strict)"("Val(Sgnl)"=w1088) -> ()  [unwired: 2 in, 2 out]
                            n1055 = property on="倒计时开关" class="Bool (strict)"() -> ("Value"=w1089:bool)  [unwired: 2 in, 2 out]
                          }
                          n1056 = property on="In挡板" class="Bool (strict)"("Val(Sgnl)"=FALSE ("Value (Signaling)")) -> ()  [unwired: 2 in, 2 out]
                          n1057 = property on="Main挡板" class="Bool (strict)"("Val(Sgnl)"=TRUE ("Value (Signaling)")) -> ()  [unwired: 2 in, 2 out]
                          n1058 = property on="Ga2挡板" class="Bool (strict)"("Val(Sgnl)"=FALSE ("Value (Signaling)")) -> ()  [unwired: 2 in, 2 out]
                          n1059 = property on="Reminder Information" class="Str"("Val(Sgnl)"="Finish the growth of GaAs buffer." ("Value (Signaling)")) -> ()  [unwired: 2 in, 2 out]
                        }
                        frame #3 {
                          n1060 = Wait (ms)(milliseconds to wait=u32 100) -> ()  [unwired: 1 out]
                          n1061 = property on="倒计时开关" class="Bool (strict)"("Val(Sgnl)"=FALSE ("Value (Signaling)")) -> ()  [unwired: 2 in, 2 out]
                          n1062 = property on="GaAs buffer 0.6 μm/h  2" class="Bool (strict)"("Val(Sgnl)"=FALSE ("Value (Signaling)")) -> ()  [unwired: 2 in, 2 out]
                        }
                      }
                    }
                  }
                  n1063 = Increment(x=w806) -> (x+1=w805:i32)
                  n1064 = property on="Repetition" class="DigNum (strict)"("Val(Sgnl)"=w805) -> ()  [unwired: 2 in, 2 out]
                }
                n1065 = property on="Growth Switch" class="DigNum (strict)"() -> ("Value"=w803:i32)  [unwired: 2 in, 2 out]
                n1066 = Increment(x=w803) -> (x+1=w804:i32)
                n1067 = property on="Growth Switch" class="DigNum (strict)"("Val(Sgnl)"=w804) -> ()  [unwired: 2 in, 2 out]
                n1068 = property on="Tab Control" class="TabCtl (strict)"("Val(Sgnl)"=T1."InAs/GaAs QDs on GaAs substrates" ("Value (Signaling)")) -> ()  [unwired: 2 in, 2 out]
              }
              frame 5 {
                n1069 = property on="Growth Switch" class="DigNum (strict)"() -> ("Value"=w1096:i32)  [unwired: 2 in, 2 out]
                n1070 = property on="Surface InAs QDs" class="Bool (strict)"() -> ("Value"=w1095:bool)  [unwired: 2 in, 2 out]
                n1071 = Increment(x=w1096) -> (x+1=w1097:i32)
                n1072 = property on="Growth Switch" class="DigNum (strict)"("Val(Sgnl)"=w1097) -> ()  [unwired: 2 in, 2 out]
                n1073 = case shown="True" w1095 {
                  frame False {
                  }
                  frame True {
                    n1074 = flat-sequence {
                      frame #0 {
                        n1075 = flat-sequence "Surface InAs QDs" {
                          frame #0 {
                            n1076 = Wait (ms)(milliseconds to wait=u32 100) -> ()  [unwired: 1 out]
                            n1077 = property on="Repetition" class="DigNum (strict)"("Val(Sgnl)"=0 ("Value (Signaling)")) -> ()  [unwired: 2 in, 2 out]
                            n1078 = property on="倒计时开关" class="Bool (strict)"("Val(Sgnl)"=FALSE ("Value (Signaling)")) -> ()  [unwired: 2 in, 2 out]
                          }
                          frame #1 {
                            n1079 = flat-sequence {
                              tunnel: [w1106] -> w1104
                              tunnel: w1104 -> [w1117]
                              frame #0 {
                                n1080 = property on="Sub实测" class="Str"() -> ("Value"=w1111:string)  [unwired: 2 in, 2 out]
                                n1081 = property on="Sub4" class="Str"() -> ("Value"=w1105:string)  [unwired: 2 in, 2 out]
                                n1082 = property on="Optimize Sub Temperature 2" class="Str"("Val(Sgnl)"=w1105) -> ()  [unwired: 2 in, 2 out]
                                n1083 = Decimal String To Number(string=w1111) -> (number=w1110:i32)  [unwired: 2 in, 1 out]
                                n1084 = Decimal String To Number(string=w1105) -> (number=w1113:i32)  [unwired: 2 in, 1 out]
                                n1085 = Subtract(x=w1110, y=w1113) -> (x-y=w1112:i32)
                                n1086 = Absolute Value(x=w1112) -> (abs(x)=w1114:i32)
                                n1087 = Divide(x=w1114, y=10) -> (x/y=w1115:dbl)
                                n1088 = Add(x=w1115, y=3.0) -> (x+y=w1116:dbl)
                                n1089 = Multiply(x=w1116, y=60.0) -> (x*y=w1106:dbl)
                              }
                              frame #1 {
                                n1090 = property on="Sub2" class="Str"() -> ("Value"=w1118:string)  [unwired: 2 in, 2 out]
                                n1091 = while {
                                shift-right: [w1120] -> _
                                shift-left: w1117 -> [w1122]
                                stop <- w1121 stop-if-true
                                n1092 = Decrement(x=w1122) -> (x-1=w1120:dbl)
                                n1093 = property on="Countdow" class="DigNum (strict)"("Val(Sgnl)"=w1120) -> ()  [unwired: 2 in, 2 out]
                                n1094 = Less Or Equal To 0?(x=w1120) -> (x <= 0?=w1119:bool)
                                n1095 = Wait (ms)(milliseconds to wait=u32 1000) -> ()  [unwired: 1 out]
                                n1096 = property on="倒计时开关" class="Bool (strict)"("Val(Sgnl)"=w1119) -> ()  [unwired: 2 in, 2 out]
                                n1097 = property on="倒计时开关" class="Bool (strict)"() -> ("Value"=w1121:bool)  [unwired: 2 in, 2 out]
                                }
                                n1098 = property on="Sub设定" class="Str"("Val(Sgnl)"=w1118) -> ()  [unwired: 2 in, 2 out]
                              }
                            }
                            n1099 = property on="Ga2 4" class="Str"() -> ("Value"=w1102:string)  [unwired: 2 in, 2 out]
                            n1100 = property on="Temperature adjustment 3" class="Bool (strict)"("Val(Sgnl)"=TRUE ("Temperature adjustment 1")) -> ()  [unwired: 2 in, 2 out]
                            n1101 = property on="Ga2设定" class="Str"("Val(Sgnl)"=w1102) -> ()  [unwired: 2 in, 2 out]
                            n1102 = property on="Reminder Information" class="Str"("Val(Sgnl)"="Start temperature adjustment, then manually adjust the As cracker needle valve." ("Value (Signaling)")) -> ()  [unwired: 2 in, 2 out]
                          }
                          frame #2 {
                            n1103 = Wait (ms)(milliseconds to wait=u32 100) -> ()  [unwired: 1 out]
                            n1104 = property on="倒计时开关" class="Bool (strict)"("Val(Sgnl)"=FALSE ("Value (Signaling)")) -> ()  [unwired: 2 in, 2 out]
                          }
                          frame #3 {
                            n1105 = property on="Temperature adjustment 3" class="Bool (strict)"("Val(Sgnl)"=FALSE ("Temperature adjustment 1")) -> ()  [unwired: 2 in, 2 out]
                            n1106 = while {
                              shift-right: [w1130] -> _
                              shift-left: 5.0 -> [w1132]
                              stop <- w1131 stop-if-true
                              n1107 = Decrement(x=w1132) -> (x-1=w1130:dbl)
                              n1108 = Wait (ms)(milliseconds to wait=u32 1000) -> ()  [unwired: 1 out]
                              n1109 = property on="Countdow" class="DigNum (strict)"("Val(Sgnl)"=w1130) -> ()  [unwired: 2 in, 2 out]
                              n1110 = Less Or Equal To 0?(x=w1130) -> (x <= 0?=w1129:bool)
                              n1111 = property on="倒计时开关" class="Bool (strict)"("Val(Sgnl)"=w1129) -> ()  [unwired: 2 in, 2 out]
                              n1112 = property on="倒计时开关" class="Bool (strict)"() -> ("Value"=w1131:bool)  [unwired: 2 in, 2 out]
                            }
                            n1113 = property on="Reminder Information" class="Str"("Val(Sgnl)"="Finish temperature adjustment." ("Value (Signaling)")) -> ()  [unwired: 2 in, 2 out]
                          }
                          frame #4 {
                            n1114 = Wait (ms)(milliseconds to wait=u32 100) -> ()  [unwired: 1 out]
                            n1115 = property on="倒计时开关" class="Bool (strict)"("Val(Sgnl)"=FALSE ("Value (Signaling)")) -> ()  [unwired: 2 in, 2 out]
                          }
                        }
                      }
                      frame #1 {
                        n1116 = flat-sequence "Overshoot" {
                          frame #0 {
                            n1117 = property on="Main挡板" class="Bool (strict)"("Val(Sgnl)"=FALSE ("Value (Signaling)")) -> ()  [unwired: 2 in, 2 out]
                            n1118 = property on="Surface InAs QDs for AFM" class="Bool (strict)"("Val(Sgnl)"=TRUE ("Value (Signaling)")) -> ()  [unwired: 2 in, 2 out]
                            n1119 = property on="In挡板" class="Bool (strict)"("Val(Sgnl)"=FALSE ("Value (Signaling)")) -> ()  [unwired: 2 in, 2 out]
                            n1120 = while {
                              shift-right: [w1143] -> _
                              shift-left: 4.0 -> [w1146]
                              stop <- w1145 stop-if-true
                              n1121 = Decrement(x=w1146) -> (x-1=w1143:dbl)
                              n1122 = property on="Countdow" class="DigNum (strict)"("Val(Sgnl)"=w1143) -> ()  [unwired: 2 in, 2 out]
                              n1123 = Less Or Equal To 0?(x=w1143) -> (x <= 0?=w1144:bool)
                              n1124 = Wait (ms)(milliseconds to wait=u32 1000) -> ()  [unwired: 1 out]
                              n1125 = property on="倒计时开关" class="Bool (strict)"("Val(Sgnl)"=w1144) -> ()  [unwired: 2 in, 2 out]
                              n1126 = property on="倒计时开关" class="Bool (strict)"() -> ("Value"=w1145:bool)  [unwired: 2 in, 2 out]
                            }
                            n1127 = property on="Ga2挡板" class="Bool (strict)"("Val(Sgnl)"=FALSE ("Value (Signaling)")) -> ()  [unwired: 2 in, 2 out]
                            n1128 = property on="As挡板" class="Bool (strict)"("Val(Sgnl)"=TRUE ("Value (Signaling)")) -> ()  [unwired: 2 in, 2 out]
                            n1129 = property on="Reminder Information" class="Str"("Val(Sgnl)"="Start overshoot by 2 minutes." ("Value (Signaling)")) -> ()  [unwired: 2 in, 2 out]
                          }
                          frame #1 {
                            n1130 = Wait (ms)(milliseconds to wait=u32 100) -> ()  [unwired: 1 out]
                            n1131 = property on="倒计时开关" class="Bool (strict)"("Val(Sgnl)"=FALSE ("Value (Signaling)")) -> ()  [unwired: 2 in, 2 out]
                          }
                          frame #2 {
                            n1132 = property on="As挡板" class="Bool (strict)"("Val(Sgnl)"=TRUE ("Value (Signaling)")) -> ()  [unwired: 2 in, 2 out]
                            n1133 = while {
                              shift-right: [w1155] -> _
                              shift-left: 4.0 -> [w1158]
                              stop <- w1157 stop-if-true
                              n1134 = Decrement(x=w1158) -> (x-1=w1155:dbl)
                              n1135 = property on="Countdow" class="DigNum (strict)"("Val(Sgnl)"=w1155) -> ()  [unwired: 2 in, 2 out]
                              n1136 = Less Or Equal To 0?(x=w1155) -> (x <= 0?=w1156:bool)
                              n1137 = Wait (ms)(milliseconds to wait=u32 1000) -> ()  [unwired: 1 out]
                              n1138 = property on="倒计时开关" class="Bool (strict)"("Val(Sgnl)"=w1156) -> ()  [unwired: 2 in, 2 out]
                              n1139 = property on="倒计时开关" class="Bool (strict)"() -> ("Value"=w1157:bool)  [unwired: 2 in, 2 out]
                            }
                            n1140 = property on="Main挡板" class="Bool (strict)"("Val(Sgnl)"=FALSE ("Value (Signaling)")) -> ()  [unwired: 2 in, 2 out]
                            n1141 = property on="Ga2挡板" class="Bool (strict)"("Val(Sgnl)"=TRUE ("Value (Signaling)")) -> ()  [unwired: 2 in, 2 out]
                            n1142 = property on="In挡板" class="Bool (strict)"("Val(Sgnl)"=TRUE ("Value (Signaling)")) -> ()  [unwired: 2 in, 2 out]
                          }
                          frame #3 {
                            n1143 = Wait (ms)(milliseconds to wait=u32 100) -> ()  [unwired: 1 out]
                            n1144 = property on="倒计时开关" class="Bool (strict)"("Val(Sgnl)"=FALSE ("Value (Signaling)")) -> ()  [unwired: 2 in, 2 out]
                          }
                          frame #4 {
                            n1145 = while {
                              shift-right: [w1165] -> _
                              shift-left: 120.0 -> [w1167]
                              stop <- w1166 stop-if-true
                              n1146 = Decrement(x=w1167) -> (x-1=w1165:dbl)
                              n1147 = property on="Countdow" class="DigNum (strict)"("Val(Sgnl)"=w1165) -> ()  [unwired: 2 in, 2 out]
                              n1148 = Wait (ms)(milliseconds to wait=u32 1000) -> ()  [unwired: 1 out]
                              n1149 = Less?(x=w1165, y=60.0) -> (x < y?=w1163:bool)
                              n1150 = property on="倒计时开关" class="Bool (strict)"("Val(Sgnl)"=w1163) -> ()  [unwired: 2 in, 2 out]
                              n1151 = property on="倒计时开关" class="Bool (strict)"() -> ("Value"=w1166:bool)  [unwired: 2 in, 2 out]
                            }
                          }
                          frame #5 {
                            n1152 = Wait (ms)(milliseconds to wait=u32 100) -> ()  [unwired: 1 out]
                            n1153 = property on="倒计时开关" class="Bool (strict)"("Val(Sgnl)"=FALSE ("Value (Signaling)")) -> ()  [unwired: 2 in, 2 out]
                          }
                          frame #6 {
                            n1154 = while {
                              shift-right: [w1174] -> _
                              shift-left: 60.0 -> [w1177]
                              stop <- w1176 stop-if-true
                              n1155 = Decrement(x=w1177) -> (x-1=w1174:dbl)
                              n1156 = Wait (ms)(milliseconds to wait=u32 1000) -> ()  [unwired: 1 out]
                              n1157 = property on="Countdow" class="DigNum (strict)"("Val(Sgnl)"=w1174) -> ()  [unwired: 2 in, 2 out]
                              n1158 = Less Or Equal To 0?(x=w1174) -> (x <= 0?=w1175:bool)
                              n1159 = property on="倒计时开关" class="Bool (strict)"("Val(Sgnl)"=w1175) -> ()  [unwired: 2 in, 2 out]
                              n1160 = property on="倒计时开关" class="Bool (strict)"() -> ("Value"=w1176:bool)  [unwired: 2 in, 2 out]
                            }
                            n1161 = property on="摄像头开关" class="Bool (strict)"("Val(Sgnl)"=TRUE ("Value (Signaling)")) -> ()  [unwired: 2 in, 2 out]
                            n1162 = property on="Reminder Information" class="Str"("Val(Sgnl)"="Please manually open the RHEED shutter." ("Value (Signaling)")) -> ()  [unwired: 2 in, 2 out]
                          }
                          frame #7 {
                            n1163 = Wait (ms)(milliseconds to wait=u32 100) -> ()  [unwired: 1 out]
                            n1164 = property on="倒计时开关" class="Bool (strict)"("Val(Sgnl)"=FALSE ("Value (Signaling)")) -> ()  [unwired: 2 in, 2 out]
                          }
                          frame #8 {
                            n1165 = property on="As挡板" class="Bool (strict)"("Val(Sgnl)"=TRUE ("Value (Signaling)")) -> ()  [unwired: 2 in, 2 out]
                            n1166 = while {
                              shift-right: [w1186] -> _
                              shift-left: 4.0 -> [w1189]
                              stop <- w1188 stop-if-true
                              n1167 = Decrement(x=w1189) -> (x-1=w1186:dbl)
                              n1168 = property on="Countdow" class="DigNum (strict)"("Val(Sgnl)"=w1186) -> ()  [unwired: 2 in, 2 out]
                              n1169 = Wait (ms)(milliseconds to wait=u32 1000) -> ()  [unwired: 1 out]
                              n1170 = Less Or Equal To 0?(x=w1186) -> (x <= 0?=w1187:bool)
                              n1171 = property on="倒计时开关" class="Bool (strict)"("Val(Sgnl)"=w1187) -> ()  [unwired: 2 in, 2 out]
                              n1172 = property on="倒计时开关" class="Bool (strict)"() -> ("Value"=w1188:bool)  [unwired: 2 in, 2 out]
                            }
                            n1173 = property on="In挡板" class="Bool (strict)"("Val(Sgnl)"=FALSE ("Value (Signaling)")) -> ()  [unwired: 2 in, 2 out]
                            n1174 = property on="Main挡板" class="Bool (strict)"("Val(Sgnl)"=FALSE ("Value (Signaling)")) -> ()  [unwired: 2 in, 2 out]
                            n1175 = property on="Ga2挡板" class="Bool (strict)"("Val(Sgnl)"=FALSE ("Value (Signaling)")) -> ()  [unwired: 2 in, 2 out]
                          }
                          frame #9 {
                            n1176 = Wait (ms)(milliseconds to wait=u32 100) -> ()  [unwired: 1 out]
                            n1177 = property on="倒计时开关" class="Bool (strict)"("Val(Sgnl)"=FALSE ("Value (Signaling)")) -> ()  [unwired: 2 in, 2 out]
                          }
                          frame #10 {
                            n1178 = property on="Ga2挡板" class="Bool (strict)"("Val(Sgnl)"=FALSE ("Value (Signaling)")) -> ()  [unwired: 2 in, 2 out]
                            n1179 = property on="As挡板" class="Bool (strict)"("Val(Sgnl)"=TRUE ("Value (Signaling)")) -> ()  [unwired: 2 in, 2 out]
                            n1180 = while {
                              shift-right: [w1201] -> _
                              shift-left: 4.0 -> [w1204]
                              stop <- w1203 stop-if-true
                              n1181 = Decrement(x=w1204) -> (x-1=w1201:dbl)
                              n1182 = Wait (ms)(milliseconds to wait=u32 1000) -> ()  [unwired: 1 out]
                              n1183 = property on="Countdow" class="DigNum (strict)"("Val(Sgnl)"=w1201) -> ()  [unwired: 2 in, 2 out]
                              n1184 = Less Or Equal To 0?(x=w1201) -> (x <= 0?=w1202:bool)
                              n1185 = property on="倒计时开关" class="Bool (strict)"("Val(Sgnl)"=w1202) -> ()  [unwired: 2 in, 2 out]
                              n1186 = property on="记录Shutter模型的连续24个输出结果" class="Arr (strict)"("Val(Sgnl)"=u8[] [0, 0, 0, 0, 0, 0, 0, 0, 0, 0, 0, 0, 0, 0, 0, 0, 0, 0, 0, 0, 0, 0, 0, 0] ("initialized array")) -> ()  [unwired: 2 in, 2 out]
                              n1187 = property on="倒计时开关" class="Bool (strict)"() -> ("Value"=w1203:bool)  [unwired: 2 in, 2 out]
                            }
                            n1188 = property on="Model switch" class="Bool (strict)"("Val(Sgnl)"=TRUE ("Value (Signaling)")) -> ()  [unwired: 2 in, 2 out]
                            n1189 = property on="Main挡板" class="Bool (strict)"("Val(Sgnl)"=TRUE ("Value (Signaling)")) -> ()  [unwired: 2 in, 2 out]
                            n1190 = property on="In挡板" class="Bool (strict)"("Val(Sgnl)"=FALSE ("Value (Signaling)")) -> ()  [unwired: 2 in, 2 out]
                            n1191 = property on="Reminder Information" class="Str"("Val(Sgnl)"="Finish overshoot." ("Value (Signaling)")) -> ()  [unwired: 2 in, 2 out]
                          }
                          frame #11 {
                            n1192 = Wait (ms)(milliseconds to wait=u32 100) -> ()  [unwired: 1 out]
                            n1193 = property on="倒计时开关" class="Bool (strict)"("Val(Sgnl)"=FALSE ("Value (Signaling)")) -> ()  [unwired: 2 in, 2 out]
                          }
                        }
                      }
                      frame #2 {
                        n1194 = flat-sequence "Inside InAs QDs" {
                          frame #0 {
                            n1195 = property on="As挡板" class="Bool (strict)"("Val(Sgnl)"=TRUE ("Value (Signaling)")) -> ()  [unwired: 2 in, 2 out]
                            n1196 = while {
                              shift-right: [w1215] -> _
                              shift-left: 10.0 -> [w1218]
                              stop <- w1217 stop-if-true
                              n1197 = Decrement(x=w1218) -> (x-1=w1215:dbl)
                              n1198 = property on="Countdow" class="DigNum (strict)"("Val(Sgnl)"=w1215) -> ()  [unwired: 2 in, 2 out]
                              n1199 = Wait (ms)(milliseconds to wait=u32 1000) -> ()  [unwired: 1 out]
                              n1200 = Less Or Equal To 0?(x=w1215) -> (x <= 0?=w1216:bool)
                              n1201 = property on="倒计时开关" class="Bool (strict)"("Val(Sgnl)"=w1216) -> ()  [unwired: 2 in, 2 out]
                              n1202 = property on="倒计时开关" class="Bool (strict)"() -> ("Value"=w1217:bool)  [unwired: 2 in, 2 out]
                            }
                            n1203 = property on="Sub速度" class="Str"("Val(Sgnl)"="5" ("Value (Signaling)")) -> ()  [unwired: 2 in, 2 out]
                            n1204 = property on="Main挡板" class="Bool (strict)"("Val(Sgnl)"=TRUE ("Value (Signaling)")) -> ()  [unwired: 2 in, 2 out]
                            n1205 = property on="Ga2挡板" class="Bool (strict)"("Val(Sgnl)"=FALSE ("Value (Signaling)")) -> ()  [unwired: 2 in, 2 out]
                            n1206 = property on="In挡板" class="Bool (strict)"("Val(Sgnl)"=TRUE ("Value (Signaling)")) -> ()  [unwired: 2 in, 2 out]
                            n1207 = property on="Reminder Information" class="Str"("Val(Sgnl)"="Start growth of surface InAs QDs." ("Value (Signaling)")) -> ()  [unwired: 2 in, 2 out]
                          }
                          frame #1 {
                            n1208 = while {
                              stop <- w1220 stop-if-true
                              n1209 = property on="模型输出是否超过0.7概率是Ys" class="Bool (strict)"() -> ("Value"=w1221:bool)  [unwired: 2 in, 2 out]
                              n1210 = case shown="True" w1221 {
                                frame False {
                                n1211 = property on="If In Shutter can be closed 2" class="Bool (strict)"("Val(Sgnl)"=FALSE ("Value (Signaling)")) -> ()  [unwired: 2 in, 2 out]
                                n1212 = property on="Temperature count result" class="DigNum (strict)"() -> ("Value"=w1223:u8)  [unwired: 2 in, 2 out]
                                n1213 = case shown="1" w1223 {
                                frame 0 {
                                n1214 = flat-sequence {
                                frame #0 {
                                n1215 = property on="Sub实测" class="Str"() -> ("Value"=w1229:string)  [unwired: 2 in, 2 out]
                                n1216 = Decimal String To Number(string=w1229) -> (number=w1227:i32)  [unwired: 2 in, 1 out]
                                n1217 = Subtract(x=w1227, y=2) -> (x-y=w1225:i32)
                                n1218 = Number To Decimal String(number=w1225) -> (decimal integer string=w1228:string)  [unwired: 1 in]
                                n1219 = property on="Optimize Sub Temperature 2" class="Str"("Val(Sgnl)"=w1228) -> ()  [unwired: 2 in, 2 out]
                                }
                                frame #1 {
                                n1220 = property on="Optimize Sub Temperature 2" class="Str"() -> ("Value"=w1230:string)  [unwired: 2 in, 2 out]
                                n1221 = property on="Sub设定" class="Str"("Val(Sgnl)"=w1230) -> ()  [unwired: 2 in, 2 out]
                                }
                                }
                                n1222 = property on="Reminder Information" class="Str"("Val(Sgnl)"="Cool the substrate temperature." ("Value (Signaling)")) -> ()  [unwired: 2 in, 2 out]
                                }
                                frame 1 {
                                n1223 = flat-sequence {
                                frame #0 {
                                n1224 = property on="Sub实测" class="Str"() -> ("Value"=w1236:string)  [unwired: 2 in, 2 out]
                                n1225 = Decimal String To Number(string=w1236) -> (number=w1234:i32)  [unwired: 2 in, 1 out]
                                n1226 = Add(x=w1234, y=2) -> (x+y=w1232:i32)
                                n1227 = Number To Decimal String(number=w1232) -> (decimal integer string=w1235:string)  [unwired: 1 in]
                                n1228 = property on="Optimize Sub Temperature 2" class="Str"("Val(Sgnl)"=w1235) -> ()  [unwired: 2 in, 2 out]
                                }
                                frame #1 {
                                n1229 = property on="Optimize Sub Temperature 2" class="Str"() -> ("Value"=w1237:string)  [unwired: 2 in, 2 out]
                                n1230 = property on="Sub设定" class="Str"("Val(Sgnl)"=w1237) -> ()  [unwired: 2 in, 2 out]
                                }
                                }
                                n1231 = property on="Reminder Information" class="Str"("Val(Sgnl)"="Heat up the substrate temperature." ("Value (Signaling)")) -> ()  [unwired: 2 in, 2 out]
                                }
                                frame 2, Default {
                                n1232 = property on="Sub实测" class="Str"() -> ("Value"=w1238:string)  [unwired: 2 in, 2 out]
                                n1233 = property on="Sub设定" class="Str"("Val(Sgnl)"=w1238) -> ()  [unwired: 2 in, 2 out]
                                n1234 = property on="Optimize Sub Temperature 2" class="Str"("Val(Sgnl)"=w1238) -> ()  [unwired: 2 in, 2 out]
                                n1235 = property on="Reminder Information" class="Str"("Val(Sgnl)"="Maintain the substrate temperature." ("Value (Signaling)")) -> ()  [unwired: 2 in, 2 out]
                                }
                                }
                                }
                                frame True {
                                n1236 = property on="Sub实测" class="Str"() -> ("Value"=w1240:string)  [unwired: 2 in, 2 out]
                                n1237 = property on="As挡板" class="Bool (strict)"("Val(Sgnl)"=TRUE ("Value (Signaling)")) -> ()  [unwired: 2 in, 2 out]
                                n1238 = property on="If In Shutter can be closed 2" class="Bool (strict)"("Val(Sgnl)"=TRUE ("Value (Signaling)")) -> ()  [unwired: 2 in, 2 out]
                                n1239 = property on="Sub4" class="Str"("Val(Sgnl)"=w1240) -> ()  [unwired: 2 in, 2 out]
                                n1240 = property on="In挡板" class="Bool (strict)"("Val(Sgnl)"=FALSE ("Value (Signaling)")) -> ()  [unwired: 2 in, 2 out]
                                n1241 = property on="Main挡板" class="Bool (strict)"("Val(Sgnl)"=TRUE ("Value (Signaling)")) -> ()  [unwired: 2 in, 2 out]
                                n1242 = property on="Ga2挡板" class="Bool (strict)"("Val(Sgnl)"=FALSE ("Value (Signaling)")) -> ()  [unwired: 2 in, 2 out]
                                n1243 = property on="Reminder Information" class="Str"("Val(Sgnl)"="Finish growth of surface InAs QDs." ("Value (Signaling)")) -> ()  [unwired: 2 in, 2 out]
                                }
                              }
                              n1244 = property on="If In Shutter can be closed 2" class="Bool (strict)"() -> ("Value"=w1220:bool)  [unwired: 2 in, 2 out]
                            }
                          }
                          frame #2 {
                            n1245 = Wait (ms)(milliseconds to wait=u32 100) -> ()  [unwired: 1 out]
                            n1246 = property on="摄像头开关" class="Bool (strict)"("Val(Sgnl)"=FALSE ("Value (Signaling)")) -> ()  [unwired: 2 in, 2 out]
                          }
                          frame #3 {
                            n1247 = property on="Surface InAs QDs for AFM" class="Bool (strict)"("Val(Sgnl)"=FALSE ("Value (Signaling)")) -> ()  [unwired: 2 in, 2 out]
                            n1248 = property on="Sub速度" class="Str"("Val(Sgnl)"="10" ("Value (Signaling)")) -> ()  [unwired: 2 in, 2 out]
                            n1249 = property on="Model switch" class="Bool (strict)"("Val(Sgnl)"=FALSE ("Value (Signaling)")) -> ()  [unwired: 2 in, 2 out]
                            n1250 = property on="If In Shutter can be closed 2" class="Bool (strict)"("Val(Sgnl)"=FALSE ("Value (Signaling)")) -> ()  [unwired: 2 in, 2 out]
                            n1251 = while {
                              shift-right: [w1256] -> _
                              shift-left: 5.0 -> [w1259]
                              stop <- w1258 stop-if-true
                              n1252 = Decrement(x=w1259) -> (x-1=w1256:dbl)
                              n1253 = Wait (ms)(milliseconds to wait=u32 1000) -> ()  [unwired: 1 out]
                              n1254 = property on="Countdow" class="DigNum (strict)"("Val(Sgnl)"=w1256) -> ()  [unwired: 2 in, 2 out]
                              n1255 = Less Or Equal To 0?(x=w1256) -> (x <= 0?=w1257:bool)
                              n1256 = property on="倒计时开关" class="Bool (strict)"("Val(Sgnl)"=w1257) -> ()  [unwired: 2 in, 2 out]
                              n1257 = property on="记录Shutter模型的连续24个输出结果" class="Arr (strict)"("Val(Sgnl)"=u8[] [0, 0, 0, 0, 0, 0, 0, 0, 0, 0, 0, 0, 0, 0, 0, 0, 0, 0, 0, 0, 0, 0, 0, 0] ("initialized array")) -> ()  [unwired: 2 in, 2 out]
                              n1258 = property on="倒计时开关" class="Bool (strict)"() -> ("Value"=w1258:bool)  [unwired: 2 in, 2 out]
                            }
                            n1259 = property on="Reminder Information" class="Str"("Val(Sgnl)"="The RHEED shutter can now be closed." ("Value (Signaling)")) -> ()  [unwired: 2 in, 2 out]
                          }
                          frame #4 {
                            n1260 = Wait (ms)(milliseconds to wait=u32 100) -> ()  [unwired: 1 out]
                            n1261 = property on="摄像头开关" class="Bool (strict)"("Val(Sgnl)"=FALSE ("Value (Signaling)")) -> ()  [unwired: 2 in, 2 out]
                          }
                        }
                      }
                    }
                  }
                }
              }
              frame 6 {
                n1262 = flat-sequence "Ready" {
                  frame #0 {
                    n1263 = Wait (ms)(milliseconds to wait=u32 100) -> ()  [unwired: 1 out]
                    n1264 = property on="倒计时开关" class="Bool (strict)"("Val(Sgnl)"=FALSE ("Value (Signaling)")) -> ()  [unwired: 2 in, 2 out]
                  }
                  frame #1 {
                    n1265 = property on="Sub5" class="Str"() -> ("Value"=w1268:string)  [unwired: 2 in, 2 out]
                    n1266 = property on="Ga2挡板" class="Bool (strict)"("Val(Sgnl)"=FALSE ("Value (Signaling)")) -> ()  [unwired: 2 in, 2 out]
                    n1267 = while {
                      shift-right: [w1275] -> _
                      shift-left: 5.0 -> [w1277]
                      stop <- w1276 stop-if-true
                      n1268 = Decrement(x=w1277) -> (x-1=w1275:dbl)
                      n1269 = Wait (ms)(milliseconds to wait=u32 1000) -> ()  [unwired: 1 out]
                      n1270 = property on="Countdow" class="DigNum (strict)"("Val(Sgnl)"=w1275) -> ()  [unwired: 2 in, 2 out]
                      n1271 = Less Or Equal To 0?(x=w1275) -> (x <= 0?=w1274:bool)
                      n1272 = property on="倒计时开关" class="Bool (strict)"("Val(Sgnl)"=w1274) -> ()  [unwired: 2 in, 2 out]
                      n1273 = property on="倒计时开关" class="Bool (strict)"() -> ("Value"=w1276:bool)  [unwired: 2 in, 2 out]
                    }
                    n1274 = property on="In挡板" class="Bool (strict)"("Val(Sgnl)"=FALSE ("Value (Signaling)")) -> ()  [unwired: 2 in, 2 out]
                    n1275 = property on="Sub设定" class="Str"("Val(Sgnl)"=w1268) -> ()  [unwired: 2 in, 2 out]
                    n1276 = property on="As挡板" class="Bool (strict)"("Val(Sgnl)"=TRUE ("Value (Signaling)")) -> ()  [unwired: 2 in, 2 out]
                    n1277 = property on="Main挡板" class="Bool (strict)"("Val(Sgnl)"=TRUE ("Value (Signaling)")) -> ()  [unwired: 2 in, 2 out]
                    n1278 = property on="Reminder Information" class="Str"("Val(Sgnl)"="Start substrate cooling." ("Value (Signaling)")) -> ()  [unwired: 2 in, 2 out]
                  }
                  frame #2 {
                    n1279 = property on="Start" class="Bool (strict)"("Val(Sgnl)"=FALSE ("Value (Signaling)")) -> ()  [unwired: 2 in, 2 out]
                    n1280 = property on="倒计时开关" class="Bool (strict)"("Val(Sgnl)"=FALSE ("Value (Signaling)")) -> ()  [unwired: 2 in, 2 out]
                  }
                }
                n1281 = property on="Growth Switch" class="DigNum (strict)"() -> ("Value"=w1263:i32)  [unwired: 2 in, 2 out]
                n1282 = Increment(x=w1263) -> (x+1=w1264:i32)
                n1283 = property on="Growth Switch" class="DigNum (strict)"("Val(Sgnl)"=w1264) -> ()  [unwired: 2 in, 2 out]
              }
            }
          }
        }
      }
    }
  }
  n1284 = flat-sequence {
    tunnel: [w1281] -> w62
    tunnel: w62 -> [w1300]
    frame #0 {
      n1285 = Wait (ms)(milliseconds to wait=u32 5000 ("等待时间（毫秒）")) -> ()  [unwired: 1 out]
      n1286 = Get Date/Time In Seconds() -> (seconds since 1Jan1904=w1293:timestamp)
      n1287 = Format Date/Time String(time format string (%c)="%Y%m%d%H%M", seconds (now)=w1293) -> (date/time string=w1294:string)  [unwired: 1 in]
      n1288 = Current VI's Path() -> (path=w1288:path)
      n1289 = Strip Path(path=w1288) -> (stripped path=w1289:path)  [unwired: 1 out]
      n1290 = Search/Split String(string=w1294, search string/char (-)=".") -> (substring before match=w1296:string, match + rest of string=w1295:string)  [unwired: 1 in, 1 out]
      n1291 = Path To String(path=w1289) -> (string=w1290:string)
      n1292 = String Subset(string=w1295, offset (0)=1) -> (substring=w1297:string)  [unwired: 1 in]
      n1293 = Concatenate Strings(w1290, "\\Real time storage Excel\\" ("时间格式字符串(%c)")) -> (w1291:string)
      n1294 = Concatenate Strings(w1296, w1297) -> (w1298:string)
      n1295 = String To Path(string=w1291) -> (path=w1292:path)
      n1296 = Concatenate Strings(w1298, "Excel data storage.xls" ("时间格式字符串(%c)")) -> (w1287:string)
      n1297 = Build Path(base path=w1292, name or relative path=w1287) -> (appended path=w1281:path)
    }
    frame #1 {
      n1298 = while {
        tunnel: w1300 -> [w1562]
        stop <- FALSE stop-if-true
        n1299 = Wait (ms)(milliseconds to wait=u32 125 ("等待时间（毫秒）")) -> ()  [unwired: 1 out]
        n1300 = property on="0 Growth真空度（字符串）" class="Str"() -> ("Value"=w1570:string)  [unwired: 2 in, 2 out]
        n1301 = property on="0 Buffer真空度(字符串)" class="Str"() -> ("Value"=w1569:string)  [unwired: 2 in, 2 out]
        n1302 = Format Date/Time String(time format string (%c)="%Y/%m/%d/-%H:%M:%S" ("时间格式字符串(%c)")) -> (date/time string=w1571:string)  [unwired: 2 in]
        n1303 = property on="摄像头选择" class="IMAQdx (strict)"() -> ("Value"=w1543:T3)  [unwired: 2 in, 2 out]
        n1304 = property on="Is the probability of the model output deoxidization exceeding" class="Bool (strict)"() -> ("Value"=w1534:bool)  [unwired: 2 in, 2 out]
        n1305 = property on="Main挡板" class="Bool (strict)"() -> ("Value"=w1553:bool)  [unwired: 2 in, 2 out]
        n1306 = property on="Sub实测" class="Str"() -> ("Value"=w1568:string)  [unwired: 2 in, 2 out]
        n1307 = property on="Sub程序" class="Str"() -> ("Value"=w1567:string)  [unwired: 2 in, 2 out]
        n1308 = property on="Sub设定" class="Str"() -> ("Value"=w1566:string)  [unwired: 2 in, 2 out]
        n1309 = property on="Sub速度" class="Str"() -> ("Value"=w1565:string)  [unwired: 2 in, 2 out]
        n1310 = property on="Ga2实测" class="Str"() -> ("Value"=w1561:string)  [unwired: 2 in, 2 out]
        n1311 = property on="Ga2程序" class="Str"() -> ("Value"=w1560:string)  [unwired: 2 in, 2 out]
        n1312 = property on="Ga2设定" class="Str"() -> ("Value"=w1559:string)  [unwired: 2 in, 2 out]
        n1313 = property on="Ga2速度" class="Str"() -> ("Value"=w1558:string)  [unwired: 2 in, 2 out]
        n1314 = property on="Ga2挡板" class="Bool (strict)"() -> ("Value"=w1552:bool)  [unwired: 2 in, 2 out]
        n1315 = property on="As挡板" class="Bool (strict)"() -> ("Value"=w1550:bool)  [unwired: 2 in, 2 out]
        n1316 = property on="In设定" class="Str"() -> ("Value"=w1557:string)  [unwired: 2 in, 2 out]
        n1317 = property on="In实测" class="Str"() -> ("Value"=w1556:string)  [unwired: 2 in, 2 out]
        n1318 = property on="In程序" class="Str"() -> ("Value"=w1555:string)  [unwired: 2 in, 2 out]
        n1319 = property on="In速度" class="Str"() -> ("Value"=w1554:string)  [unwired: 2 in, 2 out]
        n1320 = property on="In挡板" class="Bool (strict)"() -> ("Value"=w1551:bool)  [unwired: 2 in, 2 out]
        n1321 = property on="Substrate to find Reconstruction temperature" class="Str"() -> ("Value"=w1525:string)  [unwired: 2 in, 2 out]
        n1322 = property on="Cool to less than 100 ℃ and wait 20 minutes" class="Bool (strict)"() -> ("Value"=w1527:bool)  [unwired: 2 in, 2 out]
        n1323 = property on="Substrate to find Deoxidation temperature" class="Str"() -> ("Value"=w1536:string)  [unwired: 2 in, 2 out]
        n1324 = property on="Whether to continue heating up operation" class="Bool (strict)"() -> ("Value"=w1535:bool)  [unwired: 2 in, 2 out]
        n1325 = property on="Obtaining the reconstruction  temperature" class="Bool (strict)"() -> ("Value"=w1526:bool)  [unwired: 2 in, 2 out]
        n1326 = property on="Reminder Information" class="Str"() -> ("Value"=w1545:string)  [unwired: 2 in, 2 out]
        n1327 = property on="Heating to completely remove oxidation" class="Bool (strict)"() -> ("Value"=w1532:bool)  [unwired: 2 in, 2 out]
        n1328 = property on="Obtaining the deoxidation temperature" class="Bool (strict)"() -> ("Value"=w1537:bool)  [unwired: 2 in, 2 out]
        n1329 = property on="Model switch" class="Bool (strict)"() -> ("Value"=w1547:bool)  [unwired: 2 in, 2 out]
        n1330 = property on="Ready for GaAs buffer 0.6 μm/h" class="Bool (strict)"() -> ("Value"=w1514:bool)  [unwired: 2 in, 2 out]
        n1331 = property on="Tab Control" class="TabCtl (strict)"() -> ("Value"=w1541:T1)  [unwired: 2 in, 2 out]
        n1332 = property on="摄像头开关" class="Bool (strict)"() -> ("Value"=w1548:bool)  [unwired: 2 in, 2 out]
        n1333 = property on="Countdow" class="DigNum (strict)"() -> ("Value"=w1546:u16)  [unwired: 2 in, 2 out]
        n1334 = property on="Obtain Growth Temperature" class="Bool (strict)"() -> ("Value"=w1521:bool)  [unwired: 2 in, 2 out]
        n1335 = property on="Reconstruction模型输出结果" class="Str"() -> ("Value"=w1538:string)  [unwired: 2 in, 2 out]
        n1336 = Format Into String "左上"(format string="%s\\t%s\\t%s\\t%s\\t%s\\t%s\\t%s\\t%s\\t%s\\t%s\\t%s\\t%s\\t%s\\t%s\\t%s\\t%s\\t%s\\t%s\\t%s\\t%s\\t%s\\t%s\\t%s\\t%s\\t%s\\t%s\\t%s\\t%s\\t%s\\t%s\\t%s\\t%g\\t%s\\t%g\\t%s\\t%g\\t%s\\t%g\\t" ("格式字符串"), "Time", w1571, "0 Growth真空度（字符串）", w1570, "0 Buffer真空度(字符串)", w1569, "Sub实测", w1568, "Sub程序", w1567, "Sub设定", w1566, "Sub速度", w1565, "Ga2实测", w1561, "Ga2程序", w1560, "Ga2设定", w1559, "Ga2速度", w1558, "In设定", w1557, "In实测", w1556, "In程序", w1555, "In速度", w1554, "Main挡板", w1553, "Ga2挡板", w1552, "In挡板", w1551, "As挡板", w1550) -> (resulting string=w1436:string)  [unwired: 2 in, 1 out]
        n1337 = property on="GaAs growth temperature" class="Str"() -> ("Value"=w1515:string)  [unwired: 2 in, 2 out]
        n1338 = Format Into String(w1543) -> (resulting string=w1542:string)  [unwired: 3 in, 1 out]
        n1339 = property on="Deoxidation temperature" class="Str"() -> ("Value"=w1533:string)  [unwired: 2 in, 2 out]
        n1340 = property on="InAs growth temperature" class="Str"() -> ("Value"=w1516:string)  [unwired: 2 in, 2 out]
        n1341 = property on="From As cap to c(4×4)" class="Str"() -> ("Value"=w1524:string)  [unwired: 2 in, 2 out]
        n1342 = property on="GaAs buffer 0.6 μm/h" class="Bool (strict)"() -> ("Value"=w1511:bool)  [unwired: 2 in, 2 out]
        n1343 = property on="GaAs buffer 0.6 μm/h" class="Bool (strict)"() -> ("Value"=w1529:bool)  [unwired: 2 in, 2 out]
        n1344 = property on="From c(4×4) to (2×4)" class="Str"() -> ("Value"=w1523:string)  [unwired: 2 in, 2 out]
        n1345 = property on="From (2×4) to (n×6)" class="Str"() -> ("Value"=w1522:string)  [unwired: 2 in, 2 out]
        n1346 = Format Into String(format string="%s\\t%s\\t%s\\t%g\\t%s\\t%g\\t%s\\t%d\\t%s\\t%s\\t" ("格式字符串"), initial string=w1436, "摄像头选择", w1542, "摄像头开关", w1548, "Model switch", w1547, "Countdow", w1546, "Reminder Information", w1545) -> (resulting string=w1435:string)  [unwired: 1 in, 1 out]
        n1347 = Format Into String(w1541) -> (resulting string=w1540:string)  [unwired: 3 in, 1 out]
        n1348 = property on="MSE loss" class="Str"() -> ("Value"=w1517:string)  [unwired: 2 in, 2 out]
        n1349 = property on="Sub1 2" class="Str"() -> ("Value"=w1531:string)  [unwired: 2 in, 2 out]
        n1350 = property on="Sub1 3" class="Str"() -> ("Value"=w1306:string)  [unwired: 2 in, 2 out]
        n1351 = property on="Start" class="Bool (strict)"() -> ("Value"=w1539:bool)  [unwired: 2 in, 2 out]
        n1352 = property on="Ga2 5" class="Str"() -> ("Value"=w1530:string)  [unwired: 2 in, 2 out]
        n1353 = property on="nm 3" class="DigNum (strict)"() -> ("Value"=w1528:u32)  [unwired: 2 in, 2 out]
        n1354 = property on="A =" class="Str"() -> ("Value"=w1520:string)  [unwired: 2 in, 2 out]
        n1355 = property on="B =" class="Str"() -> ("Value"=w1519:string)  [unwired: 2 in, 2 out]
        n1356 = property on="C =" class="Str"() -> ("Value"=w1518:string)  [unwired: 2 in, 2 out]
        n1357 = property on="Sub1" class="Str"() -> ("Value"=w1513:string)  [unwired: 2 in, 2 out]
        n1358 = property on="Ga2 1" class="Str"() -> ("Value"=w1512:string)  [unwired: 2 in, 2 out]
        n1359 = property on="nm" class="DigNum (strict)"() -> ("Value"=w1510:u32)  [unwired: 2 in, 2 out]
        n1360 = property on="Ga2 6" class="Str"() -> ("Value"=w1304:string)  [unwired: 2 in, 2 out]
        n1361 = Format Into String "Growth Temperature Calibration"(format string="%s\\t%s\\t%s\\t%g\\t%s\\t%s\\t%s\\t%g\\t%s\\t%s\\t%s\\t%g\\t%s\\t%g\\t%s\\t%s\\t%s\\t%g\\t%s\\t%s\\t%s\\t%s\\t%s\\t%g\\t%s\\t%d\\t%s\\t%g\\t%s\\t%g\\t%s\\t%s\\t%s\\t%s\\t%s\\t%s\\t%s\\t%s\\t%s\\t%s\\t%s\\t%s\\t%s\\t%s\\t%s\\t%s\\t%s\\t%s\\t%s\\t%s\\t%s\\t%s\\t%s\\t%s\\t%s\\t%s\\t%s\\t%s\\t%s\\t%s\\t%s\\t%g\\t%s\\t%s\\t%s\\t%s\\t" ("格式字符串"), initial string=w1435, "Tab Control", w1540, "Start", w1539, "Reconstruction模型输出结果", w1538, "Obtaining the deoxidation temperature", w1537, "Substrate to find Deoxidation temperature ", w1536, "Whether to continue heating up operation", w1535, "Is the probability of the model output deoxidization exceeding", w1534, "Deoxidation temperature", w1533, "Outgassing at about 620 ℃ for 10 minutes", w1532, "Sub1 2", w1531, "Ga2 5", w1530, "GaAs buffer 0.6 μm/h", w1529, "nm 3", w1528, "Cool to less than 100 ℃ and wait 10 minutes", w1527, "Obtaining the reconstruction  temperature", w1526, "Substrate to find Reconstruction temperature", w1525, "From As cap to c(4×4)", w1524, "From c(4×4) to (2×4) ", w1523, "From (2×4) to (n×6)", w1522, "Obtain Growth Temperature", w1521, "A =", w1520, "B =", w1519, "C =", w1518, "MSE loss", w1517, "InAs growth temperature", w1516, "GaAs growth temperature", w1515, "Ready for GaAs buffer 0.6 μm/h", w1514, "Sub1", w1513, "Ga2 1", w1512, "GaAs buffer 0.6 μm/h ", w1511, "nm", w1510, "Sub1 3", w1306, "Ga2 6", w1304) -> (resulting string=w1434:string)  [unwired: 1 in, 1 out]
        n1362 = property on="10 nm GaAs cap layer 0.36 μm/h" class="Bool (strict)"() -> ("Value"=w1500:bool)  [unwired: 2 in, 2 out]
        n1363 = property on="Optimize Sub Temperature 1" class="Str"() -> ("Value"=w1502:string)  [unwired: 2 in, 2 out]
        n1364 = property on="Optimize Sub Temperature 2" class="Str"() -> ("Value"=w1488:string)  [unwired: 2 in, 2 out]
        n1365 = property on="If In Shutter can be closed 1" class="Bool (strict)"() -> ("Value"=w1501:bool)  [unwired: 2 in, 2 out]
        n1366 = property on="If In Shutter can be closed 2" class="Bool (strict)"() -> ("Value"=w1487:bool)  [unwired: 2 in, 2 out]
        n1367 = property on="模型输出是否超过0.7概率是Ys" class="Bool (strict)"() -> ("Value"=w1508:bool)  [unwired: 2 in, 2 out]
        n1368 = property on="Temperature模型输出结果 2" class="Str"() -> ("Value"=w1506:string)  [unwired: 2 in, 2 out]
        n1369 = property on="Temperature adjustment 1" class="Bool (strict)"() -> ("Value"=w1505:bool)  [unwired: 2 in, 2 out]
        n1370 = property on="Temperature adjustment 2" class="Bool (strict)"() -> ("Value"=w1499:bool)  [unwired: 2 in, 2 out]
        n1371 = property on="Temperature adjustment 3" class="Bool (strict)"() -> ("Value"=w1492:bool)  [unwired: 2 in, 2 out]
        n1372 = property on="Surface InAs QDs for AFM" class="Bool (strict)"() -> ("Value"=w1489:bool)  [unwired: 2 in, 2 out]
        n1373 = property on="GaAs buffer 0.6 μm/h  2" class="Bool (strict)"() -> ("Value"=w1496:bool)  [unwired: 2 in, 2 out]
        n1374 = property on="Shutter模型输出结果" class="Str"() -> ("Value"=w1507:string)  [unwired: 2 in, 2 out]
        n1375 = property on="Surface InAs QDs" class="Bool (strict)"() -> ("Value"=w1493:bool)  [unwired: 2 in, 2 out]
        n1376 = property on="Inside InAs QDs" class="Bool (strict)"() -> ("Value"=w1494:bool)  [unwired: 2 in, 2 out]
        n1377 = property on="Cooling" class="Bool (strict)"() -> ("Value"=w1486:bool)  [unwired: 2 in, 2 out]
        n1378 = property on="Sub2" class="Str"() -> ("Value"=w1504:string)  [unwired: 2 in, 2 out]
        n1379 = property on="Ga2 2" class="Str"() -> ("Value"=w1503:string)  [unwired: 2 in, 2 out]
        n1380 = property on="Sub3" class="Str"() -> ("Value"=w1498:string)  [unwired: 2 in, 2 out]
        n1381 = property on="Ga2 3" class="Str"() -> ("Value"=w1497:string)  [unwired: 2 in, 2 out]
        n1382 = property on="nm 2" class="DigNum (strict)"() -> ("Value"=w1495:u32)  [unwired: 2 in, 2 out]
        n1383 = property on="Sub4" class="Str"() -> ("Value"=w1491:string)  [unwired: 2 in, 2 out]
        n1384 = property on="Ga2 4" class="Str"() -> ("Value"=w1490:string)  [unwired: 2 in, 2 out]
        n1385 = property on="Sub5" class="Str"() -> ("Value"=w1485:string)  [unwired: 2 in, 2 out]
        n1386 = property on="Reconstruction probability" class="DigNum (strict)"() -> ("Value"=w1480:dbl)  [unwired: 2 in, 2 out]
        n1387 = property on="转换给模型的像素长宽大小" class="DigNum (strict)"() -> ("Value"=w1477:i32)  [unwired: 2 in, 2 out]
        n1388 = property on="选择多少张图片（通道）" class="DigNum (strict)"() -> ("Value"=w1476:i32)  [unwired: 2 in, 2 out]
        n1389 = property on="dimension size" class="DigNum (strict)"() -> ("Value"=w1479:i32)  [unwired: 2 in, 2 out]
        n1390 = property on="Suitable prop" class="DigNum (strict)"() -> ("Value"=w1481:dbl)  [unwired: 2 in, 2 out]
        n1391 = property on="Yes prop" class="DigNum (strict)"() -> ("ClassName"=w1483:string)  [unwired: 2 in, 2 out]
        n1392 = Format Into String(format string="%s\\t%g\\t%s\\t%s\\t%s\\t%s\\t%s\\t%g\\t%s\\t%s\\t%s\\t%s\\t%s\\t%g\\t%s\\t%s\\t%s\\t%g\\t%s\\t%g\\t%s\\t%g\\t%s\\t%s\\t%s\\t%s\\t%s\\t%g\\t%s\\t%d\\t%s\\t%g\\t%s\\t%g\\t%s\\t%s\\t%s\\t%s\\t%s\\t%g\\t%s\\t%s\\t%s\\t%g\\t%s\\t%g\\t%s\\t%s\\t" ("格式字符串"), initial string=w1434, "模型输出是否超过0.7概率是Ys", w1508, "Shutter模型输出结果", w1507, "Temperature模型输出结果 2", w1506, "Temperature adjustment 1", w1505, "Sub2 2", w1504, "Ga2 2", w1503, "Inside InAs QDs", w1494, "Optimize Sub Temperature 1", w1502, "If In Shutter can be closed 1", w1501, "10 nm GaAs cap layer 0.36 μm/h ", w1500, "Temperature adjustment 2", w1499, "Sub3", w1498, "Ga2 3", w1497, "GaAs buffer 0.6 μm/h  2", w1496, "nm 2", w1495, "Surface InAs QDs", w1493, "Temperature adjustment 3", w1492, "Sub4", w1491, "Ga2 4", w1490, "Surface InAs QDs for AFM", w1489, "Optimize Sub Temperature 2", w1488, "If In Shutter can be closed 2", w1487, "Cooling", w1486, "Sub5", w1485) -> (resulting string=w1433:string)  [unwired: 1 in, 1 out]
        n1393 = property on="10 nm LT-GaAs switch Yes is do" class="Bool (strict)"() -> ("Value"=w1475:bool)  [unwired: 2 in, 2 out]
        n1394 = property on="Yes prop" class="DigNum (strict)"() -> ("Value"=w1482:dbl)  [unwired: 2 in, 2 out]
        n1395 = property on="repetition 1 LT-GaAs not do" class="Bool (strict)"() -> ("Value"=w1474:bool)  [unwired: 2 in, 2 out]
        n1396 = property on="If In Shutter can be closed 1" class="Bool (strict)"() -> ("Value"=w1303:bool)  [unwired: 2 in, 2 out]
        n1397 = property on="T" class="DigNum (strict)"() -> ("Value"=w1478:i32)  [unwired: 2 in, 2 out]
        n1398 = property on="Model switch" class="Bool (strict)"() -> ("Value"=w1301:bool)  [unwired: 2 in, 2 out]
        n1399 = property on="倒计时开关" class="Bool (strict)"() -> ("Value"=w1473:bool)  [unwired: 2 in, 2 out]
        n1400 = property on="Is the probability of the model output oxidization exceeding" class="Bool (strict)"() -> ("Value"=w1455:bool)  [unwired: 2 in, 2 out]
        n1401 = Format Into String(format string="%s\\t%g\\t%s\\t%g\\t%s\\t%g\\t%s\\t%d\\t%s\\t%d\\t%s\\t%d\\t%s\\t%d\\t" ("格式字符串"), initial string=w1433, w1483, w1482, "Suitable prop", w1481, "Reconstruction probability", w1480, "dimension size", w1479, "T", w1478, "转换给模型的像素长宽大小", w1477, "选择多少张图片（通道）", w1476) -> (resulting string=w1432:string)  [unwired: 1 in, 1 out]
        n1402 = property on="Is the probability of the model output As cap exceeding" class="Bool (strict)"() -> ("Value"=w1458:bool)  [unwired: 2 in, 2 out]
        n1403 = property on="Is the probability of the model output c(4×4) exceeding" class="Bool (strict)"() -> ("Value"=w1457:bool)  [unwired: 2 in, 2 out]
        n1404 = property on="Is the probability of the model output (2×4) exceeding" class="Bool (strict)"() -> ("Value"=w1456:bool)  [unwired: 2 in, 2 out]
        n1405 = property on="Is the probability of the model output (n×6) exceeding" class="Bool (strict)"() -> ("Value"=w1454:bool)  [unwired: 2 in, 2 out]
        n1406 = property on="In挡板" class="Bool (strict)"() -> ("Value"=w1302:bool)  [unwired: 2 in, 2 out]
        n1407 = property on="4 Deoxidization number" class="DigNum (strict)"() -> ("Value"=w1460:u8)  [unwired: 2 in, 2 out]
        n1408 = property on="Whether to continue heat up for reconstruction" class="Bool (strict)"() -> ("Value"=w1452:bool)  [unwired: 2 in, 2 out]
        n1409 = property on="4 Deoxidization count" class="DigNum (strict)"() -> ("Value"=w1466:u8)  [unwired: 2 in, 2 out]
        n1410 = property on="3 Oxidization number" class="DigNum (strict)"() -> ("Value"=w1461:u8)  [unwired: 2 in, 2 out]
        n1411 = property on="repeats of InAs/GaAs" class="DigNum (strict)"() -> ("Value"=w1472:i32)  [unwired: 2 in, 2 out]
        n1412 = property on="3 Oxidization count" class="DigNum (strict)"() -> ("Value"=w1467:u8)  [unwired: 2 in, 2 out]
        n1413 = property on="0 As cap number" class="DigNum (strict)"() -> ("Value"=w1464:u8)  [unwired: 2 in, 2 out]
        n1414 = property on="1 c(4×4) number" class="DigNum (strict)"() -> ("Value"=w1463:i32)  [unwired: 2 in, 2 out]
        n1415 = property on="2 (2×4) number" class="DigNum (strict)"() -> ("Value"=w1462:u8)  [unwired: 2 in, 2 out]
        n1416 = property on="5 (n×6) number" class="DigNum (strict)"() -> ("Value"=w1459:i32)  [unwired: 2 in, 2 out]
        n1417 = property on="0 As cap count" class="DigNum (strict)"() -> ("Value"=w1470:u8)  [unwired: 2 in, 2 out]
        n1418 = property on="While loop for cool to less than 100 ℃" class="Bool (strict)"() -> ("Value"=w1453:bool)  [unwired: 2 in, 2 out]
        n1419 = property on="1 c(4×4) count" class="DigNum (strict)"() -> ("Value"=w1469:i32)  [unwired: 2 in, 2 out]
        n1420 = property on="2 (2×4) count" class="DigNum (strict)"() -> ("Value"=w1468:u8)  [unwired: 2 in, 2 out]
        n1421 = property on="5 (n×6) count" class="DigNum (strict)"() -> ("Value"=w1465:i32)  [unwired: 2 in, 2 out]
        n1422 = property on="Repetition" class="DigNum (strict)"() -> ("Value"=w1471:i32)  [unwired: 2 in, 2 out]
        n1423 = Format Into String(format string="%s\\t%g\\t%s\\t%g\\t%s\\t%g\\t%s\\t%g\\t%s\\t%g\\t%s\\t%g\\t" ("格式字符串"), initial string=w1432, "In挡板", w1302, "10 nm LT-GaAs switch Yes is do ", w1475, "If In Shutter can be closed 1", w1303, "repetition 1 LT-GaAs not do", w1474, "Model switch", w1301, "倒计时开关", w1473) -> (resulting string=w1431:string)  [unwired: 1 in, 1 out]
        n1424 = Format Into String(format string="%s\\t%d\\t%s\\t%d\\t%s\\t%d\\t%s\\t%d\\t%s\\t%d\\t%s\\t%d\\t%s\\t%d\\t%s\\t%d\\t%s\\t%d\\t%s\\t%d\\t%s\\t%d\\t%s\\t%d\\t%s\\t%d\\t%s\\t%d\\t" ("格式字符串"), initial string=w1431, "repeats of InAs/GaAs", w1472, "Repetition", w1471, "0 As cap count", w1470, "1 c(4×4) count", w1469, "2 (2×4) count", w1468, "3 Oxidization count", w1467, "4 Deoxidization count", w1466, "5 (n×6) count", w1465, "0 As cap number", w1464, "1 c(4×4) number", w1463, "2 (2×4) number", w1462, "3 Oxidization number", w1461, "4 Deoxidization number", w1460, "5 (n×6) number", w1459) -> (resulting string=w1430:string)  [unwired: 1 in, 1 out]
        n1425 = property on="Temperature count Suitable" class="DigNum (strict)"() -> ("Value"=w1448:u8)  [unwired: 2 in, 2 out]
        n1426 = property on="Temperature count result" class="DigNum (strict)"() -> ("Value"=w1447:u8)  [unwired: 2 in, 2 out]
        n1427 = property on="Temperature count High" class="DigNum (strict)"() -> ("Value"=w1450:u8)  [unwired: 2 in, 2 out]
        n1428 = property on="Temperature count Low" class="DigNum (strict)"() -> ("Value"=w1449:u8)  [unwired: 2 in, 2 out]
        n1429 = property on="Shutter count Yes result" class="DigNum (strict)"() -> ("Value"=w1443:u8)  [unwired: 2 in, 2 out]
        n1430 = property on="Temperature Switch" class="DigNum (strict)"() -> ("Value"=w1446:i32)  [unwired: 2 in, 2 out]
        n1431 = property on="Shutter count Yes" class="DigNum (strict)"() -> ("Value"=w1444:u8)  [unwired: 2 in, 2 out]
        n1432 = property on="Shutter count No" class="DigNum (strict)"() -> ("Value"=w1445:u8)  [unwired: 2 in, 2 out]
        n1433 = property on="Growth Switch" class="DigNum (strict)"() -> ("Value"=w1451:i32)  [unwired: 2 in, 2 out]
        n1434 = Format Into String(format string="%s\\t%g\\t%s\\t%g\\t%s\\t%g\\t%s\\t%g\\t%s\\t%g\\t%s\\t%g\\t%s\\t%g\\t" ("格式字符串"), initial string=w1430, "Is the probability of the model output As cap exceeding", w1458, "Is the probability of the model output c(4×4) exceeding", w1457, "Is the probability of the model output (2×4) exceeding", w1456, "Is the probability of the model output oxidization exceeding", w1455, "Is the probability of the model output (n×6) exceeding", w1454, "While loop for cool to less than 100 ℃", w1453, "Whether to continue heat up for reconstruction", w1452) -> (resulting string=w1429:string)  [unwired: 1 in, 1 out]
        n1435 = Format Into String(format string="%s\\t%d\\t%s\\t%d\\t%s\\t%d\\t%s\\t%d\\t%s\\t%d\\t%s\\t%d\\t%s\\t%d\\t%s\\t%d\\t%s\\t%d\\t" ("格式字符串"), initial string=w1429, "Growth Switch", w1451, "Temperature count High", w1450, "Temperature count Low", w1449, "Temperature count Suitable", w1448, "Temperature count result", w1447, "Temperature Switch", w1446, "Shutter count No", w1445, "Shutter count Yes", w1444, "Shutter count Yes result", w1443) -> (resulting string=w1437:string)  [unwired: 1 in, 1 out]
        n1436 = Build Array(w1437) -> (w1428:string[])
        n1437 = call-poly <vilib>:"Write Delimited Spreadsheet.vi"("file path (dialog if empty)"=w1562, "1D data"=w1428, "append to file? (new file:F)"=TRUE) -> ()  [unwired: 11 in, 2 out]
      }
    }
  }
  n1438 = call-poly <vilib>:"Set Cursor.vi"() -> ()  [unwired: 10 in, 2 out]
  n1439 = property on="转换给模型的像素长宽大小" class="DigNum (strict)"() -> ("Value"=w57:i32)  [unwired: 2 in, 2 out]
  n1440 = property on="转换给模型的像素长宽大小" class="DigNum (strict)"() -> ("Value"=w58:i32)  [unwired: 2 in, 2 out]
  n1441 = while {
    stop <- FALSE stop-if-true
    n1442 = flat-sequence {
      frame #0 {
        w1576 = u8 0 ("Value (Signaling)")
        n1443 = property on="Temperature count Low" class="DigNum (strict)"("Val(Sgnl)"=w1576) -> ()  [unwired: 2 in, 2 out]
        n1444 = property on="Temperature count Suitable" class="DigNum (strict)"("Val(Sgnl)"=w1576) -> ()  [unwired: 2 in, 2 out]
        n1445 = property on="Temperature count High" class="DigNum (strict)"("Val(Sgnl)"=w1576) -> ()  [unwired: 2 in, 2 out]
      }
      frame #1 {
        n1446 = property on="记录Temperature模型的连续24个输出结果" class="Arr (strict)"() -> ("Value"=w1578:u8[])  [unwired: 2 in, 2 out]
        n1447 = property on="dimension size" class="DigNum (strict)"() -> ("Value"=w1577:i32)  [unwired: 2 in, 2 out]
        n1448 = for {
          N: w1577 -> [_]
          tunnel: w1578 -> [w1581]
          i -> [w1580]
          n1449 = Index Array(array=w1581, index=w1580) -> (element=w1579:u8)
          n1450 = Equal?(x=w1579, y=0 ("index")) -> (x = y?=w1587:bool)
          n1451 = Equal?(x=w1579, y=1 ("index")) -> (x = y?=w1586:bool)
          n1452 = Equal?(x=w1579, y=2 ("index")) -> (x = y?=w1585:bool)
          n1453 = case shown="True" w1587 {
            frame False {
            }
            frame True {
              n1454 = property on="Temperature count High" class="DigNum (strict)"() -> ("Value"=w1593:u8)  [unwired: 2 in, 2 out]
              n1455 = Increment(x=w1593) -> (x+1=w1592:u8)
              n1456 = property on="Temperature count High" class="DigNum (strict)"("Val(Sgnl)"=w1592) -> ()  [unwired: 2 in, 2 out]
            }
          }
          n1457 = case shown="True" w1586 {
            frame False {
            }
            frame True {
              n1458 = property on="Temperature count Low" class="DigNum (strict)"() -> ("Value"=w1591:u8)  [unwired: 2 in, 2 out]
              n1459 = Increment(x=w1591) -> (x+1=w1590:u8)
              n1460 = property on="Temperature count Low" class="DigNum (strict)"("Val(Sgnl)"=w1590) -> ()  [unwired: 2 in, 2 out]
            }
          }
          n1461 = case shown="True" w1585 {
            frame False {
            }
            frame True {
              n1462 = property on="Temperature count Suitable" class="DigNum (strict)"() -> ("Value"=w1589:u8)  [unwired: 2 in, 2 out]
              n1463 = Increment(x=w1589) -> (x+1=w1588:u8)
              n1464 = property on="Temperature count Suitable" class="DigNum (strict)"("Val(Sgnl)"=w1588) -> ()  [unwired: 2 in, 2 out]
            }
          }
        }
      }
      frame #2 {
        n1465 = property on="Temperature count Suitable" class="DigNum (strict)"() -> ("Value"=w1606:u8)  [unwired: 2 in, 2 out]
        n1466 = property on="Temperature count High" class="DigNum (strict)"() -> ("Value"=w1608:u8)  [unwired: 2 in, 2 out]
        n1467 = property on="Temperature count Low" class="DigNum (strict)"() -> ("Value"=w1607:u8)  [unwired: 2 in, 2 out]
        n1468 = Build Array(w1608, w1607, w1606) -> (w1598:u8[])
        n1469 = property on="dimension size" class="DigNum (strict)"() -> ("Value"=w1601:i32)  [unwired: 2 in, 2 out]
        n1470 = Index Array(array=w1598, index=0) -> (element=w1597:u8)
        n1471 = Index Array(array=w1598, index=1) -> (element=w1596:u8)
        n1472 = Index Array(array=w1598, index=2) -> (element=w1604:u8)
        n1473 = property on="Suitable prop" class="DigNum (strict)"() -> ("Value"=w1594:dbl)  [unwired: 2 in, 2 out]
        n1474 = Greater?(x=w1597, y=w1596) -> (0:w1595:bool)
        n1475 = Divide(x=w1604, y=w1601) -> (x/y=w1603:dbl)
        n1476 = Greater?(x=w1603, y=w1594) -> (0:w1602:bool)
        n1477 = case shown="True" w1602 {
          tunnel: w1595 -> [w1609 _]
          frame False {
            n1478 = case shown="True" w1609 {
              frame False {
                n1479 = property on="Temperature count result" class="DigNum (strict)"("Val(Sgnl)"=u8 1 ("Value (Signaling)")) -> ()  [unwired: 2 in, 2 out]
                n1480 = Wait (ms)(milliseconds to wait=u32 2000) -> ()  [unwired: 1 out]
              }
              frame True {
                n1481 = property on="Temperature count result" class="DigNum (strict)"("Val(Sgnl)"=u8 0 ("Value (Signaling)")) -> ()  [unwired: 2 in, 2 out]
                n1482 = Wait (ms)(milliseconds to wait=u32 2000) -> ()  [unwired: 1 out]
              }
            }
          }
          frame True {
            n1483 = property on="Temperature count result" class="DigNum (strict)"("Val(Sgnl)"=u8 2 ("Value (Signaling)")) -> ()  [unwired: 2 in, 2 out]
          }
        }
      }
    }
  }
  n1484 = while {
    stop <- FALSE stop-if-true
    n1485 = flat-sequence {
      tunnel: [w1619] -> w1616
      tunnel: w1616 -> [w1633]
      tunnel: [w1633] -> w1615
      tunnel: w1615 -> [w1637]
      frame #0 {
        w1618 = u8 0 ("Value (Signaling)")
        n1486 = property on="Shutter count No" class="DigNum (strict)"("Val(Sgnl)"=w1618) -> ()  [unwired: 2 in, 2 out]
        n1487 = property on="Shutter count Yes" class="DigNum (strict)"("Val(Sgnl)"=w1618) -> ()  [unwired: 2 in, 2 out]
      }
      frame #1 {
        n1488 = property on="记录Shutter模型的连续24个输出结果" class="Arr (strict)"() -> ("Value"=w1620:u8[])  [unwired: 2 in, 2 out]
        n1489 = property on="dimension size" class="DigNum (strict)"() -> ("Value"=w1619:i32)  [unwired: 2 in, 2 out]
        n1490 = for {
          N: w1619 -> [_]
          tunnel: w1620 -> [w1621]
          i -> [w1627]
          n1491 = Index Array(array=w1621, index=w1627) -> (element=w1622:u8)
          n1492 = Equal?(x=w1622, y=0 ("index")) -> (x = y?=w1624:bool)
          n1493 = Equal?(x=w1622, y=1 ("index")) -> (x = y?=w1623:bool)
          n1494 = case shown="True" w1624 {
            frame False {
            }
            frame True {
              n1495 = property on="Shutter count No" class="DigNum (strict)"() -> ("Value"=w1631:u8)  [unwired: 2 in, 2 out]
              n1496 = Increment(x=w1631) -> (x+1=w1630:u8)
              n1497 = property on="Shutter count No" class="DigNum (strict)"("Val(Sgnl)"=w1630) -> ()  [unwired: 2 in, 2 out]
            }
          }
          n1498 = case shown="True" w1623 {
            frame False {
            }
            frame True {
              n1499 = property on="Shutter count Yes" class="DigNum (strict)"() -> ("Value"=w1629:u8)  [unwired: 2 in, 2 out]
              n1500 = Increment(x=w1629) -> (x+1=w1628:u8)
              n1501 = property on="Shutter count Yes" class="DigNum (strict)"("Val(Sgnl)"=w1628) -> ()  [unwired: 2 in, 2 out]
            }
          }
        }
      }
      frame #2 {
        n1502 = property on="Shutter count Yes" class="DigNum (strict)"() -> ("Value"=w1632:u8)  [unwired: 2 in, 2 out]
        n1503 = property on="Shutter count Yes result" class="DigNum (strict)"("Val(Sgnl)"=w1632) -> ()  [unwired: 2 in, 2 out]
      }
      frame #3 {
        n1504 = property on="Shutter count Yes result" class="DigNum (strict)"() -> ("Value"=w1636:u8)  [unwired: 2 in, 2 out]
        n1505 = Divide(x=w1636, y=w1637) -> (x/y=w1638:dbl)
        n1506 = property on="Yes prop" class="DigNum (strict)"() -> ("Value"=w1634:dbl)  [unwired: 2 in, 2 out]
        n1507 = Greater Or Equal?(x=w1638, y=w1634) -> (x >= y?=w1639:bool)
        n1508 = property on="In挡板" class="Bool (strict)"() -> ("Value"=w1635:bool)  [unwired: 2 in, 2 out]
        n1509 = case shown="False" w1635 {
          tunnel: w1639 -> [_ w1641]
          frame False {
            n1510 = property on="模型输出是否超过0.7概率是Ys" class="Bool (strict)"("Val(Sgnl)"=FALSE ("Value (Signaling)")) -> ()  [unwired: 2 in, 2 out]
          }
          frame True {
            n1511 = case shown="False" w1641 {
              frame False {
                n1512 = property on="模型输出是否超过0.7概率是Ys" class="Bool (strict)"("Val(Sgnl)"=FALSE ("Value (Signaling)")) -> ()  [unwired: 2 in, 2 out]
              }
              frame True {
                n1513 = property on="模型输出是否超过0.7概率是Ys" class="Bool (strict)"("Val(Sgnl)"=TRUE ("Value (Signaling)")) -> ()  [unwired: 2 in, 2 out]
              }
            }
          }
        }
      }
    }
  }
  n1514 = while {
    stop <- FALSE stop-if-true
    n1515 = flat-sequence {
      tunnel: [w1649] -> w1645
      tunnel: w1645 -> [w1683]
      tunnel: [w1683] -> w1644
      tunnel: w1644 -> [w1694]
      frame #0 {
        w1647 = u8 0 ("Value (Signaling)")
        n1516 = property on="3 Oxidization number" class="DigNum (strict)"("Val(Sgnl)"=w1647) -> ()  [unwired: 2 in, 2 out]
        n1517 = property on="4 Deoxidization number" class="DigNum (strict)"("Val(Sgnl)"=w1647) -> ()  [unwired: 2 in, 2 out]
        n1518 = property on="5 (n×6) number" class="DigNum (strict)"("Val(Sgnl)"=w1647) -> ()  [unwired: 2 in, 2 out]
        n1519 = property on="0 As cap number" class="DigNum (strict)"("Val(Sgnl)"=w1647) -> ()  [unwired: 2 in, 2 out]
        n1520 = property on="1 c(4×4) number" class="DigNum (strict)"("Val(Sgnl)"=w1647) -> ()  [unwired: 2 in, 2 out]
        n1521 = property on="2 (2×4) number" class="DigNum (strict)"("Val(Sgnl)"=w1647) -> ()  [unwired: 2 in, 2 out]
      }
      frame #1 {
        n1522 = property on="记录Reconstruction模型的连续24个输出结果" class="Arr (strict)"() -> ("Value"=w1648:u8[])  [unwired: 2 in, 2 out]
        n1523 = property on="dimension size" class="DigNum (strict)"() -> ("Value"=w1649:i32)  [unwired: 2 in, 2 out]
        n1524 = for {
          N: w1649 -> [_]
          tunnel: w1648 -> [w1659]
          i -> [w1664]
          n1525 = Index Array(array=w1659, index=w1664) -> (element=w1650:u8)
          n1526 = Equal?(x=w1650, y=0 ("index")) -> (x = y?=w1661:bool)
          n1527 = Equal?(x=w1650, y=1 ("index")) -> (x = y?=w1660:bool)
          n1528 = Equal?(x=w1650, y=2 ("index")) -> (x = y?=w1658:bool)
          n1529 = Equal?(x=w1650, y=3 ("index")) -> (x = y?=w1655:bool)
          n1530 = Equal?(x=w1650, y=5 ("index")) -> (x = y?=w1652:bool)
          n1531 = Equal?(x=w1650, y=4 ("index")) -> (x = y?=w1653:bool)
          n1532 = case shown="False" w1661 {
            frame False {
            }
            frame True {
              n1533 = property on="0 As cap number" class="DigNum (strict)"() -> ("Value"=w1675:u8)  [unwired: 2 in, 2 out]
              n1534 = Increment(x=w1675) -> (x+1=w1676:u8)
              n1535 = property on="0 As cap number" class="DigNum (strict)"("Val(Sgnl)"=w1676) -> ()  [unwired: 2 in, 2 out]
            }
          }
          n1536 = case shown="True" w1660 {
            frame False {
            }
            frame True {
              n1537 = property on="1 c(4×4) number" class="DigNum (strict)"() -> ("Value"=w1673:i32)  [unwired: 2 in, 2 out]
              n1538 = Increment(x=w1673) -> (x+1=w1674:i32)
              n1539 = property on="1 c(4×4) number" class="DigNum (strict)"("Val(Sgnl)"=w1674) -> ()  [unwired: 2 in, 2 out]
            }
          }
          n1540 = case shown="True" w1658 {
            frame False {
            }
            frame True {
              n1541 = property on="2 (2×4) number" class="DigNum (strict)"() -> ("Value"=w1671:u8)  [unwired: 2 in, 2 out]
              n1542 = Increment(x=w1671) -> (x+1=w1672:u8)
              n1543 = property on="2 (2×4) number" class="DigNum (strict)"("Val(Sgnl)"=w1672) -> ()  [unwired: 2 in, 2 out]
            }
          }
          n1544 = case shown="True" w1655 {
            frame False {
            }
            frame True {
              n1545 = property on="3 Oxidization number" class="DigNum (strict)"() -> ("Value"=w1669:u8)  [unwired: 2 in, 2 out]
              n1546 = Increment(x=w1669) -> (x+1=w1670:u8)
              n1547 = property on="3 Oxidization number" class="DigNum (strict)"("Val(Sgnl)"=w1670) -> ()  [unwired: 2 in, 2 out]
            }
          }
          n1548 = case shown="True" w1652 {
            frame False {
            }
            frame True {
              n1549 = property on="5 (n×6) number" class="DigNum (strict)"() -> ("Value"=w1665:i32)  [unwired: 2 in, 2 out]
              n1550 = Increment(x=w1665) -> (x+1=w1666:i32)
              n1551 = property on="5 (n×6) number" class="DigNum (strict)"("Val(Sgnl)"=w1666) -> ()  [unwired: 2 in, 2 out]
            }
          }
          n1552 = case shown="True" w1653 {
            frame False {
            }
            frame True {
              n1553 = property on="4 Deoxidization number" class="DigNum (strict)"() -> ("Value"=w1667:u8)  [unwired: 2 in, 2 out]
              n1554 = Increment(x=w1667) -> (x+1=w1668:u8)
              n1555 = property on="4 Deoxidization number" class="DigNum (strict)"("Val(Sgnl)"=w1668) -> ()  [unwired: 2 in, 2 out]
            }
          }
        }
      }
      frame #2 {
        n1556 = property on="3 Oxidization number" class="DigNum (strict)"() -> ("Value"=w1677:u8)  [unwired: 2 in, 2 out]
        n1557 = property on="4 Deoxidization number" class="DigNum (strict)"() -> ("Value"=w1680:u8)  [unwired: 2 in, 2 out]
        n1558 = property on="0 As cap number" class="DigNum (strict)"() -> ("Value"=w1678:u8)  [unwired: 2 in, 2 out]
        n1559 = property on="1 c(4×4) number" class="DigNum (strict)"() -> ("Value"=w1682:i32)  [unwired: 2 in, 2 out]
        n1560 = property on="2 (2×4) number" class="DigNum (strict)"() -> ("Value"=w1681:u8)  [unwired: 2 in, 2 out]
        n1561 = property on="5 (n×6) number" class="DigNum (strict)"() -> ("Value"=w1679:i32)  [unwired: 2 in, 2 out]
        n1562 = property on="3 Oxidization count" class="DigNum (strict)"("Val(Sgnl)"=w1677) -> ()  [unwired: 2 in, 2 out]
        n1563 = property on="2 (2×4) count" class="DigNum (strict)"("Val(Sgnl)"=w1681) -> ()  [unwired: 2 in, 2 out]
        n1564 = property on="5 (n×6) count" class="DigNum (strict)"("Val(Sgnl)"=w1679) -> ()  [unwired: 2 in, 2 out]
        n1565 = property on="0 As cap count" class="DigNum (strict)"("Val(Sgnl)"=w1678) -> ()  [unwired: 2 in, 2 out]
        n1566 = property on="1 c(4×4) count" class="DigNum (strict)"("Val(Sgnl)"=w1682) -> ()  [unwired: 2 in, 2 out]
        n1567 = property on="4 Deoxidization count" class="DigNum (strict)"("Val(Sgnl)"=w1680) -> ()  [unwired: 2 in, 2 out]
      }
      frame #3 {
        n1568 = property on="0 As cap count" class="DigNum (strict)"() -> ("Value"=w1704:u8)  [unwired: 2 in, 2 out]
        n1569 = property on="1 c(4×4) count" class="DigNum (strict)"() -> ("Value"=w1700:i32)  [unwired: 2 in, 2 out]
        n1570 = property on="2 (2×4) count" class="DigNum (strict)"() -> ("Value"=w1699:u8)  [unwired: 2 in, 2 out]
        n1571 = property on="5 (n×6) count" class="DigNum (strict)"() -> ("Value"=w1695:i32)  [unwired: 2 in, 2 out]
        n1572 = property on="4 Deoxidization count" class="DigNum (strict)"() -> ("Value"=w1697:u8)  [unwired: 2 in, 2 out]
        n1573 = property on="3 Oxidization count" class="DigNum (strict)"() -> ("Value"=w1698:u8)  [unwired: 2 in, 2 out]
        n1574 = property on="Reconstruction probability" class="DigNum (strict)"() -> ("Value"=w1685:dbl)  [unwired: 2 in, 2 out]
        n1575 = property on="Obtaining the reconstruction  temperature" class="Bool (strict)"() -> ("Value"=w1693:bool)  [unwired: 2 in, 2 out]
        n1576 = Divide(x=w1704, y=w1694) -> (x/y=w1686:dbl)
        n1577 = Divide(x=w1700, y=w1694) -> (x/y=w1703:dbl)
        n1578 = Divide(x=w1699, y=w1694) -> (x/y=w1702:dbl)
        n1579 = Divide(x=w1695, y=w1694) -> (x/y=w1696:dbl)
        n1580 = Divide(x=w1698, y=w1694) -> (x/y=w1687:dbl)
        n1581 = Divide(x=w1697, y=w1694) -> (x/y=w1701:dbl)
        n1582 = Greater Or Equal?(x=w1687, y=w1685) -> (x >= y?=w1684:bool)
        n1583 = Greater Or Equal?(x=w1686, y=w1685) -> (x >= y?=w1691:bool)
        n1584 = Greater Or Equal?(x=w1701, y=w1685) -> (x >= y?=w1692:bool)
        n1585 = Greater Or Equal?(x=w1703, y=w1685) -> (x >= y?=w1690:bool)
        n1586 = Greater Or Equal?(x=w1702, y=w1685) -> (x >= y?=w1689:bool)
        n1587 = Greater Or Equal?(x=w1696, y=w1685) -> (x >= y?=w1688:bool)
        n1588 = case shown="False" w1693 {
          tunnel: w1692 -> [w1706 _]
          tunnel: w1684 -> [w1705 _]
          tunnel: w1691 -> [_ w1714]
          tunnel: w1690 -> [_ w1713]
          tunnel: w1689 -> [_ w1712]
          tunnel: w1688 -> [_ w1711]
          frame False {
            n1589 = case shown="True" w1705 {
              frame False {
                n1590 = property on="Is the probability of the model output oxidization exceeding" class="Bool (strict)"("Val(Sgnl)"=FALSE ("Value (Signaling)")) -> ()  [unwired: 2 in, 2 out]
              }
              frame True {
                n1591 = property on="Is the probability of the model output oxidization exceeding" class="Bool (strict)"("Val(Sgnl)"=TRUE ("Value (Signaling)")) -> ()  [unwired: 2 in, 2 out]
              }
            }
            n1592 = case shown="True" w1706 {
              frame False {
                n1593 = property on="Is the probability of the model output deoxidization exceeding" class="Bool (strict)"("Val(Sgnl)"=FALSE ("Value (Signaling)")) -> ()  [unwired: 2 in, 2 out]
              }
              frame True {
                n1594 = property on="Is the probability of the model output deoxidization exceeding" class="Bool (strict)"("Val(Sgnl)"=TRUE ("Value (Signaling)")) -> ()  [unwired: 2 in, 2 out]
              }
            }
          }
          frame True {
            n1595 = case shown="False" w1714 {
              frame False {
                n1596 = property on="Is the probability of the model output As cap exceeding" class="Bool (strict)"("Val(Sgnl)"=FALSE ("Value (Signaling)")) -> ()  [unwired: 2 in, 2 out]
              }
              frame True {
                n1597 = property on="Is the probability of the model output As cap exceeding" class="Bool (strict)"("Val(Sgnl)"=TRUE ("Value (Signaling)")) -> ()  [unwired: 2 in, 2 out]
              }
            }
            n1598 = case shown="False" w1713 {
              frame False {
                n1599 = property on="Is the probability of the model output c(4×4) exceeding" class="Bool (strict)"("Val(Sgnl)"=FALSE ("Value (Signaling)")) -> ()  [unwired: 2 in, 2 out]
              }
              frame True {
                n1600 = property on="Is the probability of the model output c(4×4) exceeding" class="Bool (strict)"("Val(Sgnl)"=TRUE ("Value (Signaling)")) -> ()  [unwired: 2 in, 2 out]
              }
            }
            n1601 = case shown="False" w1712 {
              frame False {
                n1602 = property on="Is the probability of the model output (2×4) exceeding" class="Bool (strict)"("Val(Sgnl)"=FALSE ("Value (Signaling)")) -> ()  [unwired: 2 in, 2 out]
              }
              frame True {
                n1603 = property on="Is the probability of the model output (2×4) exceeding" class="Bool (strict)"("Val(Sgnl)"=TRUE ("Value (Signaling)")) -> ()  [unwired: 2 in, 2 out]
              }
            }
            n1604 = case shown="False" w1711 {
              frame False {
                n1605 = property on="Is the probability of the model output (n×6) exceeding" class="Bool (strict)"("Val(Sgnl)"=FALSE ("Value (Signaling)")) -> ()  [unwired: 2 in, 2 out]
              }
              frame True {
                n1606 = property on="Is the probability of the model output (n×6) exceeding" class="Bool (strict)"("Val(Sgnl)"=TRUE ("Value (Signaling)")) -> ()  [unwired: 2 in, 2 out]
              }
            }
          }
        }
      }
    }
  }
  n1607 = property on="选择多少张图片（通道）" class="DigNum (strict)"() -> ("Value"=w59:i32)  [unwired: 2 in, 2 out]
  n1608 = property on="摄像头选择" class="IMAQdx (strict)"("Val(Sgnl)"=T3 "cam0" ("值(信号)")) -> ()  [unwired: 2 in, 2 out]
  n1609 = Obtain Queue(max queue size (-1, unlimited)=1 ("队列最大值（-1，无限）"), name (unnamed)="date2" ("名称（未命名）"), element data type=0.0) -> (queue out=w67:refnum<queue>, error out=w66:errorcluster)  [unwired: 2 in, 1 out]
  n1610 = property on="摄像头选择" class="IMAQdx (strict)"("DisabledEnum"=T4."Enabled" ("禁用")) -> ()  [unwired: 2 in, 2 out]
  n1611 = while {
    tunnel: w67 -> [w1726]
    tunnel: w66 -> [w1724]
    stop <- FALSE stop-if-true
    # "摄像头部分"
    n1612 = event shown="[1] \"摄像头开关\": Value Change" {
      selector: _ -> [_ _]
      dyn-events: _ -> [_ _]
      timeout: 10 -> [_ _]
      tunnel: w1726 -> [_ w1730]
      tunnel: w1724 -> [_ w1729]
      tunnel: [_ w1728] -> w1723
      event Timeout {
        n1613 = event-data() -> ()  [unwired: 1 in, 2 out]
      }
      event "摄像头开关": Value Change {
        n1614 = event-data() -> ("NewVal"=w1731:bool)  [unwired: 1 in, 4 out]
        n1615 = case shown="True" w1731 {
          tunnel: w1730 -> [_ w1741]
          tunnel: w1729 -> [w1733 w1740]
          tunnel: [w1732 w1738] -> w1728
          frame False {
            n1616 = property on="摄像头选择" class="IMAQdx (strict)"(error in=w1733) -> (error out=w1734:errorcluster, "Value"=w1735:T3)  [unwired: 1 in, 1 out]
            n1617 = property on="摄像头选择" class="IMAQdx (strict)"("DisabledEnum"=T4."Enabled" ("禁用")) -> ()  [unwired: 2 in, 2 out]
            n1618 = call <vilib>:"IMAQdx Close Camera.vi"("error in"=w1734, "Session In"=w1735) -> ("error out"=w1732:errorcluster)  [unwired: 9 in]
          }
          frame True {
            w1739 = T5 0 items=["Grayscale (U8)", "Grayscale (I16)", "Grayscale (SGL)", "Complex (CSG)", "RGB (U32)", "HSL (U32)", "RGB (U64)", "Grayscale (U16)"] ("Image Type")
            w1744 = T5 4 items=["Grayscale (U8)", "Grayscale (I16)", "Grayscale (SGL)", "Complex (CSG)", "RGB (U32)", "HSL (U32)", "RGB (U64)", "Grayscale (U16)"] ("Image Type")
            n1619 = property on="摄像头选择" class="IMAQdx (strict)"() -> ("Value"=w1752:T3)  [unwired: 2 in, 2 out]
            n1620 = call <vilib>:"IMAQdx Open Camera.vi"("error in"=w1740, "Session In"=w1752) -> ("error out"=w1749:errorcluster, "Session Out"=w1751:T3)  [unwired: 8 in]
            n1621 = call <vilib>:"IMAQdx Configure Grab.vi"("error in"=w1749, "Session In"=w1751) -> ("error out"=w1747:errorcluster, "Session Out"=w1750:T3)  [unwired: 8 in]
            n1622 = property on="摄像头选择" class="IMAQdx (strict)"("DisabledEnum"=T4."Disabled and Grayed Out" ("禁用")) -> ()  [unwired: 2 in, 2 out]
            n1623 = call "IMAQ Create"("Image Name"="image2", "Image Type"=w1739) -> ("New Image"=w1742:T2)  [unwired: 3 in, 1 out]
            n1624 = call "IMAQ Create"("Image Name"="image1", "Image Type"=w1744, "error in (no error)"=w1747) -> ("New Image"=w1745:T2, "error out"=w1746:errorcluster)  [unwired: 2 in]
            n1625 = while {
              tunnel: w1750 -> [w1765]
              tunnel: w1746 -> [w1767]
              tunnel: w1745 -> [w1766]
              tunnel: w1742 -> [w1756]
              tunnel: w1741 -> [w1763]
              tunnel: [w1759] -> w1738
              tunnel: [w1757] -> w1737
              stop <- w1758 continue-if-true
              w1764 = 5 items=["Red", "Green", "Blue", "Hue", "Saturation", "Luminance", "Value", "Intensity"] ("Color Plane")
              n1626 = call <vilib>:"IMAQdx Grab.vi"("error in"=w1767, "Image In"=w1766, "Session In"=w1765) -> ("error out"=w1760:errorcluster, "Image Out"=w1755:T2)  [unwired: 5 in, 2 out]
              "主界面 1" <- w1755
              n1627 = property on="摄像头开关" class="Bool (strict)"() -> ("Value"=w1754:bool)  [unwired: 2 in, 2 out]
              n1628 = Enqueue Element(queue=w1763, element=1, timeout in ms (-1)=10 ("超时毫秒(-1)")) -> ()  [unwired: 1 in, 3 out]
              n1629 = case shown="True" w1754 {
                tunnel: w1755 -> [_ w1768]
                frame False {
                }
                frame True {
                  n1630 = Get Date/Time In Seconds() -> (seconds since 1Jan1904=w1786:timestamp)
                  n1631 = Format Date/Time String(time format string (%c)="%Y%m%d%H%M%S%3u", seconds (now)=w1786) -> (date/time string=w1785:string)  [unwired: 1 in]
                  n1632 = Search/Split String(string=w1785, search string/char (-)=".") -> (substring before match=w1783:string, match + rest of string=w1784:string)  [unwired: 1 in, 1 out]
                  n1633 = Current VI's Path() -> (path=w1780:path)
                  n1634 = Strip Path(path=w1780) -> (stripped path=w1779:path)  [unwired: 1 out]
                  n1635 = String Subset(string=w1784, offset (0)=1) -> (substring=w1782:string)  [unwired: 1 in]
                  n1636 = Concatenate Strings(w1783, w1782) -> (w1781:string)
                  n1637 = Path To String(path=w1779) -> (string=w1778:string)
                  n1638 = Concatenate Strings(w1778, "\\Image save\\") -> (w1777:string)
                  n1639 = String To Path(string=w1777) -> (path=w1776:path)
                  n1640 = Concatenate Strings(w1781, ".PNG") -> (w1775:string)
                  n1641 = Build Path(base path=w1776, name or relative path=w1775) -> (appended path=w1774:path)
                  n1642 = call-poly "IMAQ Write File 2"("File Path"=w1774, "Image"=w1768) -> ()  [unwired: 8 in, 2 out]
                }
              }
              n1643 = call "IMAQ ExtractSingleColorPlane"("Color Plane"=w1764, "error in (no error)"=w1760, "Image Dst"=w1756, "Image Src"=w1755) -> ("error out"=w1759:errorcluster, "Image Dst Out"=w1757:T2)  [unwired: 6 in]
              n1644 = while {
                tunnel: w1757 -> [w1794]
                stop <- FALSE continue-if-true
                n1645 = property on="Tetragon" class="Arr (strict)"() -> ("Value"=w1787:cluster{"x":sgl, "y":sgl}[])  [unwired: 2 in, 2 out]
                n1646 = Wait (ms)(milliseconds to wait=100) -> ()  [unwired: 1 out]
                n1647 = property on="转换给模型的像素长宽大小" class="DigNum (strict)"() -> ("Value"=w1791:i32)  [unwired: 2 in, 2 out]
                n1648 = call-poly "IMAQ Extract Tetragon"("Tetragon"=w1787, "Image Src"=w1794) -> ("Image Dst Out"=w1789:T2)  [unwired: 8 in, 1 out]
                "主界面 2" <- w1789
                n1649 = call "IMAQ Resample"("X Resolution"=w1791, "Y Resolution"=w1791, "Image Src"=w1789) -> ("Image Dst Out"=w1792:T2)  [unwired: 7 in, 1 out]
                n1650 = call "IMAQ ImageToArray"("Image"=w1792) -> ("Image Pixels (U8)"=w1790:u8[][])  [unwired: 3 in, 4 out]
                n1651 = property on="用于存储单站图片转换后的单通道矩阵" class="Arr (strict)"("Val(Sgnl)"=w1790) -> ()  [unwired: 2 in, 2 out]
              }
              n1652 = property on="摄像头开关" class="Bool (strict)"() -> ("Value"=w1758:bool)  [unwired: 2 in, 2 out]
            }
            n1653 = call "IMAQ Dispose"("Image"=w1737) -> ()  [unwired: 5 in, 1 out]
          }
        }
      }
    }
    "error out 6" <- w1723
  }
  n1654 = call-poly "VISA Configure Serial Port"("VISA resource name"=refnum<visa-resource-name> "COM7", "baud rate (9600)"=u32 4800) -> ("VISA resource name out"=w54:refnum<visa-resource-name>, "error out"=w53:errorcluster)  [unwired: 12 in]
  n1655 = call-poly "VISA Configure Serial Port"("VISA resource name"=refnum<visa-resource-name> "COM5" ("过渡室真空"), "baud rate (9600)"=u32 9600, "data bits (8)"=u16 8, "parity (0:none)"=enum16{"None", "Odd", "Even", "Mark", "Space"}."None", "stop bits (10: 1 bit)"=w71) -> ("VISA resource name out"=w90:refnum<visa-resource-name>, "error out"=w89:errorcluster)  [unwired: 9 in]
  n1656 = call-poly "VISA Configure Serial Port"("VISA resource name"=refnum<visa-resource-name> "COM3" ("过渡室真空"), "baud rate (9600)"=u32 300, "data bits (8)"=u16 7, "parity (0:none)"=enum16{"None", "Odd", "Even", "Mark", "Space"}."None", "stop bits (10: 1 bit)"=w82) -> ("VISA resource name out"=w85:refnum<visa-resource-name>, "error out"=w84:errorcluster)  [unwired: 9 in]
  n1657 = Multiply(x=w58, y=w58) -> (x*y=w61:i32)
  n1658 = for {
    N: 1 -> [_]
    tunnel: w57 -> [w1814]
    tunnel: w57 -> [w1813]
    tunnel: w57 -> [w1812]
    w1802 = TRUE ("Value (Signaling)")
    w1796 = u8 0 ("Value (Signaling)")
    w1809 = 0.0 ("element")
    w1801 = "" ("Value (Signaling)")
    w1803 = sgl[] [] ("Value (Signaling)")
    w1800 = FALSE ("Value (Signaling)")
    w1804 = u8[] [0, 0, 0, 0, 0, 0, 0, 0, 0, 0, 0, 0, 0, 0, 0, 0, 0, 0, 0, 0, 0, 0, 0, 0] ("initialized array")
    n1659 = Initialize Array(w1814, w1813, w1812) -> (w1815:i32[][])
    n1660 = property on="In设定" class="Str"("Val(Sgnl)"="650" ("Value (Signaling)")) -> ()  [unwired: 2 in, 2 out]
    n1661 = property on="Temperature count Low" class="DigNum (strict)"("Val(Sgnl)"=w1796) -> ()  [unwired: 2 in, 2 out]
    n1662 = property on="Temperature count Suitable" class="DigNum (strict)"("Val(Sgnl)"=w1796) -> ()  [unwired: 2 in, 2 out]
    n1663 = property on="Temperature count High" class="DigNum (strict)"("Val(Sgnl)"=w1796) -> ()  [unwired: 2 in, 2 out]
    n1664 = property on="Countdow" class="DigNum (strict)"("Val(Sgnl)"=w1796) -> ()  [unwired: 2 in, 2 out]
    n1665 = property on="Temperature Switch" class="DigNum (strict)"("Val(Sgnl)"=w1796) -> ()  [unwired: 2 in, 2 out]
    n1666 = property on="Repetition" class="DigNum (strict)"("Val(Sgnl)"=w1796) -> ()  [unwired: 2 in, 2 out]
    n1667 = property on="Shutter count No" class="DigNum (strict)"("Val(Sgnl)"=w1796) -> ()  [unwired: 2 in, 2 out]
    n1668 = property on="Temperature count result" class="DigNum (strict)"("Val(Sgnl)"=w1796) -> ()  [unwired: 2 in, 2 out]
    n1669 = property on="Shutter count Yes" class="DigNum (strict)"("Val(Sgnl)"=w1796) -> ()  [unwired: 2 in, 2 out]
    n1670 = property on="Growth Switch" class="DigNum (strict)"("Val(Sgnl)"=w1796) -> ()  [unwired: 2 in, 2 out]
    n1671 = property on="Shutter count Yes result" class="DigNum (strict)"("Val(Sgnl)"=w1796) -> ()  [unwired: 2 in, 2 out]
    n1672 = property on="Reconstruction模型输出结果" class="Arr (strict)"("Val(Sgnl)"=w1803) -> ()  [unwired: 2 in, 2 out]
    n1673 = property on="Temperature模型输出结果" class="Arr (strict)"("Val(Sgnl)"=w1803) -> ()  [unwired: 2 in, 2 out]
    n1674 = property on="Shutter模型输出结果" class="Arr (strict)"("Val(Sgnl)"=w1803) -> ()  [unwired: 2 in, 2 out]
    n1675 = property on="MSE loss" class="Str"("Value"=w1801) -> ()  [unwired: 2 in, 2 out]
    n1676 = property on="Sub1" class="Str"("Value"=w1801) -> ()  [unwired: 2 in, 2 out]
    n1677 = property on="用于存储单站图片转换后的单通道矩阵" class="Arr (strict)"("Val(Sgnl)"=w1815) -> ()  [unwired: 2 in, 2 out]
    n1678 = property on="In速度" class="Str"("Val(Sgnl)"="2" ("Value (Signaling)")) -> ()  [unwired: 2 in, 2 out]
    n1679 = property on="Cooling" class="Bool (strict)"("Val(Sgnl)"=w1802) -> ()  [unwired: 2 in, 2 out]
    n1680 = property on="Surface InAs QDs" class="Bool (strict)"("Val(Sgnl)"=w1802) -> ()  [unwired: 2 in, 2 out]
    n1681 = property on="Ga2速度" class="Str"("Val(Sgnl)"="6" ("Value (Signaling)")) -> ()  [unwired: 2 in, 2 out]
    n1682 = property on="模型输出是否超过0.7概率是Ys" class="Bool (strict)"("Val(Sgnl)"=w1800) -> ()  [unwired: 2 in, 2 out]
    n1683 = property on="Heating to completely remove oxidation" class="Bool (strict)"("Val(Sgnl)"=w1800) -> ()  [unwired: 2 in, 2 out]
    n1684 = property on="Is the probability of the model output (n×6) exceeding" class="Bool (strict)"("Val(Sgnl)"=w1800) -> ()  [unwired: 2 in, 2 out]
    n1685 = property on="Ready for GaAs buffer 0.6 μm/h" class="Bool (strict)"("Val(Sgnl)"=w1800) -> ()  [unwired: 2 in, 2 out]
    n1686 = property on="While loop for cool to less than 100 ℃" class="Bool (strict)"("Val(Sgnl)"=w1800) -> ()  [unwired: 2 in, 2 out]
    n1687 = property on="Start" class="Bool (strict)"("Val(Sgnl)"=w1800) -> ()  [unwired: 2 in, 2 out]
    n1688 = property on="Temperature adjustment 1" class="Bool (strict)"("Val(Sgnl)"=w1800) -> ()  [unwired: 2 in, 2 out]
    n1689 = property on="Inside InAs QDs" class="Bool (strict)"("Val(Sgnl)"=w1800) -> ()  [unwired: 2 in, 2 out]
    n1690 = property on="Is the probability of the model output deoxidization exceeding" class="Bool (strict)"("Val(Sgnl)"=w1800) -> ()  [unwired: 2 in, 2 out]
    n1691 = property on="10 nm GaAs cap layer 0.36 μm/h" class="Bool (strict)"("Val(Sgnl)"=w1800) -> ()  [unwired: 2 in, 2 out]
    n1692 = property on="Surface InAs QDs for AFM" class="Bool (strict)"("Value"=w1800) -> ()  [unwired: 2 in, 2 out]
    n1693 = property on="GaAs buffer 0.6 μm/h" class="Bool (strict)"("Val(Sgnl)"=w1800) -> ()  [unwired: 2 in, 2 out]
    n1694 = property on="Is the probability of the model output oxidization exceeding" class="Bool (strict)"("Val(Sgnl)"=w1800) -> ()  [unwired: 2 in, 2 out]
    n1695 = property on="Obtain Growth Temperature" class="Bool (strict)"("Val(Sgnl)"=w1800) -> ()  [unwired: 2 in, 2 out]
    n1696 = property on="Model switch" class="Bool (strict)"("Val(Sgnl)"=w1800) -> ()  [unwired: 2 in, 2 out]
    n1697 = property on="Is the probability of the model output As cap exceeding" class="Bool (strict)"("Val(Sgnl)"=w1800) -> ()  [unwired: 2 in, 2 out]
    n1698 = property on="Whether to continue heating up operation" class="Bool (strict)"("Val(Sgnl)"=w1800) -> ()  [unwired: 2 in, 2 out]
    n1699 = property on="倒计时开关" class="Bool (strict)"("Val(Sgnl)"=w1800) -> ()  [unwired: 2 in, 2 out]
    n1700 = property on="Is the probability of the model output c(4×4) exceeding" class="Bool (strict)"("Val(Sgnl)"=w1800) -> ()  [unwired: 2 in, 2 out]
    n1701 = property on="Cool to less than 100 ℃ and wait 20 minutes" class="Bool (strict)"("Val(Sgnl)"=w1800) -> ()  [unwired: 2 in, 2 out]
    n1702 = property on="GaAs buffer 0.6 μm/h  2" class="Bool (strict)"("Val(Sgnl)"=w1800) -> ()  [unwired: 2 in, 2 out]
    n1703 = property on="摄像头开关" class="Bool (strict)"("Val(Sgnl)"=w1800) -> ()  [unwired: 2 in, 2 out]
    n1704 = property on="If In Shutter can be closed 1" class="Bool (strict)"("Val(Sgnl)"=w1800) -> ()  [unwired: 2 in, 2 out]
    n1705 = property on="Is the probability of the model output (2×4) exceeding" class="Bool (strict)"("Val(Sgnl)"=w1800) -> ()  [unwired: 2 in, 2 out]
    n1706 = property on="Temperature adjustment 2" class="Bool (strict)"("Val(Sgnl)"=w1800) -> ()  [unwired: 2 in, 2 out]
    n1707 = property on="Temperature adjustment 3" class="Bool (strict)"("Val(Sgnl)"=w1800) -> ()  [unwired: 2 in, 2 out]
    n1708 = property on="Obtaining the deoxidation temperature" class="Bool (strict)"("Val(Sgnl)"=w1800) -> ()  [unwired: 2 in, 2 out]
    n1709 = property on="Whether to continue heat up for reconstruction" class="Bool (strict)"("Val(Sgnl)"=w1800) -> ()  [unwired: 2 in, 2 out]
    n1710 = property on="GaAs buffer 0.6 μm/h" class="Bool (strict)"("Val(Sgnl)"=w1800) -> ()  [unwired: 2 in, 2 out]
    n1711 = property on="Obtaining the reconstruction  temperature" class="Bool (strict)"("Val(Sgnl)"=w1800) -> ()  [unwired: 2 in, 2 out]
    n1712 = property on="Sub速度" class="Str"("Val(Sgnl)"="10" ("Value (Signaling)")) -> ()  [unwired: 2 in, 2 out]
    n1713 = property on="转换给模型的像素长宽大小" class="DigNum (strict)"() -> ("Value"=w1807:i32)  [unwired: 2 in, 2 out]
    n1714 = property on="选择多少张图片（通道）" class="DigNum (strict)"() -> ("Value"=w1808:i32)  [unwired: 2 in, 2 out]
    n1715 = property on="Sub1 3" class="Str"("Val(Sgnl)"=w1801) -> ()  [unwired: 2 in, 2 out]
    n1716 = property on="Deoxidation temperature" class="Str"("Val(Sgnl)"=w1801) -> ()  [unwired: 2 in, 2 out]
    n1717 = property on="Sub2" class="Str"("Val(Sgnl)"=w1801) -> ()  [unwired: 2 in, 2 out]
    n1718 = property on="Optimize Sub Temperature 2" class="Str"("Val(Sgnl)"=w1801) -> ()  [unwired: 2 in, 2 out]
    n1719 = property on="Reminder Information" class="Str"("Val(Sgnl)"=w1801) -> ()  [unwired: 2 in, 2 out]
    n1720 = property on="Substrate to find Reconstruction temperature" class="Str"("Val(Sgnl)"=w1801) -> ()  [unwired: 2 in, 2 out]
    n1721 = property on="Sub1 2" class="Str"("Val(Sgnl)"=w1801) -> ()  [unwired: 2 in, 2 out]
    n1722 = property on="Optimize Sub Temperature 1" class="Str"("Val(Sgnl)"=w1801) -> ()  [unwired: 2 in, 2 out]
    n1723 = property on="Substrate to find Deoxidation temperature" class="Str"("Val(Sgnl)"=w1801) -> ()  [unwired: 2 in, 2 out]
    n1724 = property on="From As cap to c(4×4)" class="Str"("Val(Sgnl)"=w1801) -> ()  [unwired: 2 in, 2 out]
    n1725 = property on="Sub3" class="Str"("Val(Sgnl)"=w1801) -> ()  [unwired: 2 in, 2 out]
    n1726 = property on="Reconstruction模型输出结果" class="Str"("Val(Sgnl)"=w1801) -> ()  [unwired: 2 in, 2 out]
    n1727 = property on="From c(4×4) to (2×4)" class="Str"("Val(Sgnl)"=w1801) -> ()  [unwired: 2 in, 2 out]
    n1728 = property on="Temperature模型输出结果 2" class="Str"("Val(Sgnl)"=w1801) -> ()  [unwired: 2 in, 2 out]
    n1729 = property on="A =" class="Str"("Val(Sgnl)"=w1801) -> ()  [unwired: 2 in, 2 out]
    n1730 = property on="C =" class="Str"("Val(Sgnl)"=w1801) -> ()  [unwired: 2 in, 2 out]
    n1731 = property on="InAs growth temperature" class="Str"("Val(Sgnl)"=w1801) -> ()  [unwired: 2 in, 2 out]
    n1732 = property on="From (2×4) to (n×6)" class="Str"("Val(Sgnl)"=w1801) -> ()  [unwired: 2 in, 2 out]
    n1733 = property on="GaAs growth temperature" class="Str"("Val(Sgnl)"=w1801) -> ()  [unwired: 2 in, 2 out]
    n1734 = property on="Shutter模型输出结果" class="Str"("Val(Sgnl)"=w1801) -> ()  [unwired: 2 in, 2 out]
    n1735 = property on="B =" class="Str"("Val(Sgnl)"=w1801) -> ()  [unwired: 2 in, 2 out]
    n1736 = property on="Sub4" class="Str"("Val(Sgnl)"=w1801) -> ()  [unwired: 2 in, 2 out]
    n1737 = Initialize Array(w1809, w1808, w1807, w1807) -> (w1811:dbl[][][])
    n1738 = property on="多张图片拼接后的多维数组" class="Arr (strict)"("Val(Sgnl)"=w1811) -> ()  [unwired: 2 in, 2 out]
    n1739 = Initialize Array(w1809, 1 ("dimension size"), w1808, w1807, w1807) -> (w1805:dbl[][][][])
    n1740 = property on="Tab Control" class="TabCtl (strict)"("Value"=T1."Growth Temperature Initialization" ("Tab Control")) -> ()  [unwired: 2 in, 2 out]
    n1741 = property on="经过python转换后的数组" class="Arr (strict)"("Val(Sgnl)"=w1805) -> ()  [unwired: 2 in, 2 out]
    n1742 = property on="记录Reconstruction模型的连续24个输出结果" class="Arr (strict)"("Val(Sgnl)"=w1804) -> ()  [unwired: 2 in, 2 out]
    n1743 = property on="记录Temperature模型的连续24个输出结果" class="Arr (strict)"("Val(Sgnl)"=w1804) -> ()  [unwired: 2 in, 2 out]
    n1744 = property on="记录Shutter模型的连续24个输出结果" class="Arr (strict)"("Val(Sgnl)"=w1804) -> ()  [unwired: 2 in, 2 out]
  }
  n1745 = while {
    tunnel: w54 -> [w1828]
    tunnel: w53 -> [w1827]
    tunnel: [w1826] -> w52
    tunnel: [w1825] -> w51
    stop <- FALSE ("停止") stop-if-true
    w1816 = FALSE  # Si
    w1817 = FALSE  # Al2
    w1818 = FALSE  # Be
    w1819 = FALSE  # Al1
    w1820 = FALSE  # Ga1
    n1746 = property on="Main挡板" class="Bool (strict)"() -> ("Value"=w1824:bool)  [unwired: 2 in, 2 out]
    n1747 = case shown="True" w1824 {
      tunnel: [0 8] -> w1851
      frame False {
      }
      frame True {
      }
    }
    n1748 = property on="Ga2挡板" class="Bool (strict)"() -> ("Value"=w1823:bool)  [unwired: 2 in, 2 out]
    n1749 = Add(x=w1851, y=80) -> (x+y=w1845:i32)
    n1750 = Number To Hexadecimal String(2:w1845) -> (0:w1846:string)  [unwired: 1 in]
    n1751 = case shown="True" w1823 {
      tunnel: [0 1] -> w1859
      frame False {
      }
      frame True {
      }
    }
    n1752 = case shown="True" w1820 {
      tunnel: [0 2] -> w1860
      frame False {
      }
      frame True {
      }
    }
    n1753 = case shown="True" w1819 {
      tunnel: [0 4] -> w1862
      frame False {
      }
      frame True {
      }
    }
    n1754 = property on="In挡板" class="Bool (strict)"() -> ("Value"=w1822:bool)  [unwired: 2 in, 2 out]
    n1755 = String Length ("字符串长度")(string=w1846) -> (length=w1850:i32)
    n1756 = case shown="True" w1822 {
      tunnel: [0 8] -> w1863
      frame False {
      }
      frame True {
      }
    }
    n1757 = Divide(x=w1850, y=2) -> (x/y=w1848:dbl)
    n1758 = Add(x=w1859, y=w1860) -> (x+y=w1861:i32)
    n1759 = Add(x=w1861, y=w1862) -> (x+y=w1864:i32)
    n1760 = for {
      N: w1848 -> [_]
      shift-right: [w1913] -> w1841
      shift-left: "" -> [w1922]
      tunnel: w1846 -> [w1921]
      i -> [w1920]
      w1918 = 2
      n1761 = Multiply(x=w1918, y=w1920) -> (x*y=w1919:i32)
      n1762 = String Subset(string=w1921, offset (0)=w1919, length (rest)=w1918) -> (substring=w1923:string)
      n1763 = Hexadecimal String To Number(string=w1923) -> (number=w1917:u32)  [unwired: 2 in, 1 out]
      n1764 = Build Array(w1917) -> (w1916:u32[])
      n1765 = To Unsigned Byte Integer(number=w1916) -> (unsigned 8bit integer=w1915:u8[])
      n1766 = Byte Array To String(unsigned byte array=w1915) -> (string=w1914:string)
      n1767 = Concatenate Strings(w1922, w1914) -> (w1913:string)
    }
    "String 2" <- w1841
    n1768 = Add(x=w1864, y=w1863) -> (x+y=w1865:i32)
    n1769 = case shown="True" w1818 {
      tunnel: [0 1] -> w1843
      frame False {
      }
      frame True {
      }
    }
    n1770 = case shown="True" w1817 {
      tunnel: [0 2] -> w1844
      frame False {
      }
      frame True {
      }
    }
    n1771 = Add(x=w1865, y=64) -> (x+y=w1853:i32)
    n1772 = case shown="True" w1816 {
      tunnel: [0 4] -> w1877
      frame False {
      }
      frame True {
      }
    }
    n1773 = property on="As挡板" class="Bool (strict)"() -> ("Value"=w1821:bool)  [unwired: 2 in, 2 out]
    n1774 = Number To Hexadecimal String(2:w1853) -> (0:w1854:string)  [unwired: 1 in]
    n1775 = String Length ("字符串长度")(string=w1854) -> (length=w1858:i32)
    n1776 = case shown="True" w1821 {
      tunnel: [0 8] -> w1876
      frame False {
      }
      frame True {
      }
    }
    n1777 = Add(x=w1843, y=w1844) -> (x+y=w1842:i32)
    n1778 = Divide(x=w1858, y=2) -> (x/y=w1856:dbl)
    n1779 = Add(x=w1842, y=w1877) -> (x+y=w1875:i32)
    n1780 = Add(x=w1875, y=w1876) -> (x+y=w1874:i32)
    n1781 = for {
      N: w1856 -> [_]
      shift-right: [w1926] -> w1836
      shift-left: "" -> [w1935]
      tunnel: w1854 -> [w1934]
      i -> [w1933]
      w1931 = 2
      n1782 = Multiply(x=w1931, y=w1933) -> (x*y=w1932:i32)
      n1783 = String Subset(string=w1934, offset (0)=w1932, length (rest)=w1931) -> (substring=w1936:string)
      n1784 = Hexadecimal String To Number(string=w1936) -> (number=w1930:u32)  [unwired: 2 in, 1 out]
      n1785 = Build Array(w1930) -> (w1929:u32[])
      n1786 = To Unsigned Byte Integer(number=w1929) -> (unsigned 8bit integer=w1928:u8[])
      n1787 = Byte Array To String(unsigned byte array=w1928) -> (string=w1927:string)
      n1788 = Concatenate Strings(w1935, w1927) -> (w1926:string)
    }
    n1789 = Add(x=w1874, y=48) -> (x+y=w1867:i32)
    n1790 = Number To Hexadecimal String(2:w1867) -> (0:w1868:string)  [unwired: 1 in]
    n1791 = String Length ("字符串长度")(string=w1868) -> (length=w1872:i32)
    n1792 = flat-sequence {
      tunnel: w1841 -> [w1883]
      tunnel: [w1882] -> w1840
      tunnel: [w1881] -> w1839
      tunnel: w1828 -> [w1880]
      tunnel: w1827 -> [w1879]
      tunnel: w1840 -> [w1888]
      tunnel: w1839 -> [w1887]
      tunnel: [w1886] -> w1838
      tunnel: [w1885] -> w1837
      tunnel: w1838 -> [w1894]
      tunnel: w1837 -> [w1892]
      tunnel: w1836 -> [w1893]
      tunnel: [w1891] -> w1835
      tunnel: [w1890] -> w1834
      tunnel: w1835 -> [w1899]
      tunnel: w1834 -> [w1898]
      tunnel: [w1897] -> w1833
      tunnel: [w1896] -> w1832
      tunnel: w1833 -> [w1905]
      tunnel: w1832 -> [w1903]
      tunnel: w1831 -> [w1904]
      tunnel: [w1902] -> w1830
      tunnel: [w1901] -> w1829
      tunnel: w1830 -> [w1910]
      tunnel: w1829 -> [w1909]
      tunnel: [w1907] -> w1825
      tunnel: [w1906] -> w1826
      frame #0 {
        n1793 = VISA Write "VISA写入"(VISA resource name=w1880, write buffer=w1883, error in (no error)=w1879) -> (VISA resource name out=w1881:refnum<visa-resource-name>, error out=w1882:errorcluster)  [unwired: 1 out]
      }
      frame #1 {
        n1794 = VISA Read(VISA resource name=w1887, byte count=u32 4, error in (no error)=w1888) -> (VISA resource name out=w1885:refnum<visa-resource-name>, error out=w1886:errorcluster)  [unwired: 2 out]
      }
      frame #2 {
        n1795 = VISA Write "VISA写入"(VISA resource name=w1892, write buffer=w1893, error in (no error)=w1894) -> (VISA resource name out=w1890:refnum<visa-resource-name>, error out=w1891:errorcluster)  [unwired: 1 out]
        n1796 = Wait (ms)(milliseconds to wait=25) -> ()  [unwired: 1 out]
      }
      frame #3 {
        n1797 = VISA Read(VISA resource name=w1898, byte count=u32 4, error in (no error)=w1899) -> (VISA resource name out=w1896:refnum<visa-resource-name>, error out=w1897:errorcluster)  [unwired: 2 out]
      }
      frame #4 {
        n1798 = VISA Write "VISA写入"(VISA resource name=w1903, write buffer=w1904, error in (no error)=w1905) -> (VISA resource name out=w1901:refnum<visa-resource-name>, error out=w1902:errorcluster)  [unwired: 1 out]
        n1799 = Wait (ms)(milliseconds to wait=25) -> ()  [unwired: 1 out]
      }
      frame #5 {
        n1800 = VISA Read "VISA读取"(VISA resource name=w1909, byte count=u32 4, error in (no error)=w1910) -> (VISA resource name out=w1907:refnum<visa-resource-name>, error out=w1906:errorcluster)  [unwired: 2 out]
      }
    }
    n1801 = Divide(x=w1872, y=2) -> (x/y=w1870:dbl)
    n1802 = for {
      N: w1870 -> [_]
      shift-right: [w1945] -> w1831
      shift-left: "" -> [w1954]
      tunnel: w1868 -> [w1953]
      i -> [w1952]
      w1950 = 2
      n1803 = Multiply(x=w1950, y=w1952) -> (x*y=w1951:i32)
      n1804 = String Subset(string=w1953, offset (0)=w1951, length (rest)=w1950) -> (substring=w1955:string)
      n1805 = Hexadecimal String To Number(string=w1955) -> (number=w1949:u32)  [unwired: 2 in, 1 out]
      n1806 = Build Array(w1949) -> (w1948:u32[])
      n1807 = To Unsigned Byte Integer(number=w1948) -> (unsigned 8bit integer=w1947:u8[])
      n1808 = Byte Array To String(unsigned byte array=w1947) -> (string=w1946:string)
      n1809 = Concatenate Strings(w1954, w1946) -> (w1945:string)
    }
  }
  n1810 = while {
    shift-right: [w1964] -> w88
    shift-left: w90 -> [w1968]
    shift-right: [w1965] -> w87
    shift-left: w89 -> [w1967]
    stop <- FALSE stop-if-true
    n1811 = flat-sequence {
      tunnel: w1968 -> [w1974]
      tunnel: w1967 -> [w1973]
      tunnel: [w1976] -> w1963
      tunnel: [w1975] -> w1962
      tunnel: w1963 -> [w1979]
      tunnel: w1962 -> [w1980]
      tunnel: [w1981] -> w1965
      tunnel: [w1978] -> w1964
      frame #0 {
        n1812 = Wait (ms)(milliseconds to wait=700) -> ()  [unwired: 1 out]
        n1813 = Concatenate Strings("#RD", "\r") -> (w1970:string)
        n1814 = VISA Write "VISA写入"(VISA resource name=w1974, write buffer=w1970, error in (no error)=w1973) -> (VISA resource name out=w1976:refnum<visa-resource-name>, error out=w1975:errorcluster)  [unwired: 1 out]
      }
      frame #1 {
        n1815 = property class="Instr"(reference=w1979, error in=w1980) -> (reference out=w1984:refnum<visa-resource-name>, error out=w1985:errorcluster, "Bytes at Port"=w1986:u32)
        n1816 = VISA Read "VISA读取"(VISA resource name=w1984, byte count=w1986, error in (no error)=w1985) -> (VISA resource name out=w1978:refnum<visa-resource-name>, read buffer=w1987:string, error out=w1981:errorcluster)  [unwired: 1 out]
        n1817 = String Subset(string=w1987, offset (0)=u16 1 ("data bits (8)"), length (rest)=u16 9 ("data bits (8)")) -> (substring=w1977:string)
        "0 Buffer真空度(字符串)" <- w1977
        n1818 = Fract/Exp String To Number(string=w1977) -> (number=→"Buffer vacuum":dbl)  [unwired: 3 in, 1 out]
      }
    }
  }
  n1819 = while {
    tunnel: w85 -> [w1995]
    tunnel: w84 -> [w1994]
    tunnel: [w1992] -> w77
    tunnel: [w1991] -> w76
    stop <- FALSE stop-if-true
    n1820 = flat-sequence {
      tunnel: w1995 -> [w2001]
      tunnel: w1994 -> [w2000]
      tunnel: [w1999] -> w1990
      tunnel: [w1998] -> w1989
      tunnel: w1990 -> [w2004]
      tunnel: w1989 -> [w2003]
      tunnel: [w2007] -> w1992
      tunnel: [w2006] -> w1991
      frame #0 {
        n1821 = Wait (ms)(milliseconds to wait=100) -> ()  [unwired: 1 out]
        n1822 = VISA Write "VISA写入"(VISA resource name=w2001, write buffer="DSIG\n", error in (no error)=w2000) -> (VISA resource name out=w1999:refnum<visa-resource-name>, error out=w1998:errorcluster)  [unwired: 1 out]
      }
      frame #1 {
        n1823 = VISA Read "VISA读取"(VISA resource name=w2004, byte count=u32 16, error in (no error)=w2003) -> (VISA resource name out=w2006:refnum<visa-resource-name>, read buffer=w2010:string, error out=w2007:errorcluster)  [unwired: 1 out]
        n1824 = String Subset(string=w2010, offset (0)=u16 0 ("data bits (8)"), length (rest)=u16 8 ("data bits (8)")) -> (substring=w2005:string)
        "0 Growth真空度（字符串）" <- w2005
        n1825 = Fract/Exp String To Number(string=w2005) -> (number=→"Growth vacuum":dbl)  [unwired: 3 in, 1 out]
      }
    }
  }
  n1826 = Multiply(x=w59, y=w61) -> (x*y=w60:i32)
  n1827 = while {
    shift-right: [w2021] -> _
    shift-left: _ -> [w2022]
    tunnel: w61 -> [w2017]
    tunnel: w60 -> [w2018]
    tunnel: w59 -> [w2016]
    tunnel: w58 -> [w2015]
    tunnel: w58 -> [w2014]
    stop <- FALSE stop-if-true
    n1828 = Reshape Array(w2022, w2018) -> (w2023:dbl[])
    n1829 = property on="用于存储单站图片转换后的单通道矩阵" class="Arr (strict)"() -> ("Value"=w2013:dbl[][])  [unwired: 2 in, 2 out]
    n1830 = Wait (ms)(milliseconds to wait=100) -> ()  [unwired: 1 out]
    n1831 = Delete From Array(array=w2023, length=w2017, index=0 ("索引")) -> (array with subset deleted=w2026:dbl[])  [unwired: 1 out]
    n1832 = Reshape Array(w2013, w2017) -> (w2025:dbl[])
    n1833 = Build Array(w2026, w2025) -> (w2024:dbl[][])
    n1834 = Reshape Array(w2024, w2018) -> (w2021:dbl[])
    n1835 = Reshape Array(w2021, w2016, w2015, w2014) -> (w2012:dbl[][][])
    n1836 = property on="多张图片拼接后的多维数组" class="Arr (strict)"("Val(Sgnl)"=w2012) -> ()  [unwired: 2 in, 2 out]
  }
  n1837 = Current VI's Path() -> (path=w46:path)
  n1838 = Strip Path(path=w46) -> (stripped path=w45:path)  [unwired: 1 out]
  n1839 = Open Python Session(python version="3.9" ("Python版本"), python path=path "C:/Users/meiyo/anaconda3/envs/pytorchnn/python.exe" ("Python path")) -> (session out=w48:refnum<k35>, error out=w47:errorcluster)  [unwired: 1 in]
  n1840 = property on="转换给模型的像素长宽大小" class="DigNum (strict)"() -> ("Value"=w37:i32)  [unwired: 2 in, 2 out]
  n1841 = property on="转换给模型的像素长宽大小" class="DigNum (strict)"() -> ("Value"=w22:i32)  [unwired: 2 in, 2 out]
  n1842 = property on="转换给模型的像素长宽大小" class="DigNum (strict)"() -> ("Value"=w5:i32)  [unwired: 2 in, 2 out]
  n1843 = Build Path(base path=w45, name or relative path=".\\main.py") -> (appended path=w44:path)
  n1844 = property on="选择多少张图片（通道）" class="DigNum (strict)"() -> ("Value"=w38:i32)  [unwired: 2 in, 2 out]
  n1845 = property on="选择多少张图片（通道）" class="DigNum (strict)"() -> ("Value"=w23:i32)  [unwired: 2 in, 2 out]
  n1846 = property on="选择多少张图片（通道）" class="DigNum (strict)"() -> ("Value"=w4:i32)  [unwired: 2 in, 2 out]
  n1847 = while {
    tunnel: w44 -> [w2034]
    tunnel: "change_channel" ("函数名称") -> [w2033]
    shift-right: [w2038] -> w50
    shift-left: w48 -> [w2036]
    shift-right: [w2037] -> w49
    shift-left: w47 -> [w2035]
    stop <- FALSE stop-if-true
    n1848 = property on="多张图片拼接后的多维数组" class="Arr (strict)"() -> ("Value"=w2029:dbl[][][])  [unwired: 2 in, 2 out]
    n1849 = Wait (ms)(milliseconds to wait=100) -> ()  [unwired: 1 out]
    n1850 = node(w2036, w2034, w2033, w2035, dbl[][][][] [] ("input parameter"), w2029) -> (w2038:refnum<k35>, w2037:errorcluster, w2031:dbl[][][][])  [unwired: 1 in, 2 out]
    n1851 = property on="经过python转换后的数组" class="Arr (strict)"("Val(Sgnl)"=w2031) -> ()  [unwired: 2 in, 2 out]
  }
  n1852 = Current VI's Path() -> (path=w36:path)
  n1853 = Current VI's Path() -> (path=w21:path)
  n1854 = Current VI's Path() -> (path=w6:path)
  n1855 = Strip Path(path=w36) -> (stripped path=w35:path)  [unwired: 1 out]
  n1856 = Strip Path(path=w21) -> (stripped path=w20:path)  [unwired: 1 out]
  n1857 = Strip Path(path=w6) -> (stripped path=w7:path)  [unwired: 1 out]
  n1858 = Multiply(x=w37, y=w37) -> (x*y=w39:i32)
  n1859 = Build Path(base path=w35, name or relative path=".\\Temperature_model.onnx") -> (appended path=w34:path)
  n1860 = Multiply(x=w22, y=w22) -> (x*y=w24:i32)
  n1861 = Multiply(x=w5, y=w5) -> (x*y=w3:i32)
  n1862 = Build Path(base path=w20, name or relative path=".\\Shutter_model.onnx") -> (appended path=w19:path)
  n1863 = Build Path(base path=w7, name or relative path=".\\Reconstruction_model.onnx") -> (appended path=w8:path)
  n1864 = Multiply(x=w38, y=w39) -> (x*y=w31:i32)
  n1865 = call <vilib>:"Create_Session.vi"("type"=enum16{"CPU", "CUDA", "TensorRT"}."TensorRT", "path"=w34) -> ("error out"=w30:errorcluster, "Session out"=w29:refnum<class "Session.lvclass">)  [unwired: 8 in]
  n1866 = Multiply(x=w23, y=w24) -> (x*y=w16:i32)
  n1867 = Multiply(x=w4, y=w3) -> (x*y=w11:i32)
  n1868 = call <vilib>:"Create_Session.vi"("type"=enum16{"CPU", "CUDA", "TensorRT"}."TensorRT", "path"=w19) -> ("error out"=w15:errorcluster, "Session out"=w14:refnum<class "Session.lvclass">)  [unwired: 8 in]
  n1869 = call <vilib>:"Create_Session.vi"("type"=enum16{"CPU", "CUDA", "TensorRT"}."TensorRT", "path"=w8) -> ("error out"=w12:errorcluster, "Session out"=w13:refnum<class "Session.lvclass">)  [unwired: 8 in]
  n1870 = while {
    tunnel: w31 -> [w2045]
    tunnel: w30 -> [w2044]
    tunnel: w29 -> [w2043]
    tunnel: [w2042] -> w28
    tunnel: [w2041] -> w27
    stop <- FALSE stop-if-true
    n1871 = property on="Tab Control" class="TabCtl (strict)"() -> ("Value"=w2040:T1)  [unwired: 2 in, 2 out]
    n1872 = case shown="\"Growth Temperature Initialization\", Default" w2040 {
      tunnel: [FALSE ("Value") w2048] -> w2039
      frame "Growth Temperature Initialization", Default {
      }
      frame "InAs/GaAs QDs on GaAs substrates" {
        n1873 = property on="Model switch" class="Bool (strict)"() -> ("Value"=w2048:bool)  [unwired: 2 in, 2 out]
      }
    }
    n1874 = case shown="True" w2039 {
      tunnel: w2045 -> [_ w2071]
      tunnel: w2043 -> [w2050 w2070]
      tunnel: w2044 -> [w2049 w2069]
      tunnel: [w2050 w2068] -> w2041
      tunnel: [w2049 w2067] -> w2042
      frame False {
      }
      frame True {
        n1875 = property on="经过python转换后的数组" class="Arr (strict)"() -> ("Value"=w2062:dbl[][][][])  [unwired: 2 in, 2 out]
        n1876 = property on="记录Temperature模型的连续24个输出结果" class="Arr (strict)"() -> ("Value"=w2055:u8[])  [unwired: 2 in, 2 out]
        n1877 = Array Size(array=w2062) -> (size(s)=w2063:i32[])
        n1878 = Reshape Array(w2062, w2071) -> (w2061:dbl[])
        n1879 = call <vilib>:"Run_one_input_data.vi"("error in (no error)"=w2069, "data"=w2061, "shape"=w2063, "Session in"=w2070) -> ("error out"=w2066:errorcluster, "Session out"=w2065:refnum<class "Session.lvclass">)  [unwired: 5 in, 1 out]
        n1880 = call-poly <vilib>:"Get_result.vi"("error in (no error)"=w2066, "index"=0, "Session in"=w2065) -> ("error out"=w2067:errorcluster, "data"=w2051:sgl[], "Session out"=w2068:refnum<class "Session.lvclass">)  [unwired: 5 in, 1 out]
        n1881 = property on="Temperature模型输出结果" class="Arr (strict)"("Val(Sgnl)"=w2051) -> ()  [unwired: 2 in, 2 out]
        n1882 = Array Max & Min(array=w2051) -> (max index (indices)=w2056:i32)  [unwired: 3 out]
        n1883 = Delete From Array(array=w2055, length=1 ("长度"), index=0 ("索引")) -> (array with subset deleted=w2060:u8[])  [unwired: 1 out]
        n1884 = property on="dimension size" class="DigNum (strict)"() -> ("Value"=w2052:i32)  [unwired: 2 in, 2 out]
        n1885 = case "条件结构" shown="2" w2056 {
          tunnel: ["High" "Low" "Suitable"] -> w2053
          frame 0, Default {
          }
          frame 1 {
          }
          frame 2 {
          }
        }
        n1886 = Build Array (concatenate)(w2060, w2056) -> (w2059:i32[])
        n1887 = Reshape Array(w2059, w2052) -> (w2054:i32[])
        n1888 = property on="记录Temperature模型的连续24个输出结果" class="Arr (strict)"("Val(Sgnl)"=w2054) -> ()  [unwired: 2 in, 2 out]
        n1889 = property on="Temperature模型输出结果 2" class="Str"("Val(Sgnl)"=w2053) -> ()  [unwired: 2 in, 2 out]
      }
    }
  }
  n1890 = while {
    tunnel: [w2081] -> w26
    tunnel: [w2080] -> w25
    tunnel: w16 -> [w2079]
    tunnel: w15 -> [w2078]
    tunnel: w14 -> [w2077]
    stop <- FALSE stop-if-true
    n1891 = property on="Tab Control" class="TabCtl (strict)"() -> ("Value"=w2076:T1)  [unwired: 2 in, 2 out]
    n1892 = case shown="\"InAs/GaAs QDs on GaAs substrates\"" w2076 {
      tunnel: [FALSE ("Value") w2084] -> w2075
      frame "Growth Temperature Initialization", Default {
      }
      frame "InAs/GaAs QDs on GaAs substrates" {
        n1893 = property on="Model switch" class="Bool (strict)"() -> ("Value"=w2084:bool)  [unwired: 2 in, 2 out]
      }
    }
    n1894 = case shown="True" w2075 {
      tunnel: w2079 -> [_ w2107]
      tunnel: w2077 -> [w2086 w2106]
      tunnel: w2078 -> [w2085 w2105]
      tunnel: [w2086 w2104] -> w2080
      tunnel: [w2085 w2103] -> w2081
      frame False {
      }
      frame True {
        n1895 = property on="经过python转换后的数组" class="Arr (strict)"() -> ("Value"=w2098:dbl[][][][])  [unwired: 2 in, 2 out]
        n1896 = property on="记录Shutter模型的连续24个输出结果" class="Arr (strict)"() -> ("Value"=w2092:u8[])  [unwired: 2 in, 2 out]
        n1897 = Array Size(array=w2098) -> (size(s)=w2099:i32[])
        n1898 = Reshape Array(w2098, w2107) -> (w2097:dbl[])
        n1899 = call <vilib>:"Run_one_input_data.vi"("error in (no error)"=w2105, "data"=w2097, "shape"=w2099, "Session in"=w2106) -> ("error out"=w2102:errorcluster, "Session out"=w2101:refnum<class "Session.lvclass">)  [unwired: 5 in, 1 out]
        n1900 = call-poly <vilib>:"Get_result.vi"("error in (no error)"=w2102, "index"=0, "Session in"=w2101) -> ("error out"=w2103:errorcluster, "data"=w2087:sgl[], "Session out"=w2104:refnum<class "Session.lvclass">)  [unwired: 5 in, 1 out]
        n1901 = property on="Shutter模型输出结果 2" class="Arr (strict)"("Val(Sgnl)"=w2087) -> ()  [unwired: 2 in, 2 out]
        n1902 = Array Max & Min(array=w2087) -> (max index (indices)=w2091:i32)  [unwired: 3 out]
        n1903 = Delete From Array(array=w2092, length=1 ("长度"), index=0 ("索引")) -> (array with subset deleted=w2096:u8[])  [unwired: 1 out]
        n1904 = property on="dimension size" class="DigNum (strict)"() -> ("Value"=w2088:i32)  [unwired: 2 in, 2 out]
        n1905 = case "条件结构" shown="0, Default" w2091 {
          tunnel: ["No" "Yes"] -> w2089
          frame 0, Default {
          }
          frame 1 {
          }
        }
        n1906 = Build Array (concatenate)(w2096, w2091) -> (w2095:i32[])
        n1907 = Reshape Array(w2095, w2088) -> (w2090:i32[])
        n1908 = property on="记录Shutter模型的连续24个输出结果" class="Arr (strict)"("Val(Sgnl)"=w2090) -> ()  [unwired: 2 in, 2 out]
        n1909 = property on="Shutter模型输出结果" class="Str"("Val(Sgnl)"=w2089) -> ()  [unwired: 2 in, 2 out]
      }
    }
  }
  n1910 = while {
    tunnel: [w2116] -> w1
    tunnel: [w2115] -> w2
    tunnel: w11 -> [w2114]
    tunnel: w12 -> [w2113]
    tunnel: w13 -> [w2112]
    stop <- FALSE stop-if-true
    n1911 = property on="Tab Control" class="TabCtl (strict)"() -> ("Value"=w2111:T1)  [unwired: 2 in, 2 out]
    n1912 = case shown="\"Growth Temperature Initialization\", Default" w2111 {
      tunnel: [w2118 FALSE ("Value")] -> w2110
      frame "Growth Temperature Initialization", Default {
        n1913 = property on="Model switch" class="Bool (strict)"() -> ("Value"=w2118:bool)  [unwired: 2 in, 2 out]
      }
      frame "InAs/GaAs QDs on GaAs substrates" {
      }
    }
    n1914 = case shown="True" w2110 {
      tunnel: w2114 -> [_ w2142]
      tunnel: w2112 -> [w2121 w2141]
      tunnel: w2113 -> [w2120 w2140]
      tunnel: [w2121 w2139] -> w2115
      tunnel: [w2120 w2138] -> w2116
      frame False {
      }
      frame True {
        n1915 = property on="经过python转换后的数组" class="Arr (strict)"() -> ("Value"=w2133:dbl[][][][])  [unwired: 2 in, 2 out]
        n1916 = property on="记录Reconstruction模型的连续24个输出结果" class="Arr (strict)"() -> ("Value"=w2124:u8[])  [unwired: 2 in, 2 out]
        n1917 = Array Size(array=w2133) -> (size(s)=w2134:i32[])
        n1918 = Reshape Array(w2133, w2142) -> (w2132:dbl[])
        n1919 = call <vilib>:"Run_one_input_data.vi"("error in (no error)"=w2140, "data"=w2132, "shape"=w2134, "Session in"=w2141) -> ("error out"=w2137:errorcluster, "Session out"=w2136:refnum<class "Session.lvclass">)  [unwired: 5 in, 1 out]
        n1920 = call-poly <vilib>:"Get_result.vi"("error in (no error)"=w2137, "index"=0, "Session in"=w2136) -> ("error out"=w2138:errorcluster, "data"=w2122:sgl[], "Session out"=w2139:refnum<class "Session.lvclass">)  [unwired: 5 in, 1 out]
        n1921 = property on="Reconstruction模型输出结果" class="Arr (strict)"("Val(Sgnl)"=w2122) -> ()  [unwired: 2 in, 2 out]
        n1922 = Array Max & Min(array=w2122) -> (max index (indices)=w2127:i32)  [unwired: 3 out]
        n1923 = Delete From Array(array=w2124, length=1 ("长度"), index=0 ("索引")) -> (array with subset deleted=w2131:u8[])  [unwired: 1 out]
        n1924 = property on="dimension size" class="DigNum (strict)"() -> ("Value"=w2126:i32)  [unwired: 2 in, 2 out]
        n1925 = case "条件结构" shown="0, Default" w2127 {
          tunnel: ["As cap" "c(4×4)" "(2×4)" "Oxidation" "Deoxidation" "(n×6)"] -> w2125
          frame 0, Default {
          }
          frame 1 {
          }
          frame 2 {
          }
          frame 3 {
          }
          frame 4 {
          }
          frame 5 {
          }
        }
        n1926 = Build Array (concatenate)(w2131, w2127) -> (w2130:i32[])
        n1927 = Reshape Array(w2130, w2126) -> (w2123:i32[])
        n1928 = property on="记录Reconstruction模型的连续24个输出结果" class="Arr (strict)"("Val(Sgnl)"=w2123) -> ()  [unwired: 2 in, 2 out]
        n1929 = property on="Reconstruction模型输出结果" class="Str"("Val(Sgnl)"=w2125) -> ()  [unwired: 2 in, 2 out]
      }
    }
  }
  n1930 = VISA Close(VISA resource name=w76, error in (no error)=w77) -> (error out=w83:errorcluster)
  n1931 = call <vilib>:"Simple Error Handler.vi"("error in (no error)"=w83) -> ()  [unwired: 4 in, 5 out]
  n1932 = VISA Close(VISA resource name=w88, error in (no error)=w87) -> (error out=w86:errorcluster)
  n1933 = Close Python Session(session in=w50, error in=w49) -> ()  [unwired: 1 out]
  n1934 = call <vilib>:"Simple Error Handler.vi"("error in (no error)"=w86) -> ()  [unwired: 4 in, 5 out]
  n1935 = call <vilib>:"release.vi"("error in (no error)"=w26, "Session in"=w25) -> ()  [unwired: 9 in, 1 out]
  n1936 = call <vilib>:"release.vi"("error in (no error)"=w28, "Session in"=w27) -> ()  [unwired: 9 in, 1 out]
  n1937 = call <vilib>:"release.vi"("error in (no error)"=w1, "Session in"=w2) -> ()  [unwired: 9 in, 1 out]
  n1938 = VISA Close(VISA resource name=w51, error in (no error)=w52) -> ()  [unwired: 1 out]
